vi "Final_Phase C_GND.vi"() -> ()   [LabVIEW 2014]
uses:
  <vilib>/DAQmx/create/channels.llb/DAQmx Create Channel (CO-Pulse Generation-Frequency).vi
  <vilib>/DAQmx/configure/timing.llb/DAQmx Timing (Implicit).vi
  <vilib>/DAQmx/write.llb/DAQmx Write (Counter Frequency 1Chan 1Samp).vi
  <vilib>/DAQmx/create/channels.llb/DAQmx Create Channel (DO-Digital Output).vi
  <vilib>/DAQmx/write.llb/DAQmx Write (Digital Bool 1Line 1Point).vi
  <vilib>/express/express arith-compare/Formula/XNode/ExpressFormulaBlockNode.xnode
panel:
  in  "Duration":dbl
  out "SB Elapsed Time (s)":dbl caption="Elapsed Time (s)"
  in  "frequency":dbl=1.0 format="%_6g"
  in  "Resistor Values in Ohms":string(combo)
  out "resis bank Numeric":dbl
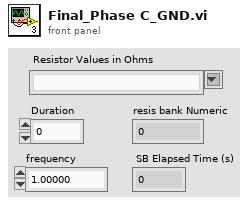
[diagram p1: front panel]
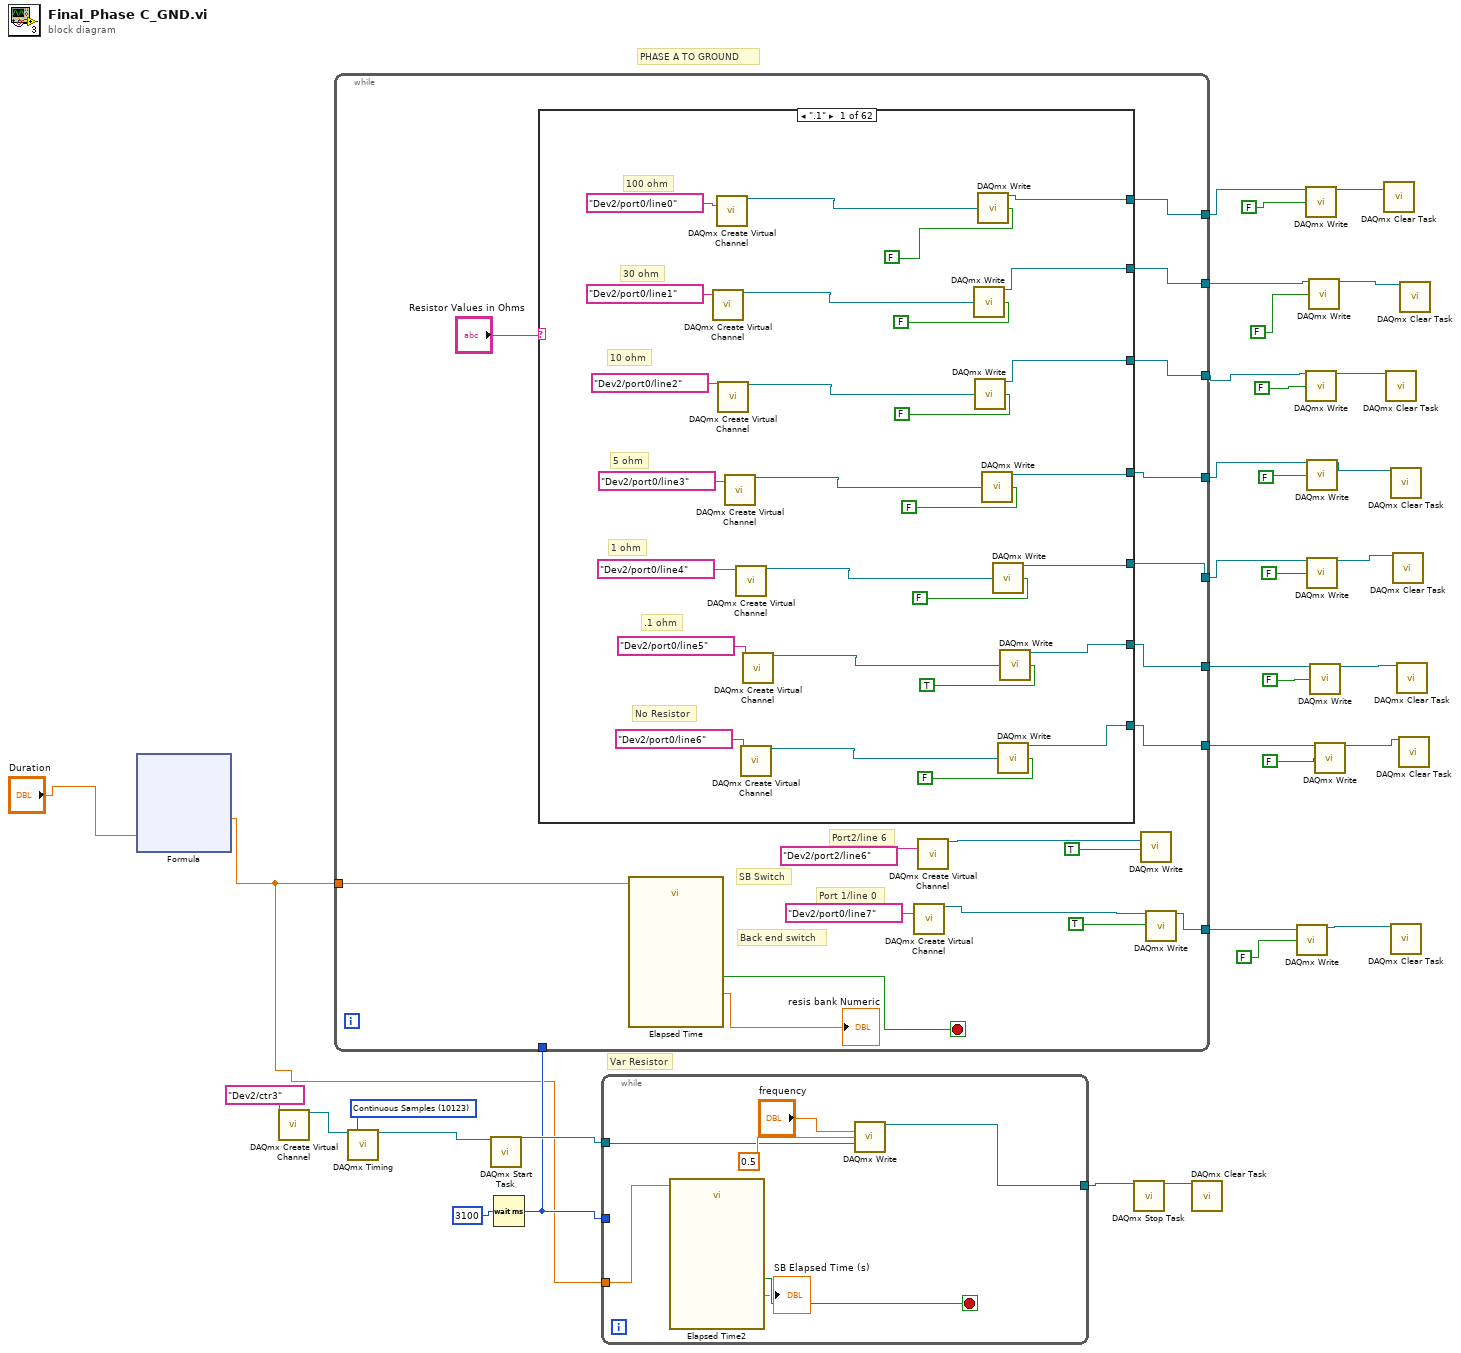
[diagram p0: block diagram]
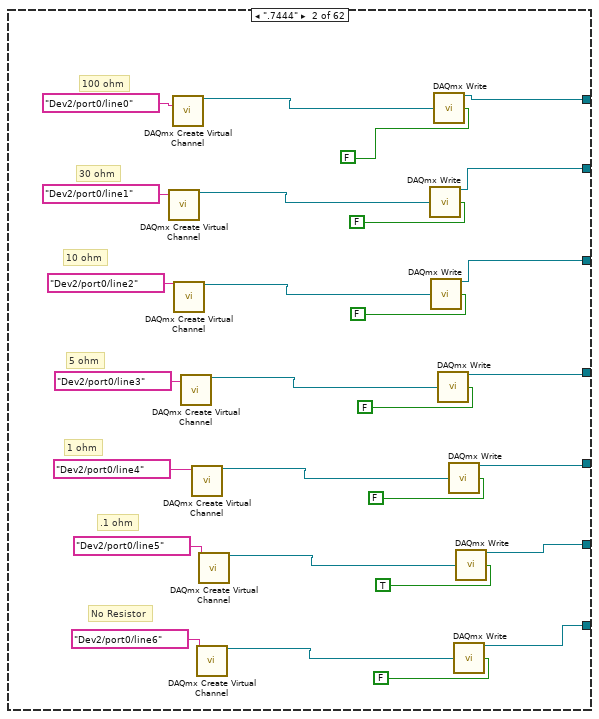
[diagram p2: hidden frame]
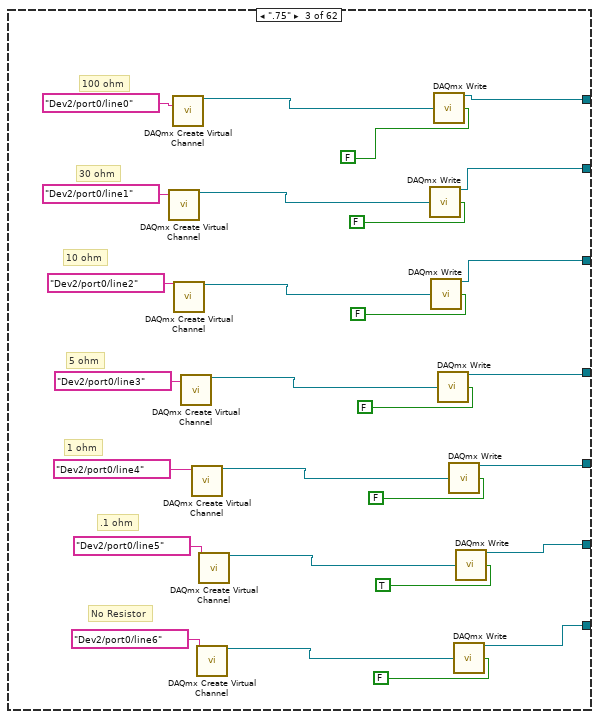
[diagram p3: hidden frame]
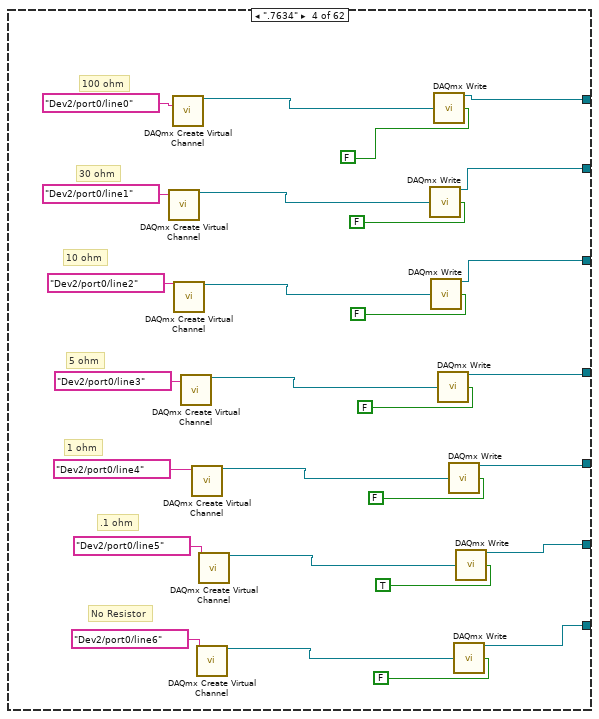
[diagram p4: hidden frame]
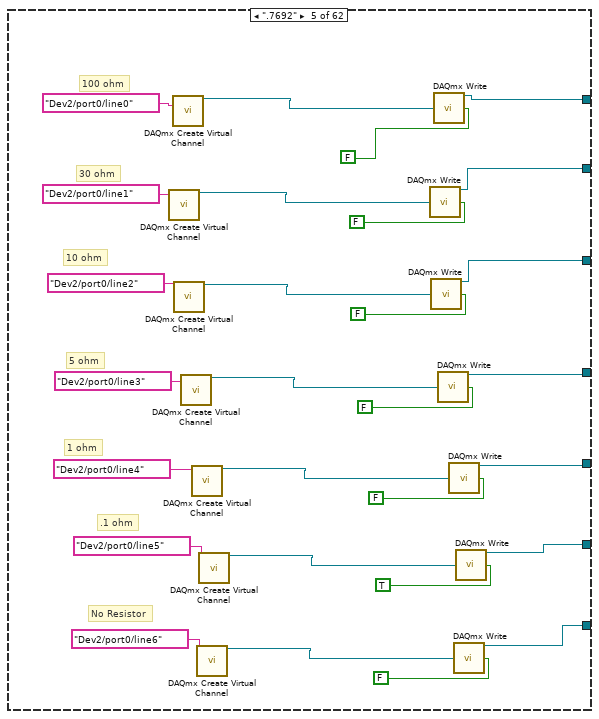
[diagram p5: hidden frame]
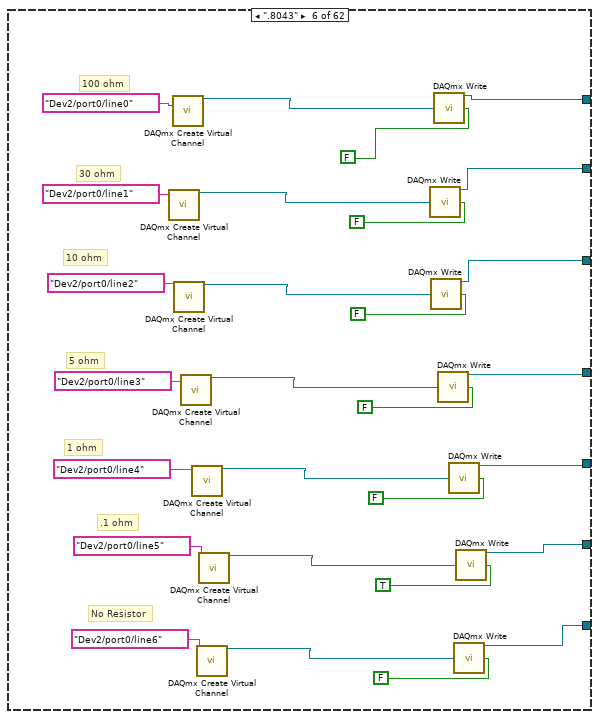
[diagram p6: hidden frame]
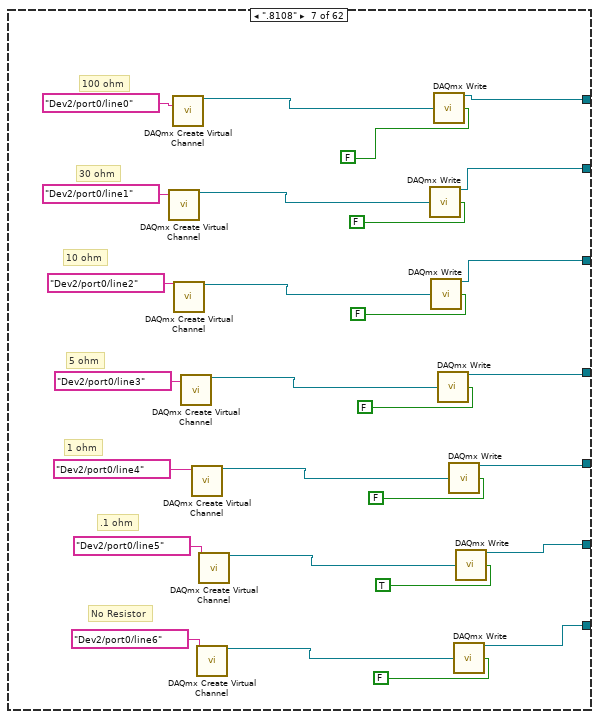
[diagram p7: hidden frame]
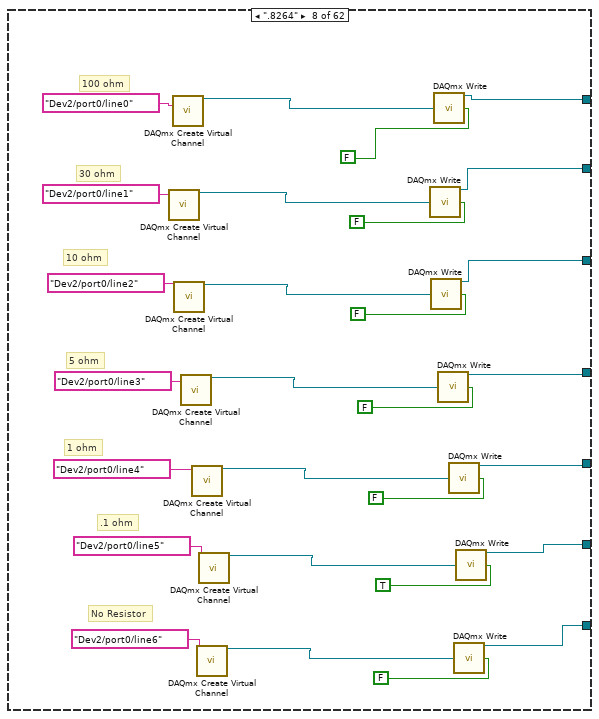
[diagram p8: hidden frame]
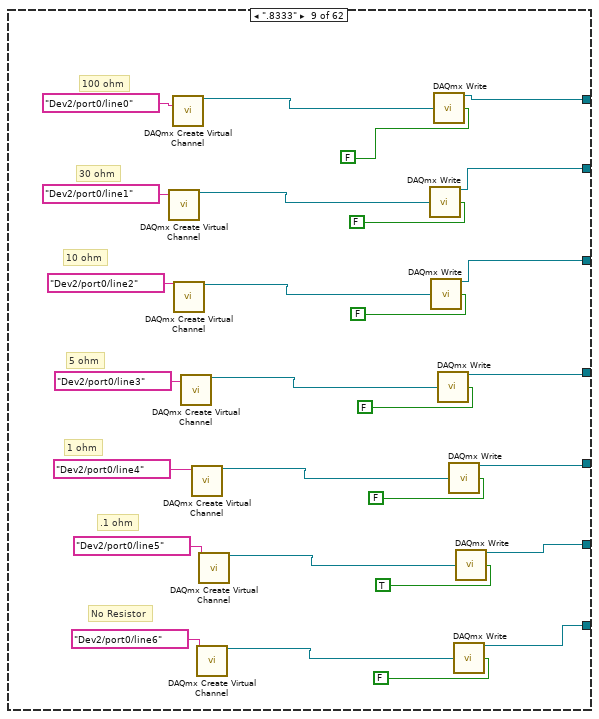
[diagram p9: hidden frame]
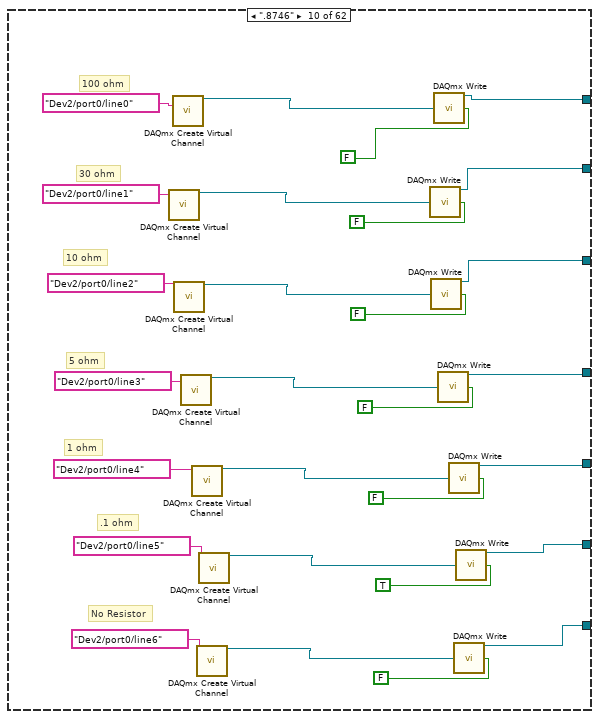
[diagram p10: hidden frame]
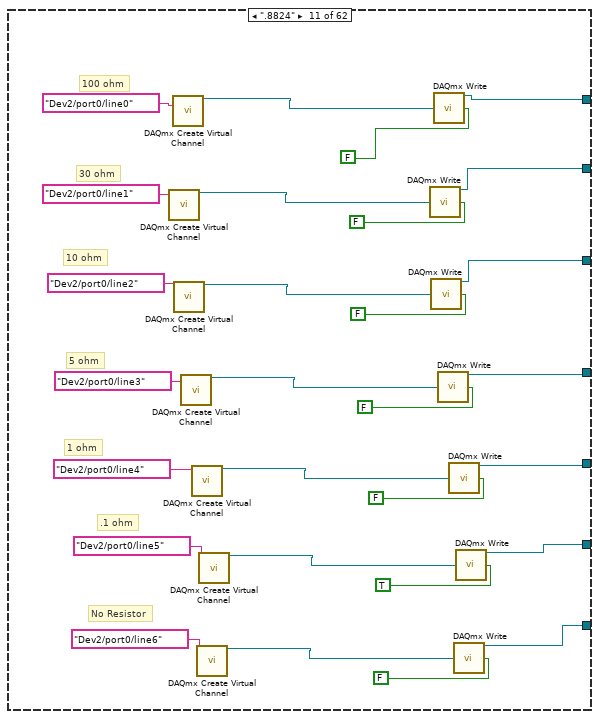
[diagram p11: hidden frame]
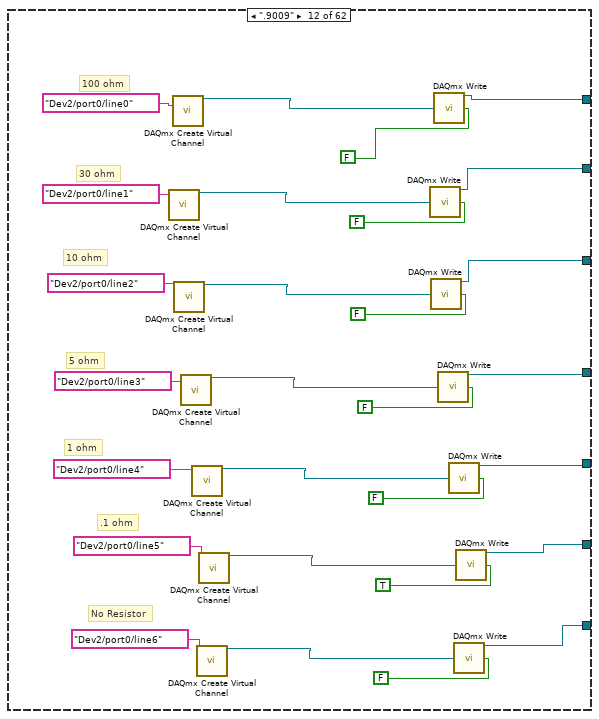
[diagram p12: hidden frame]
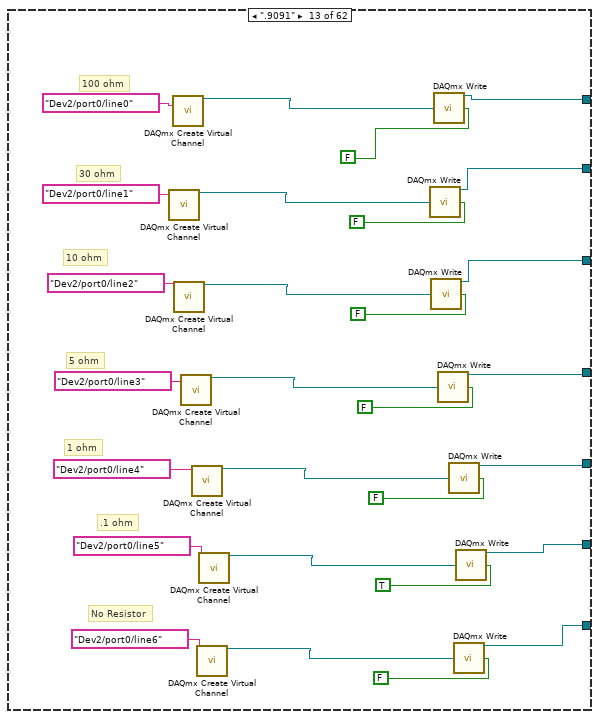
[diagram p13: hidden frame]
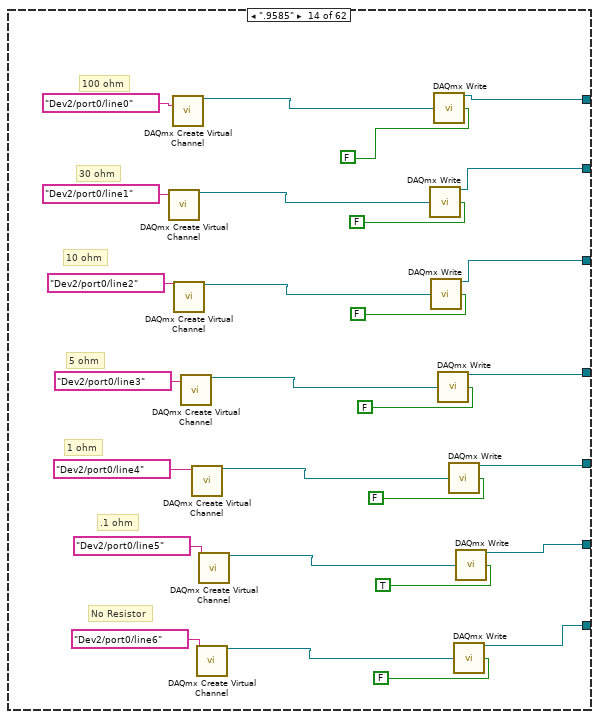
[diagram p14: hidden frame]
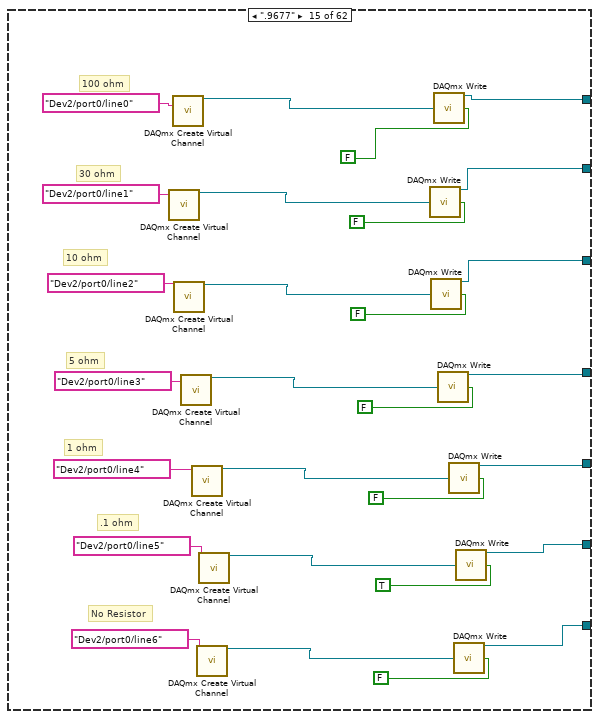
[diagram p15: hidden frame]
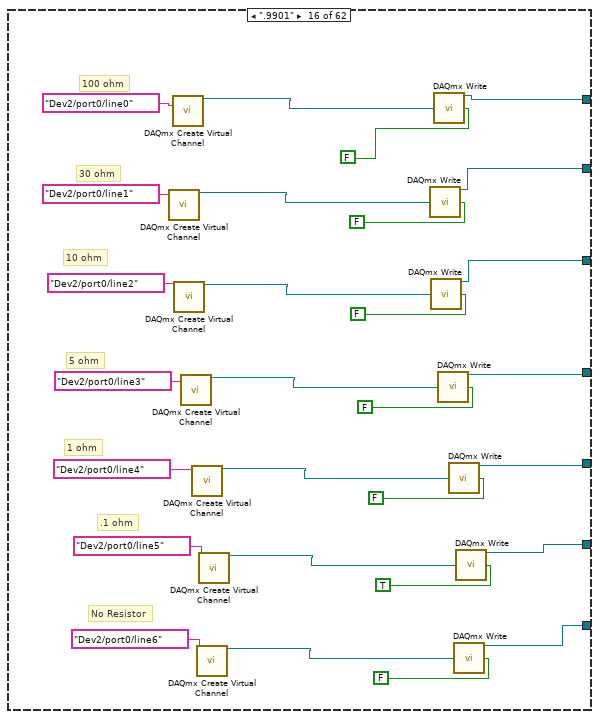
[diagram p16: hidden frame]
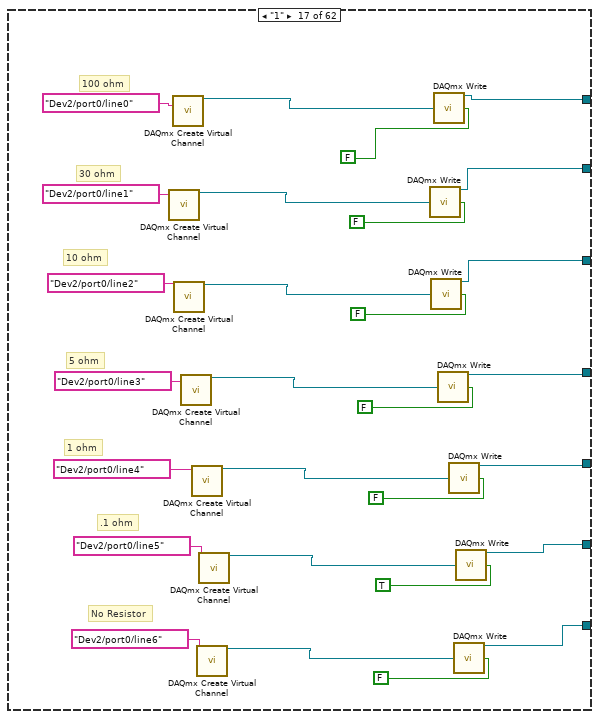
[diagram p17: hidden frame]
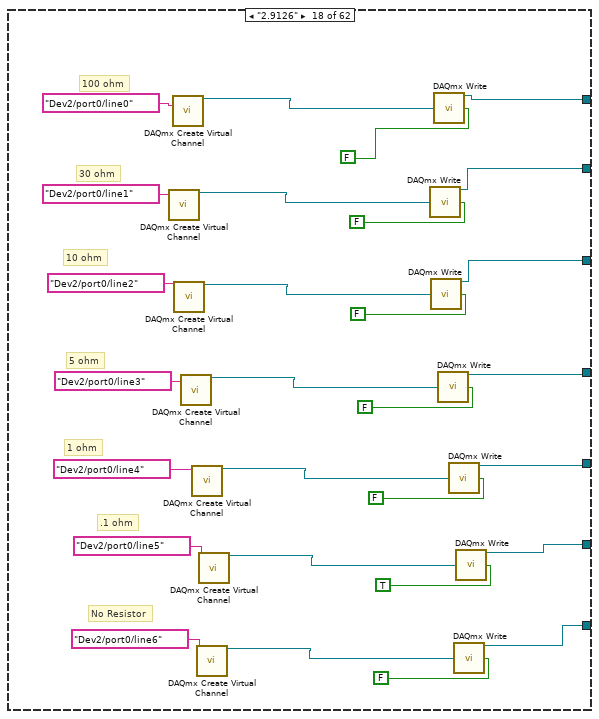
[diagram p18: hidden frame]
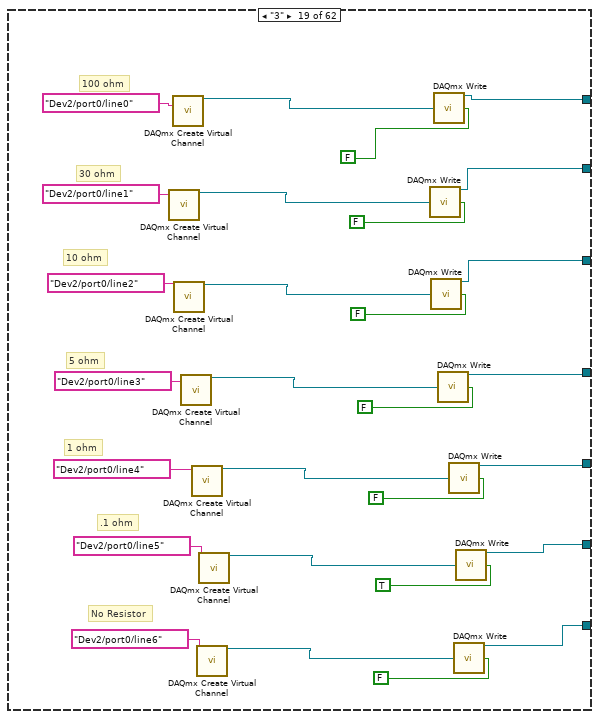
[diagram p19: hidden frame]
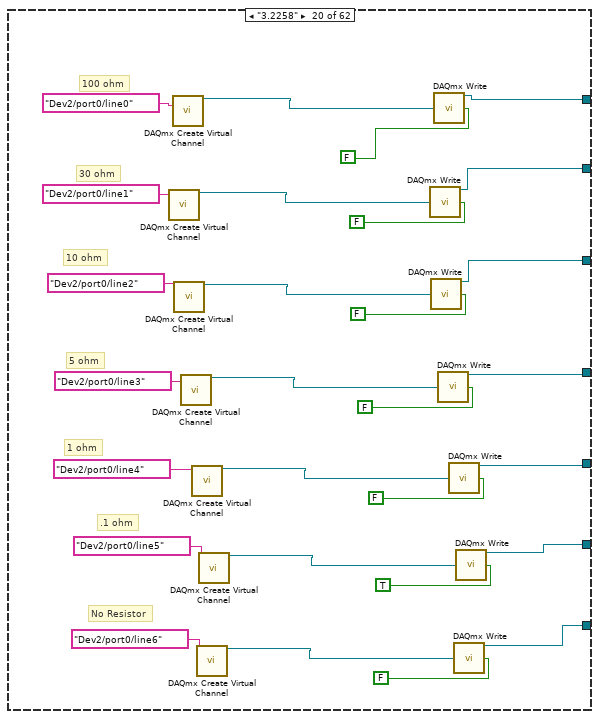
[diagram p20: hidden frame]
diagram:
  w7 = 10123 items=["Finite Samples"=10178, "Continuous Samples"=10123, "Hardware Timed Single Point"=12522] ("sample mode")
  # "Var Resistor"
  # "PHASE A TO GROUND"
  n1 = xnode "Formula"("X"="Duration") -> ("Result"=w4:dbl)  [unwired: 1 in, 1 out]
  n2 = call-poly <vilib>:"DAQmx Create Virtual Channel.vi"("counter"=tag "Dev2/ctr3" ("Counter(s)")) -> ("task out"=w8:refnum<k21>)  [unwired: 8 in, 6 out]
  n3 = call-poly <vilib>:"DAQmx Timing.vi"("task/channels in"=w8, "sample mode"=w7) -> ("task out"=w9:refnum<k21>)  [unwired: 3 in, 10 out]
  n4 = call <vilib>:"DAQmx Start Task.vi"("task/channels in"=w9) -> ("task out"=w6:refnum<k21>)  [unwired: 1 in, 13 out]
  n5 = Wait (ms)(milliseconds to wait=u32 3100) -> (millisecond timer value=w5:u32)
  n6 = while {
    tunnel: [w47] -> w12
    tunnel: [w46] -> w19
    tunnel: [w45] -> w18
    tunnel: [w44] -> w17
    tunnel: [w43] -> w16
    tunnel: [w42] -> w15
    tunnel: [w41] -> w14
    tunnel: [w40] -> w13
    tunnel: w5 -> [_]
    tunnel: w4 -> [w36]
    stop <- w37 stop-if-true
    # "Port 1/line 0"
    # "Port2/line 6"
    # "SB Switch"
    # "Back end switch"
    n7 = case shown="\".1\"" "Resistor Values in Ohms" {
      tunnel: [w63 w91 w119 w147 w175 w203 w231 w259 w287 w315 w343 w371 w399 w427 w455 w483 w511 w539 w567 w595 w623 w651 w679 w707 w735 w763 w791 w819 w847 w875 w903 w931 w959 w987 w1015 w1043 w1071 w1099 w1127 w1155 w1183 w1211 w1239 w1267 w1295 w1323 w1351 w1379 w1407 w1435 w1463 w1491 w1519 w1547 w1575 w1603 w1631 w1659 w1687 w1715 w1743 w1771] -> w46
      tunnel: [w62 w90 w118 w146 w174 w202 w230 w258 w286 w314 w342 w370 w398 w426 w454 w482 w510 w538 w566 w594 w622 w650 w678 w706 w734 w762 w790 w818 w846 w874 w902 w930 w958 w986 w1014 w1042 w1070 w1098 w1126 w1154 w1182 w1210 w1238 w1266 w1294 w1322 w1350 w1378 w1406 w1434 w1462 w1490 w1518 w1546 w1574 w1602 w1630 w1658 w1686 w1714 w1742 w1770] -> w45
      tunnel: [w60 w88 w116 w144 w172 w200 w228 w256 w284 w312 w340 w368 w396 w424 w452 w480 w508 w536 w564 w592 w620 w648 w676 w704 w732 w760 w788 w816 w844 w872 w900 w928 w956 w984 w1012 w1040 w1068 w1096 w1124 w1152 w1180 w1208 w1236 w1264 w1292 w1320 w1348 w1376 w1404 w1432 w1460 w1488 w1516 w1544 w1572 w1600 w1628 w1656 w1684 w1712 w1740 w1768] -> w43
      tunnel: [w59 w87 w115 w143 w171 w199 w227 w255 w283 w311 w339 w367 w395 w423 w451 w479 w507 w535 w563 w591 w619 w647 w675 w703 w731 w759 w787 w815 w843 w871 w899 w927 w955 w983 w1011 w1039 w1067 w1095 w1123 w1151 w1179 w1207 w1235 w1263 w1291 w1319 w1347 w1375 w1403 w1431 w1459 w1487 w1515 w1543 w1571 w1599 w1627 w1655 w1683 w1711 w1739 w1767] -> w42
      tunnel: [w58 w86 w114 w142 w170 w198 w226 w254 w282 w310 w338 w366 w394 w422 w450 w478 w506 w534 w562 w590 w618 w646 w674 w702 w730 w758 w786 w814 w842 w870 w898 w926 w954 w982 w1010 w1038 w1066 w1094 w1122 w1150 w1178 w1206 w1234 w1262 w1290 w1318 w1346 w1374 w1402 w1430 w1458 w1486 w1514 w1542 w1570 w1598 w1626 w1654 w1682 w1710 w1738 w1766] -> w41
      tunnel: [w54 w82 w110 w138 w166 w194 w222 w250 w278 w306 w334 w362 w390 w418 w446 w474 w502 w530 w558 w586 w614 w642 w670 w698 w726 w754 w782 w810 w838 w866 w894 w922 w950 w978 w1006 w1034 w1062 w1090 w1118 w1146 w1174 w1202 w1230 w1258 w1286 w1314 w1342 w1370 w1398 w1426 w1454 w1482 w1510 w1538 w1566 w1594 w1622 w1650 w1678 w1706 w1734 w1762] -> w40
      tunnel: [w61 w89 w117 w145 w173 w201 w229 w257 w285 w313 w341 w369 w397 w425 w453 w481 w509 w537 w565 w593 w621 w649 w677 w705 w733 w761 w789 w817 w845 w873 w901 w929 w957 w985 w1013 w1041 w1069 w1097 w1125 w1153 w1181 w1209 w1237 w1265 w1293 w1321 w1349 w1377 w1405 w1433 w1461 w1489 w1517 w1545 w1573 w1601 w1629 w1657 w1685 w1713 w1741 w1769] -> w44
      frame ".1" {
        # "No Resistor"
        # "30 ohm"
        # ".1 ohm"
        # "1 ohm"
        # "5 ohm"
        # "10 ohm"
        # "100 ohm"
        n8 = call-poly <vilib>:"DAQmx Create Virtual Channel.vi"("lines"=tag "Dev2/port0/line1") -> ("task out"=w68:refnum<k21>)  [unwired: 13 in, 1 out]
        n9 = call-poly <vilib>:"DAQmx Create Virtual Channel.vi"("lines"=tag "Dev2/port0/line0") -> ("task out"=w69:refnum<k21>)  [unwired: 13 in, 1 out]
        n10 = call-poly <vilib>:"DAQmx Create Virtual Channel.vi"("lines"=tag "Dev2/port0/line2") -> ("task out"=w67:refnum<k21>)  [unwired: 13 in, 1 out]
        n11 = call-poly <vilib>:"DAQmx Create Virtual Channel.vi"("lines"=tag "Dev2/port0/line3") -> ("task out"=w66:refnum<k21>)  [unwired: 13 in, 1 out]
        n12 = call-poly <vilib>:"DAQmx Create Virtual Channel.vi"("lines"=tag "Dev2/port0/line4") -> ("task out"=w65:refnum<k21>)  [unwired: 13 in, 1 out]
        n13 = call-poly <vilib>:"DAQmx Create Virtual Channel.vi"("lines"=tag "Dev2/port0/line6") -> ("task out"=w57:refnum<k21>)  [unwired: 13 in, 1 out]
        n14 = call-poly <vilib>:"DAQmx Create Virtual Channel.vi"("lines"=tag "Dev2/port0/line5") -> ("task out"=w64:refnum<k21>)  [unwired: 13 in, 1 out]
        n15 = call-poly <vilib>:"DAQmx Write.vi"("task/channels in"=w68, "data"=FALSE) -> ("task out"=w62:refnum<k21>)  [unwired: 11 in, 2 out]
        n16 = call-poly <vilib>:"DAQmx Write.vi"("task/channels in"=w67, "data"=FALSE) -> ("task out"=w61:refnum<k21>)  [unwired: 11 in, 2 out]
        n17 = call-poly <vilib>:"DAQmx Write.vi"("task/channels in"=w69, "data"=FALSE) -> ("task out"=w63:refnum<k21>)  [unwired: 11 in, 2 out]
        n18 = call-poly <vilib>:"DAQmx Write.vi"("task/channels in"=w66, "data"=FALSE) -> ("task out"=w60:refnum<k21>)  [unwired: 11 in, 2 out]
        n19 = call-poly <vilib>:"DAQmx Write.vi"("task/channels in"=w65, "data"=FALSE) -> ("task out"=w59:refnum<k21>)  [unwired: 11 in, 2 out]
        n20 = call-poly <vilib>:"DAQmx Write.vi"("task/channels in"=w57, "data"=FALSE) -> ("task out"=w54:refnum<k21>)  [unwired: 11 in, 2 out]
        n21 = call-poly <vilib>:"DAQmx Write.vi"("task/channels in"=w64, "data"=TRUE) -> ("task out"=w58:refnum<k21>)  [unwired: 11 in, 2 out]
      }
      frame ".7444" {
        # "No Resistor"
        # "30 ohm"
        # ".1 ohm"
        # "1 ohm"
        # "5 ohm"
        # "10 ohm"
        # "100 ohm"
        n22 = call-poly <vilib>:"DAQmx Create Virtual Channel.vi"("lines"=tag "Dev2/port0/line1") -> ("task out"=w96:refnum<k21>)  [unwired: 13 in, 1 out]
        n23 = call-poly <vilib>:"DAQmx Create Virtual Channel.vi"("lines"=tag "Dev2/port0/line0") -> ("task out"=w97:refnum<k21>)  [unwired: 13 in, 1 out]
        n24 = call-poly <vilib>:"DAQmx Create Virtual Channel.vi"("lines"=tag "Dev2/port0/line2") -> ("task out"=w95:refnum<k21>)  [unwired: 13 in, 1 out]
        n25 = call-poly <vilib>:"DAQmx Create Virtual Channel.vi"("lines"=tag "Dev2/port0/line3") -> ("task out"=w94:refnum<k21>)  [unwired: 13 in, 1 out]
        n26 = call-poly <vilib>:"DAQmx Create Virtual Channel.vi"("lines"=tag "Dev2/port0/line4") -> ("task out"=w93:refnum<k21>)  [unwired: 13 in, 1 out]
        n27 = call-poly <vilib>:"DAQmx Create Virtual Channel.vi"("lines"=tag "Dev2/port0/line6") -> ("task out"=w85:refnum<k21>)  [unwired: 13 in, 1 out]
        n28 = call-poly <vilib>:"DAQmx Create Virtual Channel.vi"("lines"=tag "Dev2/port0/line5") -> ("task out"=w92:refnum<k21>)  [unwired: 13 in, 1 out]
        n29 = call-poly <vilib>:"DAQmx Write.vi"("task/channels in"=w96, "data"=FALSE) -> ("task out"=w90:refnum<k21>)  [unwired: 11 in, 2 out]
        n30 = call-poly <vilib>:"DAQmx Write.vi"("task/channels in"=w95, "data"=FALSE) -> ("task out"=w89:refnum<k21>)  [unwired: 11 in, 2 out]
        n31 = call-poly <vilib>:"DAQmx Write.vi"("task/channels in"=w97, "data"=FALSE) -> ("task out"=w91:refnum<k21>)  [unwired: 11 in, 2 out]
        n32 = call-poly <vilib>:"DAQmx Write.vi"("task/channels in"=w94, "data"=FALSE) -> ("task out"=w88:refnum<k21>)  [unwired: 11 in, 2 out]
        n33 = call-poly <vilib>:"DAQmx Write.vi"("task/channels in"=w93, "data"=FALSE) -> ("task out"=w87:refnum<k21>)  [unwired: 11 in, 2 out]
        n34 = call-poly <vilib>:"DAQmx Write.vi"("task/channels in"=w85, "data"=FALSE) -> ("task out"=w82:refnum<k21>)  [unwired: 11 in, 2 out]
        n35 = call-poly <vilib>:"DAQmx Write.vi"("task/channels in"=w92, "data"=TRUE) -> ("task out"=w86:refnum<k21>)  [unwired: 11 in, 2 out]
      }
      frame ".75" {
        # "No Resistor"
        # "30 ohm"
        # ".1 ohm"
        # "1 ohm"
        # "5 ohm"
        # "10 ohm"
        # "100 ohm"
        n36 = call-poly <vilib>:"DAQmx Create Virtual Channel.vi"("lines"=tag "Dev2/port0/line1") -> ("task out"=w124:refnum<k21>)  [unwired: 13 in, 1 out]
        n37 = call-poly <vilib>:"DAQmx Create Virtual Channel.vi"("lines"=tag "Dev2/port0/line0") -> ("task out"=w125:refnum<k21>)  [unwired: 13 in, 1 out]
        n38 = call-poly <vilib>:"DAQmx Create Virtual Channel.vi"("lines"=tag "Dev2/port0/line2") -> ("task out"=w123:refnum<k21>)  [unwired: 13 in, 1 out]
        n39 = call-poly <vilib>:"DAQmx Create Virtual Channel.vi"("lines"=tag "Dev2/port0/line3") -> ("task out"=w122:refnum<k21>)  [unwired: 13 in, 1 out]
        n40 = call-poly <vilib>:"DAQmx Create Virtual Channel.vi"("lines"=tag "Dev2/port0/line4") -> ("task out"=w121:refnum<k21>)  [unwired: 13 in, 1 out]
        n41 = call-poly <vilib>:"DAQmx Create Virtual Channel.vi"("lines"=tag "Dev2/port0/line6") -> ("task out"=w113:refnum<k21>)  [unwired: 13 in, 1 out]
        n42 = call-poly <vilib>:"DAQmx Create Virtual Channel.vi"("lines"=tag "Dev2/port0/line5") -> ("task out"=w120:refnum<k21>)  [unwired: 13 in, 1 out]
        n43 = call-poly <vilib>:"DAQmx Write.vi"("task/channels in"=w124, "data"=FALSE) -> ("task out"=w118:refnum<k21>)  [unwired: 11 in, 2 out]
        n44 = call-poly <vilib>:"DAQmx Write.vi"("task/channels in"=w123, "data"=FALSE) -> ("task out"=w117:refnum<k21>)  [unwired: 11 in, 2 out]
        n45 = call-poly <vilib>:"DAQmx Write.vi"("task/channels in"=w125, "data"=FALSE) -> ("task out"=w119:refnum<k21>)  [unwired: 11 in, 2 out]
        n46 = call-poly <vilib>:"DAQmx Write.vi"("task/channels in"=w122, "data"=FALSE) -> ("task out"=w116:refnum<k21>)  [unwired: 11 in, 2 out]
        n47 = call-poly <vilib>:"DAQmx Write.vi"("task/channels in"=w121, "data"=FALSE) -> ("task out"=w115:refnum<k21>)  [unwired: 11 in, 2 out]
        n48 = call-poly <vilib>:"DAQmx Write.vi"("task/channels in"=w113, "data"=FALSE) -> ("task out"=w110:refnum<k21>)  [unwired: 11 in, 2 out]
        n49 = call-poly <vilib>:"DAQmx Write.vi"("task/channels in"=w120, "data"=TRUE) -> ("task out"=w114:refnum<k21>)  [unwired: 11 in, 2 out]
      }
      frame ".7634" {
        # "No Resistor"
        # "30 ohm"
        # ".1 ohm"
        # "1 ohm"
        # "5 ohm"
        # "10 ohm"
        # "100 ohm"
        n50 = call-poly <vilib>:"DAQmx Create Virtual Channel.vi"("lines"=tag "Dev2/port0/line1") -> ("task out"=w152:refnum<k21>)  [unwired: 13 in, 1 out]
        n51 = call-poly <vilib>:"DAQmx Create Virtual Channel.vi"("lines"=tag "Dev2/port0/line0") -> ("task out"=w153:refnum<k21>)  [unwired: 13 in, 1 out]
        n52 = call-poly <vilib>:"DAQmx Create Virtual Channel.vi"("lines"=tag "Dev2/port0/line2") -> ("task out"=w151:refnum<k21>)  [unwired: 13 in, 1 out]
        n53 = call-poly <vilib>:"DAQmx Create Virtual Channel.vi"("lines"=tag "Dev2/port0/line3") -> ("task out"=w150:refnum<k21>)  [unwired: 13 in, 1 out]
        n54 = call-poly <vilib>:"DAQmx Create Virtual Channel.vi"("lines"=tag "Dev2/port0/line4") -> ("task out"=w149:refnum<k21>)  [unwired: 13 in, 1 out]
        n55 = call-poly <vilib>:"DAQmx Create Virtual Channel.vi"("lines"=tag "Dev2/port0/line6") -> ("task out"=w141:refnum<k21>)  [unwired: 13 in, 1 out]
        n56 = call-poly <vilib>:"DAQmx Create Virtual Channel.vi"("lines"=tag "Dev2/port0/line5") -> ("task out"=w148:refnum<k21>)  [unwired: 13 in, 1 out]
        n57 = call-poly <vilib>:"DAQmx Write.vi"("task/channels in"=w152, "data"=FALSE) -> ("task out"=w146:refnum<k21>)  [unwired: 11 in, 2 out]
        n58 = call-poly <vilib>:"DAQmx Write.vi"("task/channels in"=w151, "data"=FALSE) -> ("task out"=w145:refnum<k21>)  [unwired: 11 in, 2 out]
        n59 = call-poly <vilib>:"DAQmx Write.vi"("task/channels in"=w153, "data"=FALSE) -> ("task out"=w147:refnum<k21>)  [unwired: 11 in, 2 out]
        n60 = call-poly <vilib>:"DAQmx Write.vi"("task/channels in"=w150, "data"=FALSE) -> ("task out"=w144:refnum<k21>)  [unwired: 11 in, 2 out]
        n61 = call-poly <vilib>:"DAQmx Write.vi"("task/channels in"=w149, "data"=FALSE) -> ("task out"=w143:refnum<k21>)  [unwired: 11 in, 2 out]
        n62 = call-poly <vilib>:"DAQmx Write.vi"("task/channels in"=w141, "data"=FALSE) -> ("task out"=w138:refnum<k21>)  [unwired: 11 in, 2 out]
        n63 = call-poly <vilib>:"DAQmx Write.vi"("task/channels in"=w148, "data"=TRUE) -> ("task out"=w142:refnum<k21>)  [unwired: 11 in, 2 out]
      }
      frame ".7692" {
        # "No Resistor"
        # "30 ohm"
        # ".1 ohm"
        # "1 ohm"
        # "5 ohm"
        # "10 ohm"
        # "100 ohm"
        n64 = call-poly <vilib>:"DAQmx Create Virtual Channel.vi"("lines"=tag "Dev2/port0/line1") -> ("task out"=w180:refnum<k21>)  [unwired: 13 in, 1 out]
        n65 = call-poly <vilib>:"DAQmx Create Virtual Channel.vi"("lines"=tag "Dev2/port0/line0") -> ("task out"=w181:refnum<k21>)  [unwired: 13 in, 1 out]
        n66 = call-poly <vilib>:"DAQmx Create Virtual Channel.vi"("lines"=tag "Dev2/port0/line2") -> ("task out"=w179:refnum<k21>)  [unwired: 13 in, 1 out]
        n67 = call-poly <vilib>:"DAQmx Create Virtual Channel.vi"("lines"=tag "Dev2/port0/line3") -> ("task out"=w178:refnum<k21>)  [unwired: 13 in, 1 out]
        n68 = call-poly <vilib>:"DAQmx Create Virtual Channel.vi"("lines"=tag "Dev2/port0/line4") -> ("task out"=w177:refnum<k21>)  [unwired: 13 in, 1 out]
        n69 = call-poly <vilib>:"DAQmx Create Virtual Channel.vi"("lines"=tag "Dev2/port0/line6") -> ("task out"=w169:refnum<k21>)  [unwired: 13 in, 1 out]
        n70 = call-poly <vilib>:"DAQmx Create Virtual Channel.vi"("lines"=tag "Dev2/port0/line5") -> ("task out"=w176:refnum<k21>)  [unwired: 13 in, 1 out]
        n71 = call-poly <vilib>:"DAQmx Write.vi"("task/channels in"=w180, "data"=FALSE) -> ("task out"=w174:refnum<k21>)  [unwired: 11 in, 2 out]
        n72 = call-poly <vilib>:"DAQmx Write.vi"("task/channels in"=w179, "data"=FALSE) -> ("task out"=w173:refnum<k21>)  [unwired: 11 in, 2 out]
        n73 = call-poly <vilib>:"DAQmx Write.vi"("task/channels in"=w181, "data"=FALSE) -> ("task out"=w175:refnum<k21>)  [unwired: 11 in, 2 out]
        n74 = call-poly <vilib>:"DAQmx Write.vi"("task/channels in"=w178, "data"=FALSE) -> ("task out"=w172:refnum<k21>)  [unwired: 11 in, 2 out]
        n75 = call-poly <vilib>:"DAQmx Write.vi"("task/channels in"=w177, "data"=FALSE) -> ("task out"=w171:refnum<k21>)  [unwired: 11 in, 2 out]
        n76 = call-poly <vilib>:"DAQmx Write.vi"("task/channels in"=w169, "data"=FALSE) -> ("task out"=w166:refnum<k21>)  [unwired: 11 in, 2 out]
        n77 = call-poly <vilib>:"DAQmx Write.vi"("task/channels in"=w176, "data"=TRUE) -> ("task out"=w170:refnum<k21>)  [unwired: 11 in, 2 out]
      }
      frame ".8043" {
        # "No Resistor"
        # "30 ohm"
        # ".1 ohm"
        # "1 ohm"
        # "5 ohm"
        # "10 ohm"
        # "100 ohm"
        n78 = call-poly <vilib>:"DAQmx Create Virtual Channel.vi"("lines"=tag "Dev2/port0/line1") -> ("task out"=w208:refnum<k21>)  [unwired: 13 in, 1 out]
        n79 = call-poly <vilib>:"DAQmx Create Virtual Channel.vi"("lines"=tag "Dev2/port0/line0") -> ("task out"=w209:refnum<k21>)  [unwired: 13 in, 1 out]
        n80 = call-poly <vilib>:"DAQmx Create Virtual Channel.vi"("lines"=tag "Dev2/port0/line2") -> ("task out"=w207:refnum<k21>)  [unwired: 13 in, 1 out]
        n81 = call-poly <vilib>:"DAQmx Create Virtual Channel.vi"("lines"=tag "Dev2/port0/line3") -> ("task out"=w206:refnum<k21>)  [unwired: 13 in, 1 out]
        n82 = call-poly <vilib>:"DAQmx Create Virtual Channel.vi"("lines"=tag "Dev2/port0/line4") -> ("task out"=w205:refnum<k21>)  [unwired: 13 in, 1 out]
        n83 = call-poly <vilib>:"DAQmx Create Virtual Channel.vi"("lines"=tag "Dev2/port0/line6") -> ("task out"=w197:refnum<k21>)  [unwired: 13 in, 1 out]
        n84 = call-poly <vilib>:"DAQmx Create Virtual Channel.vi"("lines"=tag "Dev2/port0/line5") -> ("task out"=w204:refnum<k21>)  [unwired: 13 in, 1 out]
        n85 = call-poly <vilib>:"DAQmx Write.vi"("task/channels in"=w208, "data"=FALSE) -> ("task out"=w202:refnum<k21>)  [unwired: 11 in, 2 out]
        n86 = call-poly <vilib>:"DAQmx Write.vi"("task/channels in"=w207, "data"=FALSE) -> ("task out"=w201:refnum<k21>)  [unwired: 11 in, 2 out]
        n87 = call-poly <vilib>:"DAQmx Write.vi"("task/channels in"=w209, "data"=FALSE) -> ("task out"=w203:refnum<k21>)  [unwired: 11 in, 2 out]
        n88 = call-poly <vilib>:"DAQmx Write.vi"("task/channels in"=w206, "data"=FALSE) -> ("task out"=w200:refnum<k21>)  [unwired: 11 in, 2 out]
        n89 = call-poly <vilib>:"DAQmx Write.vi"("task/channels in"=w205, "data"=FALSE) -> ("task out"=w199:refnum<k21>)  [unwired: 11 in, 2 out]
        n90 = call-poly <vilib>:"DAQmx Write.vi"("task/channels in"=w197, "data"=FALSE) -> ("task out"=w194:refnum<k21>)  [unwired: 11 in, 2 out]
        n91 = call-poly <vilib>:"DAQmx Write.vi"("task/channels in"=w204, "data"=TRUE) -> ("task out"=w198:refnum<k21>)  [unwired: 11 in, 2 out]
      }
      frame ".8108" {
        # "No Resistor"
        # "30 ohm"
        # ".1 ohm"
        # "1 ohm"
        # "5 ohm"
        # "10 ohm"
        # "100 ohm"
        n92 = call-poly <vilib>:"DAQmx Create Virtual Channel.vi"("lines"=tag "Dev2/port0/line1") -> ("task out"=w236:refnum<k21>)  [unwired: 13 in, 1 out]
        n93 = call-poly <vilib>:"DAQmx Create Virtual Channel.vi"("lines"=tag "Dev2/port0/line0") -> ("task out"=w237:refnum<k21>)  [unwired: 13 in, 1 out]
        n94 = call-poly <vilib>:"DAQmx Create Virtual Channel.vi"("lines"=tag "Dev2/port0/line2") -> ("task out"=w235:refnum<k21>)  [unwired: 13 in, 1 out]
        n95 = call-poly <vilib>:"DAQmx Create Virtual Channel.vi"("lines"=tag "Dev2/port0/line3") -> ("task out"=w234:refnum<k21>)  [unwired: 13 in, 1 out]
        n96 = call-poly <vilib>:"DAQmx Create Virtual Channel.vi"("lines"=tag "Dev2/port0/line4") -> ("task out"=w233:refnum<k21>)  [unwired: 13 in, 1 out]
        n97 = call-poly <vilib>:"DAQmx Create Virtual Channel.vi"("lines"=tag "Dev2/port0/line6") -> ("task out"=w225:refnum<k21>)  [unwired: 13 in, 1 out]
        n98 = call-poly <vilib>:"DAQmx Create Virtual Channel.vi"("lines"=tag "Dev2/port0/line5") -> ("task out"=w232:refnum<k21>)  [unwired: 13 in, 1 out]
        n99 = call-poly <vilib>:"DAQmx Write.vi"("task/channels in"=w236, "data"=FALSE) -> ("task out"=w230:refnum<k21>)  [unwired: 11 in, 2 out]
        n100 = call-poly <vilib>:"DAQmx Write.vi"("task/channels in"=w235, "data"=FALSE) -> ("task out"=w229:refnum<k21>)  [unwired: 11 in, 2 out]
        n101 = call-poly <vilib>:"DAQmx Write.vi"("task/channels in"=w237, "data"=FALSE) -> ("task out"=w231:refnum<k21>)  [unwired: 11 in, 2 out]
        n102 = call-poly <vilib>:"DAQmx Write.vi"("task/channels in"=w234, "data"=FALSE) -> ("task out"=w228:refnum<k21>)  [unwired: 11 in, 2 out]
        n103 = call-poly <vilib>:"DAQmx Write.vi"("task/channels in"=w233, "data"=FALSE) -> ("task out"=w227:refnum<k21>)  [unwired: 11 in, 2 out]
        n104 = call-poly <vilib>:"DAQmx Write.vi"("task/channels in"=w225, "data"=FALSE) -> ("task out"=w222:refnum<k21>)  [unwired: 11 in, 2 out]
        n105 = call-poly <vilib>:"DAQmx Write.vi"("task/channels in"=w232, "data"=TRUE) -> ("task out"=w226:refnum<k21>)  [unwired: 11 in, 2 out]
      }
      frame ".8264" {
        # "No Resistor"
        # "30 ohm"
        # ".1 ohm"
        # "1 ohm"
        # "5 ohm"
        # "10 ohm"
        # "100 ohm"
        n106 = call-poly <vilib>:"DAQmx Create Virtual Channel.vi"("lines"=tag "Dev2/port0/line1") -> ("task out"=w264:refnum<k21>)  [unwired: 13 in, 1 out]
        n107 = call-poly <vilib>:"DAQmx Create Virtual Channel.vi"("lines"=tag "Dev2/port0/line0") -> ("task out"=w265:refnum<k21>)  [unwired: 13 in, 1 out]
        n108 = call-poly <vilib>:"DAQmx Create Virtual Channel.vi"("lines"=tag "Dev2/port0/line2") -> ("task out"=w263:refnum<k21>)  [unwired: 13 in, 1 out]
        n109 = call-poly <vilib>:"DAQmx Create Virtual Channel.vi"("lines"=tag "Dev2/port0/line3") -> ("task out"=w262:refnum<k21>)  [unwired: 13 in, 1 out]
        n110 = call-poly <vilib>:"DAQmx Create Virtual Channel.vi"("lines"=tag "Dev2/port0/line4") -> ("task out"=w261:refnum<k21>)  [unwired: 13 in, 1 out]
        n111 = call-poly <vilib>:"DAQmx Create Virtual Channel.vi"("lines"=tag "Dev2/port0/line6") -> ("task out"=w253:refnum<k21>)  [unwired: 13 in, 1 out]
        n112 = call-poly <vilib>:"DAQmx Create Virtual Channel.vi"("lines"=tag "Dev2/port0/line5") -> ("task out"=w260:refnum<k21>)  [unwired: 13 in, 1 out]
        n113 = call-poly <vilib>:"DAQmx Write.vi"("task/channels in"=w264, "data"=FALSE) -> ("task out"=w258:refnum<k21>)  [unwired: 11 in, 2 out]
        n114 = call-poly <vilib>:"DAQmx Write.vi"("task/channels in"=w263, "data"=FALSE) -> ("task out"=w257:refnum<k21>)  [unwired: 11 in, 2 out]
        n115 = call-poly <vilib>:"DAQmx Write.vi"("task/channels in"=w265, "data"=FALSE) -> ("task out"=w259:refnum<k21>)  [unwired: 11 in, 2 out]
        n116 = call-poly <vilib>:"DAQmx Write.vi"("task/channels in"=w262, "data"=FALSE) -> ("task out"=w256:refnum<k21>)  [unwired: 11 in, 2 out]
        n117 = call-poly <vilib>:"DAQmx Write.vi"("task/channels in"=w261, "data"=FALSE) -> ("task out"=w255:refnum<k21>)  [unwired: 11 in, 2 out]
        n118 = call-poly <vilib>:"DAQmx Write.vi"("task/channels in"=w253, "data"=FALSE) -> ("task out"=w250:refnum<k21>)  [unwired: 11 in, 2 out]
        n119 = call-poly <vilib>:"DAQmx Write.vi"("task/channels in"=w260, "data"=TRUE) -> ("task out"=w254:refnum<k21>)  [unwired: 11 in, 2 out]
      }
      frame ".8333" {
        # "No Resistor"
        # "30 ohm"
        # ".1 ohm"
        # "1 ohm"
        # "5 ohm"
        # "10 ohm"
        # "100 ohm"
        n120 = call-poly <vilib>:"DAQmx Create Virtual Channel.vi"("lines"=tag "Dev2/port0/line1") -> ("task out"=w292:refnum<k21>)  [unwired: 13 in, 1 out]
        n121 = call-poly <vilib>:"DAQmx Create Virtual Channel.vi"("lines"=tag "Dev2/port0/line0") -> ("task out"=w293:refnum<k21>)  [unwired: 13 in, 1 out]
        n122 = call-poly <vilib>:"DAQmx Create Virtual Channel.vi"("lines"=tag "Dev2/port0/line2") -> ("task out"=w291:refnum<k21>)  [unwired: 13 in, 1 out]
        n123 = call-poly <vilib>:"DAQmx Create Virtual Channel.vi"("lines"=tag "Dev2/port0/line3") -> ("task out"=w290:refnum<k21>)  [unwired: 13 in, 1 out]
        n124 = call-poly <vilib>:"DAQmx Create Virtual Channel.vi"("lines"=tag "Dev2/port0/line4") -> ("task out"=w289:refnum<k21>)  [unwired: 13 in, 1 out]
        n125 = call-poly <vilib>:"DAQmx Create Virtual Channel.vi"("lines"=tag "Dev2/port0/line6") -> ("task out"=w281:refnum<k21>)  [unwired: 13 in, 1 out]
        n126 = call-poly <vilib>:"DAQmx Create Virtual Channel.vi"("lines"=tag "Dev2/port0/line5") -> ("task out"=w288:refnum<k21>)  [unwired: 13 in, 1 out]
        n127 = call-poly <vilib>:"DAQmx Write.vi"("task/channels in"=w292, "data"=FALSE) -> ("task out"=w286:refnum<k21>)  [unwired: 11 in, 2 out]
        n128 = call-poly <vilib>:"DAQmx Write.vi"("task/channels in"=w291, "data"=FALSE) -> ("task out"=w285:refnum<k21>)  [unwired: 11 in, 2 out]
        n129 = call-poly <vilib>:"DAQmx Write.vi"("task/channels in"=w293, "data"=FALSE) -> ("task out"=w287:refnum<k21>)  [unwired: 11 in, 2 out]
        n130 = call-poly <vilib>:"DAQmx Write.vi"("task/channels in"=w290, "data"=FALSE) -> ("task out"=w284:refnum<k21>)  [unwired: 11 in, 2 out]
        n131 = call-poly <vilib>:"DAQmx Write.vi"("task/channels in"=w289, "data"=FALSE) -> ("task out"=w283:refnum<k21>)  [unwired: 11 in, 2 out]
        n132 = call-poly <vilib>:"DAQmx Write.vi"("task/channels in"=w281, "data"=FALSE) -> ("task out"=w278:refnum<k21>)  [unwired: 11 in, 2 out]
        n133 = call-poly <vilib>:"DAQmx Write.vi"("task/channels in"=w288, "data"=TRUE) -> ("task out"=w282:refnum<k21>)  [unwired: 11 in, 2 out]
      }
      frame ".8746" {
        # "No Resistor"
        # "30 ohm"
        # ".1 ohm"
        # "1 ohm"
        # "5 ohm"
        # "10 ohm"
        # "100 ohm"
        n134 = call-poly <vilib>:"DAQmx Create Virtual Channel.vi"("lines"=tag "Dev2/port0/line1") -> ("task out"=w320:refnum<k21>)  [unwired: 13 in, 1 out]
        n135 = call-poly <vilib>:"DAQmx Create Virtual Channel.vi"("lines"=tag "Dev2/port0/line0") -> ("task out"=w321:refnum<k21>)  [unwired: 13 in, 1 out]
        n136 = call-poly <vilib>:"DAQmx Create Virtual Channel.vi"("lines"=tag "Dev2/port0/line2") -> ("task out"=w319:refnum<k21>)  [unwired: 13 in, 1 out]
        n137 = call-poly <vilib>:"DAQmx Create Virtual Channel.vi"("lines"=tag "Dev2/port0/line3") -> ("task out"=w318:refnum<k21>)  [unwired: 13 in, 1 out]
        n138 = call-poly <vilib>:"DAQmx Create Virtual Channel.vi"("lines"=tag "Dev2/port0/line4") -> ("task out"=w317:refnum<k21>)  [unwired: 13 in, 1 out]
        n139 = call-poly <vilib>:"DAQmx Create Virtual Channel.vi"("lines"=tag "Dev2/port0/line6") -> ("task out"=w309:refnum<k21>)  [unwired: 13 in, 1 out]
        n140 = call-poly <vilib>:"DAQmx Create Virtual Channel.vi"("lines"=tag "Dev2/port0/line5") -> ("task out"=w316:refnum<k21>)  [unwired: 13 in, 1 out]
        n141 = call-poly <vilib>:"DAQmx Write.vi"("task/channels in"=w320, "data"=FALSE) -> ("task out"=w314:refnum<k21>)  [unwired: 11 in, 2 out]
        n142 = call-poly <vilib>:"DAQmx Write.vi"("task/channels in"=w319, "data"=FALSE) -> ("task out"=w313:refnum<k21>)  [unwired: 11 in, 2 out]
        n143 = call-poly <vilib>:"DAQmx Write.vi"("task/channels in"=w321, "data"=FALSE) -> ("task out"=w315:refnum<k21>)  [unwired: 11 in, 2 out]
        n144 = call-poly <vilib>:"DAQmx Write.vi"("task/channels in"=w318, "data"=FALSE) -> ("task out"=w312:refnum<k21>)  [unwired: 11 in, 2 out]
        n145 = call-poly <vilib>:"DAQmx Write.vi"("task/channels in"=w317, "data"=FALSE) -> ("task out"=w311:refnum<k21>)  [unwired: 11 in, 2 out]
        n146 = call-poly <vilib>:"DAQmx Write.vi"("task/channels in"=w309, "data"=FALSE) -> ("task out"=w306:refnum<k21>)  [unwired: 11 in, 2 out]
        n147 = call-poly <vilib>:"DAQmx Write.vi"("task/channels in"=w316, "data"=TRUE) -> ("task out"=w310:refnum<k21>)  [unwired: 11 in, 2 out]
      }
      frame ".8824" {
        # "No Resistor"
        # "30 ohm"
        # ".1 ohm"
        # "1 ohm"
        # "5 ohm"
        # "10 ohm"
        # "100 ohm"
        n148 = call-poly <vilib>:"DAQmx Create Virtual Channel.vi"("lines"=tag "Dev2/port0/line1") -> ("task out"=w348:refnum<k21>)  [unwired: 13 in, 1 out]
        n149 = call-poly <vilib>:"DAQmx Create Virtual Channel.vi"("lines"=tag "Dev2/port0/line0") -> ("task out"=w349:refnum<k21>)  [unwired: 13 in, 1 out]
        n150 = call-poly <vilib>:"DAQmx Create Virtual Channel.vi"("lines"=tag "Dev2/port0/line2") -> ("task out"=w347:refnum<k21>)  [unwired: 13 in, 1 out]
        n151 = call-poly <vilib>:"DAQmx Create Virtual Channel.vi"("lines"=tag "Dev2/port0/line3") -> ("task out"=w346:refnum<k21>)  [unwired: 13 in, 1 out]
        n152 = call-poly <vilib>:"DAQmx Create Virtual Channel.vi"("lines"=tag "Dev2/port0/line4") -> ("task out"=w345:refnum<k21>)  [unwired: 13 in, 1 out]
        n153 = call-poly <vilib>:"DAQmx Create Virtual Channel.vi"("lines"=tag "Dev2/port0/line6") -> ("task out"=w337:refnum<k21>)  [unwired: 13 in, 1 out]
        n154 = call-poly <vilib>:"DAQmx Create Virtual Channel.vi"("lines"=tag "Dev2/port0/line5") -> ("task out"=w344:refnum<k21>)  [unwired: 13 in, 1 out]
        n155 = call-poly <vilib>:"DAQmx Write.vi"("task/channels in"=w348, "data"=FALSE) -> ("task out"=w342:refnum<k21>)  [unwired: 11 in, 2 out]
        n156 = call-poly <vilib>:"DAQmx Write.vi"("task/channels in"=w347, "data"=FALSE) -> ("task out"=w341:refnum<k21>)  [unwired: 11 in, 2 out]
        n157 = call-poly <vilib>:"DAQmx Write.vi"("task/channels in"=w349, "data"=FALSE) -> ("task out"=w343:refnum<k21>)  [unwired: 11 in, 2 out]
        n158 = call-poly <vilib>:"DAQmx Write.vi"("task/channels in"=w346, "data"=FALSE) -> ("task out"=w340:refnum<k21>)  [unwired: 11 in, 2 out]
        n159 = call-poly <vilib>:"DAQmx Write.vi"("task/channels in"=w345, "data"=FALSE) -> ("task out"=w339:refnum<k21>)  [unwired: 11 in, 2 out]
        n160 = call-poly <vilib>:"DAQmx Write.vi"("task/channels in"=w337, "data"=FALSE) -> ("task out"=w334:refnum<k21>)  [unwired: 11 in, 2 out]
        n161 = call-poly <vilib>:"DAQmx Write.vi"("task/channels in"=w344, "data"=TRUE) -> ("task out"=w338:refnum<k21>)  [unwired: 11 in, 2 out]
      }
      frame ".9009" {
        # "No Resistor"
        # "30 ohm"
        # ".1 ohm"
        # "1 ohm"
        # "5 ohm"
        # "10 ohm"
        # "100 ohm"
        n162 = call-poly <vilib>:"DAQmx Create Virtual Channel.vi"("lines"=tag "Dev2/port0/line1") -> ("task out"=w376:refnum<k21>)  [unwired: 13 in, 1 out]
        n163 = call-poly <vilib>:"DAQmx Create Virtual Channel.vi"("lines"=tag "Dev2/port0/line0") -> ("task out"=w377:refnum<k21>)  [unwired: 13 in, 1 out]
        n164 = call-poly <vilib>:"DAQmx Create Virtual Channel.vi"("lines"=tag "Dev2/port0/line2") -> ("task out"=w375:refnum<k21>)  [unwired: 13 in, 1 out]
        n165 = call-poly <vilib>:"DAQmx Create Virtual Channel.vi"("lines"=tag "Dev2/port0/line3") -> ("task out"=w374:refnum<k21>)  [unwired: 13 in, 1 out]
        n166 = call-poly <vilib>:"DAQmx Create Virtual Channel.vi"("lines"=tag "Dev2/port0/line4") -> ("task out"=w373:refnum<k21>)  [unwired: 13 in, 1 out]
        n167 = call-poly <vilib>:"DAQmx Create Virtual Channel.vi"("lines"=tag "Dev2/port0/line6") -> ("task out"=w365:refnum<k21>)  [unwired: 13 in, 1 out]
        n168 = call-poly <vilib>:"DAQmx Create Virtual Channel.vi"("lines"=tag "Dev2/port0/line5") -> ("task out"=w372:refnum<k21>)  [unwired: 13 in, 1 out]
        n169 = call-poly <vilib>:"DAQmx Write.vi"("task/channels in"=w376, "data"=FALSE) -> ("task out"=w370:refnum<k21>)  [unwired: 11 in, 2 out]
        n170 = call-poly <vilib>:"DAQmx Write.vi"("task/channels in"=w375, "data"=FALSE) -> ("task out"=w369:refnum<k21>)  [unwired: 11 in, 2 out]
        n171 = call-poly <vilib>:"DAQmx Write.vi"("task/channels in"=w377, "data"=FALSE) -> ("task out"=w371:refnum<k21>)  [unwired: 11 in, 2 out]
        n172 = call-poly <vilib>:"DAQmx Write.vi"("task/channels in"=w374, "data"=FALSE) -> ("task out"=w368:refnum<k21>)  [unwired: 11 in, 2 out]
        n173 = call-poly <vilib>:"DAQmx Write.vi"("task/channels in"=w373, "data"=FALSE) -> ("task out"=w367:refnum<k21>)  [unwired: 11 in, 2 out]
        n174 = call-poly <vilib>:"DAQmx Write.vi"("task/channels in"=w365, "data"=FALSE) -> ("task out"=w362:refnum<k21>)  [unwired: 11 in, 2 out]
        n175 = call-poly <vilib>:"DAQmx Write.vi"("task/channels in"=w372, "data"=TRUE) -> ("task out"=w366:refnum<k21>)  [unwired: 11 in, 2 out]
      }
      frame ".9091" {
        # "No Resistor"
        # "30 ohm"
        # ".1 ohm"
        # "1 ohm"
        # "5 ohm"
        # "10 ohm"
        # "100 ohm"
        n176 = call-poly <vilib>:"DAQmx Create Virtual Channel.vi"("lines"=tag "Dev2/port0/line1") -> ("task out"=w404:refnum<k21>)  [unwired: 13 in, 1 out]
        n177 = call-poly <vilib>:"DAQmx Create Virtual Channel.vi"("lines"=tag "Dev2/port0/line0") -> ("task out"=w405:refnum<k21>)  [unwired: 13 in, 1 out]
        n178 = call-poly <vilib>:"DAQmx Create Virtual Channel.vi"("lines"=tag "Dev2/port0/line2") -> ("task out"=w403:refnum<k21>)  [unwired: 13 in, 1 out]
        n179 = call-poly <vilib>:"DAQmx Create Virtual Channel.vi"("lines"=tag "Dev2/port0/line3") -> ("task out"=w402:refnum<k21>)  [unwired: 13 in, 1 out]
        n180 = call-poly <vilib>:"DAQmx Create Virtual Channel.vi"("lines"=tag "Dev2/port0/line4") -> ("task out"=w401:refnum<k21>)  [unwired: 13 in, 1 out]
        n181 = call-poly <vilib>:"DAQmx Create Virtual Channel.vi"("lines"=tag "Dev2/port0/line6") -> ("task out"=w393:refnum<k21>)  [unwired: 13 in, 1 out]
        n182 = call-poly <vilib>:"DAQmx Create Virtual Channel.vi"("lines"=tag "Dev2/port0/line5") -> ("task out"=w400:refnum<k21>)  [unwired: 13 in, 1 out]
        n183 = call-poly <vilib>:"DAQmx Write.vi"("task/channels in"=w404, "data"=FALSE) -> ("task out"=w398:refnum<k21>)  [unwired: 11 in, 2 out]
        n184 = call-poly <vilib>:"DAQmx Write.vi"("task/channels in"=w403, "data"=FALSE) -> ("task out"=w397:refnum<k21>)  [unwired: 11 in, 2 out]
        n185 = call-poly <vilib>:"DAQmx Write.vi"("task/channels in"=w405, "data"=FALSE) -> ("task out"=w399:refnum<k21>)  [unwired: 11 in, 2 out]
        n186 = call-poly <vilib>:"DAQmx Write.vi"("task/channels in"=w402, "data"=FALSE) -> ("task out"=w396:refnum<k21>)  [unwired: 11 in, 2 out]
        n187 = call-poly <vilib>:"DAQmx Write.vi"("task/channels in"=w401, "data"=FALSE) -> ("task out"=w395:refnum<k21>)  [unwired: 11 in, 2 out]
        n188 = call-poly <vilib>:"DAQmx Write.vi"("task/channels in"=w393, "data"=FALSE) -> ("task out"=w390:refnum<k21>)  [unwired: 11 in, 2 out]
        n189 = call-poly <vilib>:"DAQmx Write.vi"("task/channels in"=w400, "data"=TRUE) -> ("task out"=w394:refnum<k21>)  [unwired: 11 in, 2 out]
      }
      frame ".9585" {
        # "No Resistor"
        # "30 ohm"
        # ".1 ohm"
        # "1 ohm"
        # "5 ohm"
        # "10 ohm"
        # "100 ohm"
        n190 = call-poly <vilib>:"DAQmx Create Virtual Channel.vi"("lines"=tag "Dev2/port0/line1") -> ("task out"=w432:refnum<k21>)  [unwired: 13 in, 1 out]
        n191 = call-poly <vilib>:"DAQmx Create Virtual Channel.vi"("lines"=tag "Dev2/port0/line0") -> ("task out"=w433:refnum<k21>)  [unwired: 13 in, 1 out]
        n192 = call-poly <vilib>:"DAQmx Create Virtual Channel.vi"("lines"=tag "Dev2/port0/line2") -> ("task out"=w431:refnum<k21>)  [unwired: 13 in, 1 out]
        n193 = call-poly <vilib>:"DAQmx Create Virtual Channel.vi"("lines"=tag "Dev2/port0/line3") -> ("task out"=w430:refnum<k21>)  [unwired: 13 in, 1 out]
        n194 = call-poly <vilib>:"DAQmx Create Virtual Channel.vi"("lines"=tag "Dev2/port0/line4") -> ("task out"=w429:refnum<k21>)  [unwired: 13 in, 1 out]
        n195 = call-poly <vilib>:"DAQmx Create Virtual Channel.vi"("lines"=tag "Dev2/port0/line6") -> ("task out"=w421:refnum<k21>)  [unwired: 13 in, 1 out]
        n196 = call-poly <vilib>:"DAQmx Create Virtual Channel.vi"("lines"=tag "Dev2/port0/line5") -> ("task out"=w428:refnum<k21>)  [unwired: 13 in, 1 out]
        n197 = call-poly <vilib>:"DAQmx Write.vi"("task/channels in"=w432, "data"=FALSE) -> ("task out"=w426:refnum<k21>)  [unwired: 11 in, 2 out]
        n198 = call-poly <vilib>:"DAQmx Write.vi"("task/channels in"=w431, "data"=FALSE) -> ("task out"=w425:refnum<k21>)  [unwired: 11 in, 2 out]
        n199 = call-poly <vilib>:"DAQmx Write.vi"("task/channels in"=w433, "data"=FALSE) -> ("task out"=w427:refnum<k21>)  [unwired: 11 in, 2 out]
        n200 = call-poly <vilib>:"DAQmx Write.vi"("task/channels in"=w430, "data"=FALSE) -> ("task out"=w424:refnum<k21>)  [unwired: 11 in, 2 out]
        n201 = call-poly <vilib>:"DAQmx Write.vi"("task/channels in"=w429, "data"=FALSE) -> ("task out"=w423:refnum<k21>)  [unwired: 11 in, 2 out]
        n202 = call-poly <vilib>:"DAQmx Write.vi"("task/channels in"=w421, "data"=FALSE) -> ("task out"=w418:refnum<k21>)  [unwired: 11 in, 2 out]
        n203 = call-poly <vilib>:"DAQmx Write.vi"("task/channels in"=w428, "data"=TRUE) -> ("task out"=w422:refnum<k21>)  [unwired: 11 in, 2 out]
      }
      frame ".9677" {
        # "No Resistor"
        # "30 ohm"
        # ".1 ohm"
        # "1 ohm"
        # "5 ohm"
        # "10 ohm"
        # "100 ohm"
        n204 = call-poly <vilib>:"DAQmx Create Virtual Channel.vi"("lines"=tag "Dev2/port0/line1") -> ("task out"=w460:refnum<k21>)  [unwired: 13 in, 1 out]
        n205 = call-poly <vilib>:"DAQmx Create Virtual Channel.vi"("lines"=tag "Dev2/port0/line0") -> ("task out"=w461:refnum<k21>)  [unwired: 13 in, 1 out]
        n206 = call-poly <vilib>:"DAQmx Create Virtual Channel.vi"("lines"=tag "Dev2/port0/line2") -> ("task out"=w459:refnum<k21>)  [unwired: 13 in, 1 out]
        n207 = call-poly <vilib>:"DAQmx Create Virtual Channel.vi"("lines"=tag "Dev2/port0/line3") -> ("task out"=w458:refnum<k21>)  [unwired: 13 in, 1 out]
        n208 = call-poly <vilib>:"DAQmx Create Virtual Channel.vi"("lines"=tag "Dev2/port0/line4") -> ("task out"=w457:refnum<k21>)  [unwired: 13 in, 1 out]
        n209 = call-poly <vilib>:"DAQmx Create Virtual Channel.vi"("lines"=tag "Dev2/port0/line6") -> ("task out"=w449:refnum<k21>)  [unwired: 13 in, 1 out]
        n210 = call-poly <vilib>:"DAQmx Create Virtual Channel.vi"("lines"=tag "Dev2/port0/line5") -> ("task out"=w456:refnum<k21>)  [unwired: 13 in, 1 out]
        n211 = call-poly <vilib>:"DAQmx Write.vi"("task/channels in"=w460, "data"=FALSE) -> ("task out"=w454:refnum<k21>)  [unwired: 11 in, 2 out]
        n212 = call-poly <vilib>:"DAQmx Write.vi"("task/channels in"=w459, "data"=FALSE) -> ("task out"=w453:refnum<k21>)  [unwired: 11 in, 2 out]
        n213 = call-poly <vilib>:"DAQmx Write.vi"("task/channels in"=w461, "data"=FALSE) -> ("task out"=w455:refnum<k21>)  [unwired: 11 in, 2 out]
        n214 = call-poly <vilib>:"DAQmx Write.vi"("task/channels in"=w458, "data"=FALSE) -> ("task out"=w452:refnum<k21>)  [unwired: 11 in, 2 out]
        n215 = call-poly <vilib>:"DAQmx Write.vi"("task/channels in"=w457, "data"=FALSE) -> ("task out"=w451:refnum<k21>)  [unwired: 11 in, 2 out]
        n216 = call-poly <vilib>:"DAQmx Write.vi"("task/channels in"=w449, "data"=FALSE) -> ("task out"=w446:refnum<k21>)  [unwired: 11 in, 2 out]
        n217 = call-poly <vilib>:"DAQmx Write.vi"("task/channels in"=w456, "data"=TRUE) -> ("task out"=w450:refnum<k21>)  [unwired: 11 in, 2 out]
      }
      frame ".9901" {
        # "No Resistor"
        # "30 ohm"
        # ".1 ohm"
        # "1 ohm"
        # "5 ohm"
        # "10 ohm"
        # "100 ohm"
        n218 = call-poly <vilib>:"DAQmx Create Virtual Channel.vi"("lines"=tag "Dev2/port0/line1") -> ("task out"=w488:refnum<k21>)  [unwired: 13 in, 1 out]
        n219 = call-poly <vilib>:"DAQmx Create Virtual Channel.vi"("lines"=tag "Dev2/port0/line0") -> ("task out"=w489:refnum<k21>)  [unwired: 13 in, 1 out]
        n220 = call-poly <vilib>:"DAQmx Create Virtual Channel.vi"("lines"=tag "Dev2/port0/line2") -> ("task out"=w487:refnum<k21>)  [unwired: 13 in, 1 out]
        n221 = call-poly <vilib>:"DAQmx Create Virtual Channel.vi"("lines"=tag "Dev2/port0/line3") -> ("task out"=w486:refnum<k21>)  [unwired: 13 in, 1 out]
        n222 = call-poly <vilib>:"DAQmx Create Virtual Channel.vi"("lines"=tag "Dev2/port0/line4") -> ("task out"=w485:refnum<k21>)  [unwired: 13 in, 1 out]
        n223 = call-poly <vilib>:"DAQmx Create Virtual Channel.vi"("lines"=tag "Dev2/port0/line6") -> ("task out"=w477:refnum<k21>)  [unwired: 13 in, 1 out]
        n224 = call-poly <vilib>:"DAQmx Create Virtual Channel.vi"("lines"=tag "Dev2/port0/line5") -> ("task out"=w484:refnum<k21>)  [unwired: 13 in, 1 out]
        n225 = call-poly <vilib>:"DAQmx Write.vi"("task/channels in"=w488, "data"=FALSE) -> ("task out"=w482:refnum<k21>)  [unwired: 11 in, 2 out]
        n226 = call-poly <vilib>:"DAQmx Write.vi"("task/channels in"=w487, "data"=FALSE) -> ("task out"=w481:refnum<k21>)  [unwired: 11 in, 2 out]
        n227 = call-poly <vilib>:"DAQmx Write.vi"("task/channels in"=w489, "data"=FALSE) -> ("task out"=w483:refnum<k21>)  [unwired: 11 in, 2 out]
        n228 = call-poly <vilib>:"DAQmx Write.vi"("task/channels in"=w486, "data"=FALSE) -> ("task out"=w480:refnum<k21>)  [unwired: 11 in, 2 out]
        n229 = call-poly <vilib>:"DAQmx Write.vi"("task/channels in"=w485, "data"=FALSE) -> ("task out"=w479:refnum<k21>)  [unwired: 11 in, 2 out]
        n230 = call-poly <vilib>:"DAQmx Write.vi"("task/channels in"=w477, "data"=FALSE) -> ("task out"=w474:refnum<k21>)  [unwired: 11 in, 2 out]
        n231 = call-poly <vilib>:"DAQmx Write.vi"("task/channels in"=w484, "data"=TRUE) -> ("task out"=w478:refnum<k21>)  [unwired: 11 in, 2 out]
      }
      frame "1" {
        # "No Resistor"
        # "30 ohm"
        # ".1 ohm"
        # "1 ohm"
        # "5 ohm"
        # "10 ohm"
        # "100 ohm"
        n232 = call-poly <vilib>:"DAQmx Create Virtual Channel.vi"("lines"=tag "Dev2/port0/line1") -> ("task out"=w516:refnum<k21>)  [unwired: 13 in, 1 out]
        n233 = call-poly <vilib>:"DAQmx Create Virtual Channel.vi"("lines"=tag "Dev2/port0/line0") -> ("task out"=w517:refnum<k21>)  [unwired: 13 in, 1 out]
        n234 = call-poly <vilib>:"DAQmx Create Virtual Channel.vi"("lines"=tag "Dev2/port0/line2") -> ("task out"=w515:refnum<k21>)  [unwired: 13 in, 1 out]
        n235 = call-poly <vilib>:"DAQmx Create Virtual Channel.vi"("lines"=tag "Dev2/port0/line3") -> ("task out"=w514:refnum<k21>)  [unwired: 13 in, 1 out]
        n236 = call-poly <vilib>:"DAQmx Create Virtual Channel.vi"("lines"=tag "Dev2/port0/line4") -> ("task out"=w513:refnum<k21>)  [unwired: 13 in, 1 out]
        n237 = call-poly <vilib>:"DAQmx Create Virtual Channel.vi"("lines"=tag "Dev2/port0/line6") -> ("task out"=w505:refnum<k21>)  [unwired: 13 in, 1 out]
        n238 = call-poly <vilib>:"DAQmx Create Virtual Channel.vi"("lines"=tag "Dev2/port0/line5") -> ("task out"=w512:refnum<k21>)  [unwired: 13 in, 1 out]
        n239 = call-poly <vilib>:"DAQmx Write.vi"("task/channels in"=w516, "data"=FALSE) -> ("task out"=w510:refnum<k21>)  [unwired: 11 in, 2 out]
        n240 = call-poly <vilib>:"DAQmx Write.vi"("task/channels in"=w515, "data"=FALSE) -> ("task out"=w509:refnum<k21>)  [unwired: 11 in, 2 out]
        n241 = call-poly <vilib>:"DAQmx Write.vi"("task/channels in"=w517, "data"=FALSE) -> ("task out"=w511:refnum<k21>)  [unwired: 11 in, 2 out]
        n242 = call-poly <vilib>:"DAQmx Write.vi"("task/channels in"=w514, "data"=FALSE) -> ("task out"=w508:refnum<k21>)  [unwired: 11 in, 2 out]
        n243 = call-poly <vilib>:"DAQmx Write.vi"("task/channels in"=w513, "data"=FALSE) -> ("task out"=w507:refnum<k21>)  [unwired: 11 in, 2 out]
        n244 = call-poly <vilib>:"DAQmx Write.vi"("task/channels in"=w505, "data"=FALSE) -> ("task out"=w502:refnum<k21>)  [unwired: 11 in, 2 out]
        n245 = call-poly <vilib>:"DAQmx Write.vi"("task/channels in"=w512, "data"=TRUE) -> ("task out"=w506:refnum<k21>)  [unwired: 11 in, 2 out]
      }
      frame "2.9126" {
        # "No Resistor"
        # "30 ohm"
        # ".1 ohm"
        # "1 ohm"
        # "5 ohm"
        # "10 ohm"
        # "100 ohm"
        n246 = call-poly <vilib>:"DAQmx Create Virtual Channel.vi"("lines"=tag "Dev2/port0/line1") -> ("task out"=w544:refnum<k21>)  [unwired: 13 in, 1 out]
        n247 = call-poly <vilib>:"DAQmx Create Virtual Channel.vi"("lines"=tag "Dev2/port0/line0") -> ("task out"=w545:refnum<k21>)  [unwired: 13 in, 1 out]
        n248 = call-poly <vilib>:"DAQmx Create Virtual Channel.vi"("lines"=tag "Dev2/port0/line2") -> ("task out"=w543:refnum<k21>)  [unwired: 13 in, 1 out]
        n249 = call-poly <vilib>:"DAQmx Create Virtual Channel.vi"("lines"=tag "Dev2/port0/line3") -> ("task out"=w542:refnum<k21>)  [unwired: 13 in, 1 out]
        n250 = call-poly <vilib>:"DAQmx Create Virtual Channel.vi"("lines"=tag "Dev2/port0/line4") -> ("task out"=w541:refnum<k21>)  [unwired: 13 in, 1 out]
        n251 = call-poly <vilib>:"DAQmx Create Virtual Channel.vi"("lines"=tag "Dev2/port0/line6") -> ("task out"=w533:refnum<k21>)  [unwired: 13 in, 1 out]
        n252 = call-poly <vilib>:"DAQmx Create Virtual Channel.vi"("lines"=tag "Dev2/port0/line5") -> ("task out"=w540:refnum<k21>)  [unwired: 13 in, 1 out]
        n253 = call-poly <vilib>:"DAQmx Write.vi"("task/channels in"=w544, "data"=FALSE) -> ("task out"=w538:refnum<k21>)  [unwired: 11 in, 2 out]
        n254 = call-poly <vilib>:"DAQmx Write.vi"("task/channels in"=w543, "data"=FALSE) -> ("task out"=w537:refnum<k21>)  [unwired: 11 in, 2 out]
        n255 = call-poly <vilib>:"DAQmx Write.vi"("task/channels in"=w545, "data"=FALSE) -> ("task out"=w539:refnum<k21>)  [unwired: 11 in, 2 out]
        n256 = call-poly <vilib>:"DAQmx Write.vi"("task/channels in"=w542, "data"=FALSE) -> ("task out"=w536:refnum<k21>)  [unwired: 11 in, 2 out]
        n257 = call-poly <vilib>:"DAQmx Write.vi"("task/channels in"=w541, "data"=FALSE) -> ("task out"=w535:refnum<k21>)  [unwired: 11 in, 2 out]
        n258 = call-poly <vilib>:"DAQmx Write.vi"("task/channels in"=w533, "data"=FALSE) -> ("task out"=w530:refnum<k21>)  [unwired: 11 in, 2 out]
        n259 = call-poly <vilib>:"DAQmx Write.vi"("task/channels in"=w540, "data"=TRUE) -> ("task out"=w534:refnum<k21>)  [unwired: 11 in, 2 out]
      }
      frame "3" {
        # "No Resistor"
        # "30 ohm"
        # ".1 ohm"
        # "1 ohm"
        # "5 ohm"
        # "10 ohm"
        # "100 ohm"
        n260 = call-poly <vilib>:"DAQmx Create Virtual Channel.vi"("lines"=tag "Dev2/port0/line1") -> ("task out"=w572:refnum<k21>)  [unwired: 13 in, 1 out]
        n261 = call-poly <vilib>:"DAQmx Create Virtual Channel.vi"("lines"=tag "Dev2/port0/line0") -> ("task out"=w573:refnum<k21>)  [unwired: 13 in, 1 out]
        n262 = call-poly <vilib>:"DAQmx Create Virtual Channel.vi"("lines"=tag "Dev2/port0/line2") -> ("task out"=w571:refnum<k21>)  [unwired: 13 in, 1 out]
        n263 = call-poly <vilib>:"DAQmx Create Virtual Channel.vi"("lines"=tag "Dev2/port0/line3") -> ("task out"=w570:refnum<k21>)  [unwired: 13 in, 1 out]
        n264 = call-poly <vilib>:"DAQmx Create Virtual Channel.vi"("lines"=tag "Dev2/port0/line4") -> ("task out"=w569:refnum<k21>)  [unwired: 13 in, 1 out]
        n265 = call-poly <vilib>:"DAQmx Create Virtual Channel.vi"("lines"=tag "Dev2/port0/line6") -> ("task out"=w561:refnum<k21>)  [unwired: 13 in, 1 out]
        n266 = call-poly <vilib>:"DAQmx Create Virtual Channel.vi"("lines"=tag "Dev2/port0/line5") -> ("task out"=w568:refnum<k21>)  [unwired: 13 in, 1 out]
        n267 = call-poly <vilib>:"DAQmx Write.vi"("task/channels in"=w572, "data"=FALSE) -> ("task out"=w566:refnum<k21>)  [unwired: 11 in, 2 out]
        n268 = call-poly <vilib>:"DAQmx Write.vi"("task/channels in"=w571, "data"=FALSE) -> ("task out"=w565:refnum<k21>)  [unwired: 11 in, 2 out]
        n269 = call-poly <vilib>:"DAQmx Write.vi"("task/channels in"=w573, "data"=FALSE) -> ("task out"=w567:refnum<k21>)  [unwired: 11 in, 2 out]
        n270 = call-poly <vilib>:"DAQmx Write.vi"("task/channels in"=w570, "data"=FALSE) -> ("task out"=w564:refnum<k21>)  [unwired: 11 in, 2 out]
        n271 = call-poly <vilib>:"DAQmx Write.vi"("task/channels in"=w569, "data"=FALSE) -> ("task out"=w563:refnum<k21>)  [unwired: 11 in, 2 out]
        n272 = call-poly <vilib>:"DAQmx Write.vi"("task/channels in"=w561, "data"=FALSE) -> ("task out"=w558:refnum<k21>)  [unwired: 11 in, 2 out]
        n273 = call-poly <vilib>:"DAQmx Write.vi"("task/channels in"=w568, "data"=TRUE) -> ("task out"=w562:refnum<k21>)  [unwired: 11 in, 2 out]
      }
      frame "3.2258" {
        # "No Resistor"
        # "30 ohm"
        # ".1 ohm"
        # "1 ohm"
        # "5 ohm"
        # "10 ohm"
        # "100 ohm"
        n274 = call-poly <vilib>:"DAQmx Create Virtual Channel.vi"("lines"=tag "Dev2/port0/line1") -> ("task out"=w600:refnum<k21>)  [unwired: 13 in, 1 out]
        n275 = call-poly <vilib>:"DAQmx Create Virtual Channel.vi"("lines"=tag "Dev2/port0/line0") -> ("task out"=w601:refnum<k21>)  [unwired: 13 in, 1 out]
        n276 = call-poly <vilib>:"DAQmx Create Virtual Channel.vi"("lines"=tag "Dev2/port0/line2") -> ("task out"=w599:refnum<k21>)  [unwired: 13 in, 1 out]
        n277 = call-poly <vilib>:"DAQmx Create Virtual Channel.vi"("lines"=tag "Dev2/port0/line3") -> ("task out"=w598:refnum<k21>)  [unwired: 13 in, 1 out]
        n278 = call-poly <vilib>:"DAQmx Create Virtual Channel.vi"("lines"=tag "Dev2/port0/line4") -> ("task out"=w597:refnum<k21>)  [unwired: 13 in, 1 out]
        n279 = call-poly <vilib>:"DAQmx Create Virtual Channel.vi"("lines"=tag "Dev2/port0/line6") -> ("task out"=w589:refnum<k21>)  [unwired: 13 in, 1 out]
        n280 = call-poly <vilib>:"DAQmx Create Virtual Channel.vi"("lines"=tag "Dev2/port0/line5") -> ("task out"=w596:refnum<k21>)  [unwired: 13 in, 1 out]
        n281 = call-poly <vilib>:"DAQmx Write.vi"("task/channels in"=w600, "data"=FALSE) -> ("task out"=w594:refnum<k21>)  [unwired: 11 in, 2 out]
        n282 = call-poly <vilib>:"DAQmx Write.vi"("task/channels in"=w599, "data"=FALSE) -> ("task out"=w593:refnum<k21>)  [unwired: 11 in, 2 out]
        n283 = call-poly <vilib>:"DAQmx Write.vi"("task/channels in"=w601, "data"=FALSE) -> ("task out"=w595:refnum<k21>)  [unwired: 11 in, 2 out]
        n284 = call-poly <vilib>:"DAQmx Write.vi"("task/channels in"=w598, "data"=FALSE) -> ("task out"=w592:refnum<k21>)  [unwired: 11 in, 2 out]
        n285 = call-poly <vilib>:"DAQmx Write.vi"("task/channels in"=w597, "data"=FALSE) -> ("task out"=w591:refnum<k21>)  [unwired: 11 in, 2 out]
        n286 = call-poly <vilib>:"DAQmx Write.vi"("task/channels in"=w589, "data"=FALSE) -> ("task out"=w586:refnum<k21>)  [unwired: 11 in, 2 out]
        n287 = call-poly <vilib>:"DAQmx Write.vi"("task/channels in"=w596, "data"=TRUE) -> ("task out"=w590:refnum<k21>)  [unwired: 11 in, 2 out]
      }
      frame "3.333" {
        # "No Resistor"
        # "30 ohm"
        # ".1 ohm"
        # "1 ohm"
        # "5 ohm"
        # "10 ohm"
        # "100 ohm"
        n288 = call-poly <vilib>:"DAQmx Create Virtual Channel.vi"("lines"=tag "Dev2/port0/line1") -> ("task out"=w628:refnum<k21>)  [unwired: 13 in, 1 out]
        n289 = call-poly <vilib>:"DAQmx Create Virtual Channel.vi"("lines"=tag "Dev2/port0/line0") -> ("task out"=w629:refnum<k21>)  [unwired: 13 in, 1 out]
        n290 = call-poly <vilib>:"DAQmx Create Virtual Channel.vi"("lines"=tag "Dev2/port0/line2") -> ("task out"=w627:refnum<k21>)  [unwired: 13 in, 1 out]
        n291 = call-poly <vilib>:"DAQmx Create Virtual Channel.vi"("lines"=tag "Dev2/port0/line3") -> ("task out"=w626:refnum<k21>)  [unwired: 13 in, 1 out]
        n292 = call-poly <vilib>:"DAQmx Create Virtual Channel.vi"("lines"=tag "Dev2/port0/line4") -> ("task out"=w625:refnum<k21>)  [unwired: 13 in, 1 out]
        n293 = call-poly <vilib>:"DAQmx Create Virtual Channel.vi"("lines"=tag "Dev2/port0/line6") -> ("task out"=w617:refnum<k21>)  [unwired: 13 in, 1 out]
        n294 = call-poly <vilib>:"DAQmx Create Virtual Channel.vi"("lines"=tag "Dev2/port0/line5") -> ("task out"=w624:refnum<k21>)  [unwired: 13 in, 1 out]
        n295 = call-poly <vilib>:"DAQmx Write.vi"("task/channels in"=w628, "data"=FALSE) -> ("task out"=w622:refnum<k21>)  [unwired: 11 in, 2 out]
        n296 = call-poly <vilib>:"DAQmx Write.vi"("task/channels in"=w627, "data"=FALSE) -> ("task out"=w621:refnum<k21>)  [unwired: 11 in, 2 out]
        n297 = call-poly <vilib>:"DAQmx Write.vi"("task/channels in"=w629, "data"=FALSE) -> ("task out"=w623:refnum<k21>)  [unwired: 11 in, 2 out]
        n298 = call-poly <vilib>:"DAQmx Write.vi"("task/channels in"=w626, "data"=FALSE) -> ("task out"=w620:refnum<k21>)  [unwired: 11 in, 2 out]
        n299 = call-poly <vilib>:"DAQmx Write.vi"("task/channels in"=w625, "data"=FALSE) -> ("task out"=w619:refnum<k21>)  [unwired: 11 in, 2 out]
        n300 = call-poly <vilib>:"DAQmx Write.vi"("task/channels in"=w617, "data"=FALSE) -> ("task out"=w614:refnum<k21>)  [unwired: 11 in, 2 out]
        n301 = call-poly <vilib>:"DAQmx Write.vi"("task/channels in"=w624, "data"=TRUE) -> ("task out"=w618:refnum<k21>)  [unwired: 11 in, 2 out]
      }
      frame "4.1096" {
        # "No Resistor"
        # "30 ohm"
        # ".1 ohm"
        # "1 ohm"
        # "5 ohm"
        # "10 ohm"
        # "100 ohm"
        n302 = call-poly <vilib>:"DAQmx Create Virtual Channel.vi"("lines"=tag "Dev2/port0/line1") -> ("task out"=w656:refnum<k21>)  [unwired: 13 in, 1 out]
        n303 = call-poly <vilib>:"DAQmx Create Virtual Channel.vi"("lines"=tag "Dev2/port0/line0") -> ("task out"=w657:refnum<k21>)  [unwired: 13 in, 1 out]
        n304 = call-poly <vilib>:"DAQmx Create Virtual Channel.vi"("lines"=tag "Dev2/port0/line2") -> ("task out"=w655:refnum<k21>)  [unwired: 13 in, 1 out]
        n305 = call-poly <vilib>:"DAQmx Create Virtual Channel.vi"("lines"=tag "Dev2/port0/line3") -> ("task out"=w654:refnum<k21>)  [unwired: 13 in, 1 out]
        n306 = call-poly <vilib>:"DAQmx Create Virtual Channel.vi"("lines"=tag "Dev2/port0/line4") -> ("task out"=w653:refnum<k21>)  [unwired: 13 in, 1 out]
        n307 = call-poly <vilib>:"DAQmx Create Virtual Channel.vi"("lines"=tag "Dev2/port0/line6") -> ("task out"=w645:refnum<k21>)  [unwired: 13 in, 1 out]
        n308 = call-poly <vilib>:"DAQmx Create Virtual Channel.vi"("lines"=tag "Dev2/port0/line5") -> ("task out"=w652:refnum<k21>)  [unwired: 13 in, 1 out]
        n309 = call-poly <vilib>:"DAQmx Write.vi"("task/channels in"=w656, "data"=FALSE) -> ("task out"=w650:refnum<k21>)  [unwired: 11 in, 2 out]
        n310 = call-poly <vilib>:"DAQmx Write.vi"("task/channels in"=w655, "data"=FALSE) -> ("task out"=w649:refnum<k21>)  [unwired: 11 in, 2 out]
        n311 = call-poly <vilib>:"DAQmx Write.vi"("task/channels in"=w657, "data"=FALSE) -> ("task out"=w651:refnum<k21>)  [unwired: 11 in, 2 out]
        n312 = call-poly <vilib>:"DAQmx Write.vi"("task/channels in"=w654, "data"=FALSE) -> ("task out"=w648:refnum<k21>)  [unwired: 11 in, 2 out]
        n313 = call-poly <vilib>:"DAQmx Write.vi"("task/channels in"=w653, "data"=FALSE) -> ("task out"=w647:refnum<k21>)  [unwired: 11 in, 2 out]
        n314 = call-poly <vilib>:"DAQmx Write.vi"("task/channels in"=w645, "data"=FALSE) -> ("task out"=w642:refnum<k21>)  [unwired: 11 in, 2 out]
        n315 = call-poly <vilib>:"DAQmx Write.vi"("task/channels in"=w652, "data"=TRUE) -> ("task out"=w646:refnum<k21>)  [unwired: 11 in, 2 out]
      }
      frame "4.2857" {
        # "No Resistor"
        # "30 ohm"
        # ".1 ohm"
        # "1 ohm"
        # "5 ohm"
        # "10 ohm"
        # "100 ohm"
        n316 = call-poly <vilib>:"DAQmx Create Virtual Channel.vi"("lines"=tag "Dev2/port0/line1") -> ("task out"=w684:refnum<k21>)  [unwired: 13 in, 1 out]
        n317 = call-poly <vilib>:"DAQmx Create Virtual Channel.vi"("lines"=tag "Dev2/port0/line0") -> ("task out"=w685:refnum<k21>)  [unwired: 13 in, 1 out]
        n318 = call-poly <vilib>:"DAQmx Create Virtual Channel.vi"("lines"=tag "Dev2/port0/line2") -> ("task out"=w683:refnum<k21>)  [unwired: 13 in, 1 out]
        n319 = call-poly <vilib>:"DAQmx Create Virtual Channel.vi"("lines"=tag "Dev2/port0/line3") -> ("task out"=w682:refnum<k21>)  [unwired: 13 in, 1 out]
        n320 = call-poly <vilib>:"DAQmx Create Virtual Channel.vi"("lines"=tag "Dev2/port0/line4") -> ("task out"=w681:refnum<k21>)  [unwired: 13 in, 1 out]
        n321 = call-poly <vilib>:"DAQmx Create Virtual Channel.vi"("lines"=tag "Dev2/port0/line6") -> ("task out"=w673:refnum<k21>)  [unwired: 13 in, 1 out]
        n322 = call-poly <vilib>:"DAQmx Create Virtual Channel.vi"("lines"=tag "Dev2/port0/line5") -> ("task out"=w680:refnum<k21>)  [unwired: 13 in, 1 out]
        n323 = call-poly <vilib>:"DAQmx Write.vi"("task/channels in"=w684, "data"=FALSE) -> ("task out"=w678:refnum<k21>)  [unwired: 11 in, 2 out]
        n324 = call-poly <vilib>:"DAQmx Write.vi"("task/channels in"=w683, "data"=FALSE) -> ("task out"=w677:refnum<k21>)  [unwired: 11 in, 2 out]
        n325 = call-poly <vilib>:"DAQmx Write.vi"("task/channels in"=w685, "data"=FALSE) -> ("task out"=w679:refnum<k21>)  [unwired: 11 in, 2 out]
        n326 = call-poly <vilib>:"DAQmx Write.vi"("task/channels in"=w682, "data"=FALSE) -> ("task out"=w676:refnum<k21>)  [unwired: 11 in, 2 out]
        n327 = call-poly <vilib>:"DAQmx Write.vi"("task/channels in"=w681, "data"=FALSE) -> ("task out"=w675:refnum<k21>)  [unwired: 11 in, 2 out]
        n328 = call-poly <vilib>:"DAQmx Write.vi"("task/channels in"=w673, "data"=FALSE) -> ("task out"=w670:refnum<k21>)  [unwired: 11 in, 2 out]
        n329 = call-poly <vilib>:"DAQmx Write.vi"("task/channels in"=w680, "data"=TRUE) -> ("task out"=w674:refnum<k21>)  [unwired: 11 in, 2 out]
      }
      frame "4.7619" {
        # "No Resistor"
        # "30 ohm"
        # ".1 ohm"
        # "1 ohm"
        # "5 ohm"
        # "10 ohm"
        # "100 ohm"
        n330 = call-poly <vilib>:"DAQmx Create Virtual Channel.vi"("lines"=tag "Dev2/port0/line1") -> ("task out"=w712:refnum<k21>)  [unwired: 13 in, 1 out]
        n331 = call-poly <vilib>:"DAQmx Create Virtual Channel.vi"("lines"=tag "Dev2/port0/line0") -> ("task out"=w713:refnum<k21>)  [unwired: 13 in, 1 out]
        n332 = call-poly <vilib>:"DAQmx Create Virtual Channel.vi"("lines"=tag "Dev2/port0/line2") -> ("task out"=w711:refnum<k21>)  [unwired: 13 in, 1 out]
        n333 = call-poly <vilib>:"DAQmx Create Virtual Channel.vi"("lines"=tag "Dev2/port0/line3") -> ("task out"=w710:refnum<k21>)  [unwired: 13 in, 1 out]
        n334 = call-poly <vilib>:"DAQmx Create Virtual Channel.vi"("lines"=tag "Dev2/port0/line4") -> ("task out"=w709:refnum<k21>)  [unwired: 13 in, 1 out]
        n335 = call-poly <vilib>:"DAQmx Create Virtual Channel.vi"("lines"=tag "Dev2/port0/line6") -> ("task out"=w701:refnum<k21>)  [unwired: 13 in, 1 out]
        n336 = call-poly <vilib>:"DAQmx Create Virtual Channel.vi"("lines"=tag "Dev2/port0/line5") -> ("task out"=w708:refnum<k21>)  [unwired: 13 in, 1 out]
        n337 = call-poly <vilib>:"DAQmx Write.vi"("task/channels in"=w712, "data"=FALSE) -> ("task out"=w706:refnum<k21>)  [unwired: 11 in, 2 out]
        n338 = call-poly <vilib>:"DAQmx Write.vi"("task/channels in"=w711, "data"=FALSE) -> ("task out"=w705:refnum<k21>)  [unwired: 11 in, 2 out]
        n339 = call-poly <vilib>:"DAQmx Write.vi"("task/channels in"=w713, "data"=FALSE) -> ("task out"=w707:refnum<k21>)  [unwired: 11 in, 2 out]
        n340 = call-poly <vilib>:"DAQmx Write.vi"("task/channels in"=w710, "data"=FALSE) -> ("task out"=w704:refnum<k21>)  [unwired: 11 in, 2 out]
        n341 = call-poly <vilib>:"DAQmx Write.vi"("task/channels in"=w709, "data"=FALSE) -> ("task out"=w703:refnum<k21>)  [unwired: 11 in, 2 out]
        n342 = call-poly <vilib>:"DAQmx Write.vi"("task/channels in"=w701, "data"=FALSE) -> ("task out"=w698:refnum<k21>)  [unwired: 11 in, 2 out]
        n343 = call-poly <vilib>:"DAQmx Write.vi"("task/channels in"=w708, "data"=TRUE) -> ("task out"=w702:refnum<k21>)  [unwired: 11 in, 2 out]
      }
      frame "5" {
        # "No Resistor"
        # "30 ohm"
        # ".1 ohm"
        # "1 ohm"
        # "5 ohm"
        # "10 ohm"
        # "100 ohm"
        n344 = call-poly <vilib>:"DAQmx Create Virtual Channel.vi"("lines"=tag "Dev2/port0/line1") -> ("task out"=w740:refnum<k21>)  [unwired: 13 in, 1 out]
        n345 = call-poly <vilib>:"DAQmx Create Virtual Channel.vi"("lines"=tag "Dev2/port0/line0") -> ("task out"=w741:refnum<k21>)  [unwired: 13 in, 1 out]
        n346 = call-poly <vilib>:"DAQmx Create Virtual Channel.vi"("lines"=tag "Dev2/port0/line2") -> ("task out"=w739:refnum<k21>)  [unwired: 13 in, 1 out]
        n347 = call-poly <vilib>:"DAQmx Create Virtual Channel.vi"("lines"=tag "Dev2/port0/line3") -> ("task out"=w738:refnum<k21>)  [unwired: 13 in, 1 out]
        n348 = call-poly <vilib>:"DAQmx Create Virtual Channel.vi"("lines"=tag "Dev2/port0/line4") -> ("task out"=w737:refnum<k21>)  [unwired: 13 in, 1 out]
        n349 = call-poly <vilib>:"DAQmx Create Virtual Channel.vi"("lines"=tag "Dev2/port0/line6") -> ("task out"=w729:refnum<k21>)  [unwired: 13 in, 1 out]
        n350 = call-poly <vilib>:"DAQmx Create Virtual Channel.vi"("lines"=tag "Dev2/port0/line5") -> ("task out"=w736:refnum<k21>)  [unwired: 13 in, 1 out]
        n351 = call-poly <vilib>:"DAQmx Write.vi"("task/channels in"=w740, "data"=FALSE) -> ("task out"=w734:refnum<k21>)  [unwired: 11 in, 2 out]
        n352 = call-poly <vilib>:"DAQmx Write.vi"("task/channels in"=w739, "data"=FALSE) -> ("task out"=w733:refnum<k21>)  [unwired: 11 in, 2 out]
        n353 = call-poly <vilib>:"DAQmx Write.vi"("task/channels in"=w741, "data"=FALSE) -> ("task out"=w735:refnum<k21>)  [unwired: 11 in, 2 out]
        n354 = call-poly <vilib>:"DAQmx Write.vi"("task/channels in"=w738, "data"=FALSE) -> ("task out"=w732:refnum<k21>)  [unwired: 11 in, 2 out]
        n355 = call-poly <vilib>:"DAQmx Write.vi"("task/channels in"=w737, "data"=FALSE) -> ("task out"=w731:refnum<k21>)  [unwired: 11 in, 2 out]
        n356 = call-poly <vilib>:"DAQmx Write.vi"("task/channels in"=w729, "data"=FALSE) -> ("task out"=w726:refnum<k21>)  [unwired: 11 in, 2 out]
        n357 = call-poly <vilib>:"DAQmx Write.vi"("task/channels in"=w736, "data"=TRUE) -> ("task out"=w730:refnum<k21>)  [unwired: 11 in, 2 out]
      }
      frame "6.9767" {
        # "No Resistor"
        # "30 ohm"
        # ".1 ohm"
        # "1 ohm"
        # "5 ohm"
        # "10 ohm"
        # "100 ohm"
        n358 = call-poly <vilib>:"DAQmx Create Virtual Channel.vi"("lines"=tag "Dev2/port0/line1") -> ("task out"=w768:refnum<k21>)  [unwired: 13 in, 1 out]
        n359 = call-poly <vilib>:"DAQmx Create Virtual Channel.vi"("lines"=tag "Dev2/port0/line0") -> ("task out"=w769:refnum<k21>)  [unwired: 13 in, 1 out]
        n360 = call-poly <vilib>:"DAQmx Create Virtual Channel.vi"("lines"=tag "Dev2/port0/line2") -> ("task out"=w767:refnum<k21>)  [unwired: 13 in, 1 out]
        n361 = call-poly <vilib>:"DAQmx Create Virtual Channel.vi"("lines"=tag "Dev2/port0/line3") -> ("task out"=w766:refnum<k21>)  [unwired: 13 in, 1 out]
        n362 = call-poly <vilib>:"DAQmx Create Virtual Channel.vi"("lines"=tag "Dev2/port0/line4") -> ("task out"=w765:refnum<k21>)  [unwired: 13 in, 1 out]
        n363 = call-poly <vilib>:"DAQmx Create Virtual Channel.vi"("lines"=tag "Dev2/port0/line6") -> ("task out"=w757:refnum<k21>)  [unwired: 13 in, 1 out]
        n364 = call-poly <vilib>:"DAQmx Create Virtual Channel.vi"("lines"=tag "Dev2/port0/line5") -> ("task out"=w764:refnum<k21>)  [unwired: 13 in, 1 out]
        n365 = call-poly <vilib>:"DAQmx Write.vi"("task/channels in"=w768, "data"=FALSE) -> ("task out"=w762:refnum<k21>)  [unwired: 11 in, 2 out]
        n366 = call-poly <vilib>:"DAQmx Write.vi"("task/channels in"=w767, "data"=FALSE) -> ("task out"=w761:refnum<k21>)  [unwired: 11 in, 2 out]
        n367 = call-poly <vilib>:"DAQmx Write.vi"("task/channels in"=w769, "data"=FALSE) -> ("task out"=w763:refnum<k21>)  [unwired: 11 in, 2 out]
        n368 = call-poly <vilib>:"DAQmx Write.vi"("task/channels in"=w766, "data"=FALSE) -> ("task out"=w760:refnum<k21>)  [unwired: 11 in, 2 out]
        n369 = call-poly <vilib>:"DAQmx Write.vi"("task/channels in"=w765, "data"=FALSE) -> ("task out"=w759:refnum<k21>)  [unwired: 11 in, 2 out]
        n370 = call-poly <vilib>:"DAQmx Write.vi"("task/channels in"=w757, "data"=FALSE) -> ("task out"=w754:refnum<k21>)  [unwired: 11 in, 2 out]
        n371 = call-poly <vilib>:"DAQmx Write.vi"("task/channels in"=w764, "data"=TRUE) -> ("task out"=w758:refnum<k21>)  [unwired: 11 in, 2 out]
      }
      frame "7.5" {
        # "No Resistor"
        # "30 ohm"
        # ".1 ohm"
        # "1 ohm"
        # "5 ohm"
        # "10 ohm"
        # "100 ohm"
        n372 = call-poly <vilib>:"DAQmx Create Virtual Channel.vi"("lines"=tag "Dev2/port0/line1") -> ("task out"=w796:refnum<k21>)  [unwired: 13 in, 1 out]
        n373 = call-poly <vilib>:"DAQmx Create Virtual Channel.vi"("lines"=tag "Dev2/port0/line0") -> ("task out"=w797:refnum<k21>)  [unwired: 13 in, 1 out]
        n374 = call-poly <vilib>:"DAQmx Create Virtual Channel.vi"("lines"=tag "Dev2/port0/line2") -> ("task out"=w795:refnum<k21>)  [unwired: 13 in, 1 out]
        n375 = call-poly <vilib>:"DAQmx Create Virtual Channel.vi"("lines"=tag "Dev2/port0/line3") -> ("task out"=w794:refnum<k21>)  [unwired: 13 in, 1 out]
        n376 = call-poly <vilib>:"DAQmx Create Virtual Channel.vi"("lines"=tag "Dev2/port0/line4") -> ("task out"=w793:refnum<k21>)  [unwired: 13 in, 1 out]
        n377 = call-poly <vilib>:"DAQmx Create Virtual Channel.vi"("lines"=tag "Dev2/port0/line6") -> ("task out"=w785:refnum<k21>)  [unwired: 13 in, 1 out]
        n378 = call-poly <vilib>:"DAQmx Create Virtual Channel.vi"("lines"=tag "Dev2/port0/line5") -> ("task out"=w792:refnum<k21>)  [unwired: 13 in, 1 out]
        n379 = call-poly <vilib>:"DAQmx Write.vi"("task/channels in"=w796, "data"=FALSE) -> ("task out"=w790:refnum<k21>)  [unwired: 11 in, 2 out]
        n380 = call-poly <vilib>:"DAQmx Write.vi"("task/channels in"=w795, "data"=FALSE) -> ("task out"=w789:refnum<k21>)  [unwired: 11 in, 2 out]
        n381 = call-poly <vilib>:"DAQmx Write.vi"("task/channels in"=w797, "data"=FALSE) -> ("task out"=w791:refnum<k21>)  [unwired: 11 in, 2 out]
        n382 = call-poly <vilib>:"DAQmx Write.vi"("task/channels in"=w794, "data"=FALSE) -> ("task out"=w788:refnum<k21>)  [unwired: 11 in, 2 out]
        n383 = call-poly <vilib>:"DAQmx Write.vi"("task/channels in"=w793, "data"=FALSE) -> ("task out"=w787:refnum<k21>)  [unwired: 11 in, 2 out]
        n384 = call-poly <vilib>:"DAQmx Write.vi"("task/channels in"=w785, "data"=FALSE) -> ("task out"=w782:refnum<k21>)  [unwired: 11 in, 2 out]
        n385 = call-poly <vilib>:"DAQmx Write.vi"("task/channels in"=w792, "data"=TRUE) -> ("task out"=w786:refnum<k21>)  [unwired: 11 in, 2 out]
      }
      frame "9.0909" {
        # "No Resistor"
        # "30 ohm"
        # ".1 ohm"
        # "1 ohm"
        # "5 ohm"
        # "10 ohm"
        # "100 ohm"
        n386 = call-poly <vilib>:"DAQmx Create Virtual Channel.vi"("lines"=tag "Dev2/port0/line1") -> ("task out"=w824:refnum<k21>)  [unwired: 13 in, 1 out]
        n387 = call-poly <vilib>:"DAQmx Create Virtual Channel.vi"("lines"=tag "Dev2/port0/line0") -> ("task out"=w825:refnum<k21>)  [unwired: 13 in, 1 out]
        n388 = call-poly <vilib>:"DAQmx Create Virtual Channel.vi"("lines"=tag "Dev2/port0/line2") -> ("task out"=w823:refnum<k21>)  [unwired: 13 in, 1 out]
        n389 = call-poly <vilib>:"DAQmx Create Virtual Channel.vi"("lines"=tag "Dev2/port0/line3") -> ("task out"=w822:refnum<k21>)  [unwired: 13 in, 1 out]
        n390 = call-poly <vilib>:"DAQmx Create Virtual Channel.vi"("lines"=tag "Dev2/port0/line4") -> ("task out"=w821:refnum<k21>)  [unwired: 13 in, 1 out]
        n391 = call-poly <vilib>:"DAQmx Create Virtual Channel.vi"("lines"=tag "Dev2/port0/line6") -> ("task out"=w813:refnum<k21>)  [unwired: 13 in, 1 out]
        n392 = call-poly <vilib>:"DAQmx Create Virtual Channel.vi"("lines"=tag "Dev2/port0/line5") -> ("task out"=w820:refnum<k21>)  [unwired: 13 in, 1 out]
        n393 = call-poly <vilib>:"DAQmx Write.vi"("task/channels in"=w824, "data"=FALSE) -> ("task out"=w818:refnum<k21>)  [unwired: 11 in, 2 out]
        n394 = call-poly <vilib>:"DAQmx Write.vi"("task/channels in"=w823, "data"=FALSE) -> ("task out"=w817:refnum<k21>)  [unwired: 11 in, 2 out]
        n395 = call-poly <vilib>:"DAQmx Write.vi"("task/channels in"=w825, "data"=FALSE) -> ("task out"=w819:refnum<k21>)  [unwired: 11 in, 2 out]
        n396 = call-poly <vilib>:"DAQmx Write.vi"("task/channels in"=w822, "data"=FALSE) -> ("task out"=w816:refnum<k21>)  [unwired: 11 in, 2 out]
        n397 = call-poly <vilib>:"DAQmx Write.vi"("task/channels in"=w821, "data"=FALSE) -> ("task out"=w815:refnum<k21>)  [unwired: 11 in, 2 out]
        n398 = call-poly <vilib>:"DAQmx Write.vi"("task/channels in"=w813, "data"=FALSE) -> ("task out"=w810:refnum<k21>)  [unwired: 11 in, 2 out]
        n399 = call-poly <vilib>:"DAQmx Write.vi"("task/channels in"=w820, "data"=TRUE) -> ("task out"=w814:refnum<k21>)  [unwired: 11 in, 2 out]
      }
      frame "10" {
        # "No Resistor"
        # "30 ohm"
        # ".1 ohm"
        # "1 ohm"
        # "5 ohm"
        # "10 ohm"
        # "100 ohm"
        n400 = call-poly <vilib>:"DAQmx Create Virtual Channel.vi"("lines"=tag "Dev2/port0/line1") -> ("task out"=w852:refnum<k21>)  [unwired: 13 in, 1 out]
        n401 = call-poly <vilib>:"DAQmx Create Virtual Channel.vi"("lines"=tag "Dev2/port0/line0") -> ("task out"=w853:refnum<k21>)  [unwired: 13 in, 1 out]
        n402 = call-poly <vilib>:"DAQmx Create Virtual Channel.vi"("lines"=tag "Dev2/port0/line2") -> ("task out"=w851:refnum<k21>)  [unwired: 13 in, 1 out]
        n403 = call-poly <vilib>:"DAQmx Create Virtual Channel.vi"("lines"=tag "Dev2/port0/line3") -> ("task out"=w850:refnum<k21>)  [unwired: 13 in, 1 out]
        n404 = call-poly <vilib>:"DAQmx Create Virtual Channel.vi"("lines"=tag "Dev2/port0/line4") -> ("task out"=w849:refnum<k21>)  [unwired: 13 in, 1 out]
        n405 = call-poly <vilib>:"DAQmx Create Virtual Channel.vi"("lines"=tag "Dev2/port0/line6") -> ("task out"=w841:refnum<k21>)  [unwired: 13 in, 1 out]
        n406 = call-poly <vilib>:"DAQmx Create Virtual Channel.vi"("lines"=tag "Dev2/port0/line5") -> ("task out"=w848:refnum<k21>)  [unwired: 13 in, 1 out]
        n407 = call-poly <vilib>:"DAQmx Write.vi"("task/channels in"=w852, "data"=FALSE) -> ("task out"=w846:refnum<k21>)  [unwired: 11 in, 2 out]
        n408 = call-poly <vilib>:"DAQmx Write.vi"("task/channels in"=w851, "data"=FALSE) -> ("task out"=w845:refnum<k21>)  [unwired: 11 in, 2 out]
        n409 = call-poly <vilib>:"DAQmx Write.vi"("task/channels in"=w853, "data"=FALSE) -> ("task out"=w847:refnum<k21>)  [unwired: 11 in, 2 out]
        n410 = call-poly <vilib>:"DAQmx Write.vi"("task/channels in"=w850, "data"=FALSE) -> ("task out"=w844:refnum<k21>)  [unwired: 11 in, 2 out]
        n411 = call-poly <vilib>:"DAQmx Write.vi"("task/channels in"=w849, "data"=FALSE) -> ("task out"=w843:refnum<k21>)  [unwired: 11 in, 2 out]
        n412 = call-poly <vilib>:"DAQmx Write.vi"("task/channels in"=w841, "data"=FALSE) -> ("task out"=w838:refnum<k21>)  [unwired: 11 in, 2 out]
        n413 = call-poly <vilib>:"DAQmx Write.vi"("task/channels in"=w848, "data"=TRUE) -> ("task out"=w842:refnum<k21>)  [unwired: 11 in, 2 out]
      }
      frame "23.0769" {
        # "No Resistor"
        # "30 ohm"
        # ".1 ohm"
        # "1 ohm"
        # "5 ohm"
        # "10 ohm"
        # "100 ohm"
        n414 = call-poly <vilib>:"DAQmx Create Virtual Channel.vi"("lines"=tag "Dev2/port0/line1") -> ("task out"=w880:refnum<k21>)  [unwired: 13 in, 1 out]
        n415 = call-poly <vilib>:"DAQmx Create Virtual Channel.vi"("lines"=tag "Dev2/port0/line0") -> ("task out"=w881:refnum<k21>)  [unwired: 13 in, 1 out]
        n416 = call-poly <vilib>:"DAQmx Create Virtual Channel.vi"("lines"=tag "Dev2/port0/line2") -> ("task out"=w879:refnum<k21>)  [unwired: 13 in, 1 out]
        n417 = call-poly <vilib>:"DAQmx Create Virtual Channel.vi"("lines"=tag "Dev2/port0/line3") -> ("task out"=w878:refnum<k21>)  [unwired: 13 in, 1 out]
        n418 = call-poly <vilib>:"DAQmx Create Virtual Channel.vi"("lines"=tag "Dev2/port0/line4") -> ("task out"=w877:refnum<k21>)  [unwired: 13 in, 1 out]
        n419 = call-poly <vilib>:"DAQmx Create Virtual Channel.vi"("lines"=tag "Dev2/port0/line6") -> ("task out"=w869:refnum<k21>)  [unwired: 13 in, 1 out]
        n420 = call-poly <vilib>:"DAQmx Create Virtual Channel.vi"("lines"=tag "Dev2/port0/line5") -> ("task out"=w876:refnum<k21>)  [unwired: 13 in, 1 out]
        n421 = call-poly <vilib>:"DAQmx Write.vi"("task/channels in"=w880, "data"=FALSE) -> ("task out"=w874:refnum<k21>)  [unwired: 11 in, 2 out]
        n422 = call-poly <vilib>:"DAQmx Write.vi"("task/channels in"=w879, "data"=FALSE) -> ("task out"=w873:refnum<k21>)  [unwired: 11 in, 2 out]
        n423 = call-poly <vilib>:"DAQmx Write.vi"("task/channels in"=w881, "data"=FALSE) -> ("task out"=w875:refnum<k21>)  [unwired: 11 in, 2 out]
        n424 = call-poly <vilib>:"DAQmx Write.vi"("task/channels in"=w878, "data"=FALSE) -> ("task out"=w872:refnum<k21>)  [unwired: 11 in, 2 out]
        n425 = call-poly <vilib>:"DAQmx Write.vi"("task/channels in"=w877, "data"=FALSE) -> ("task out"=w871:refnum<k21>)  [unwired: 11 in, 2 out]
        n426 = call-poly <vilib>:"DAQmx Write.vi"("task/channels in"=w869, "data"=FALSE) -> ("task out"=w866:refnum<k21>)  [unwired: 11 in, 2 out]
        n427 = call-poly <vilib>:"DAQmx Write.vi"("task/channels in"=w876, "data"=TRUE) -> ("task out"=w870:refnum<k21>)  [unwired: 11 in, 2 out]
      }
      frame "30" {
        # "No Resistor"
        # "30 ohm"
        # ".1 ohm"
        # "1 ohm"
        # "5 ohm"
        # "10 ohm"
        # "100 ohm"
        n428 = call-poly <vilib>:"DAQmx Create Virtual Channel.vi"("lines"=tag "Dev2/port0/line1") -> ("task out"=w908:refnum<k21>)  [unwired: 13 in, 1 out]
        n429 = call-poly <vilib>:"DAQmx Create Virtual Channel.vi"("lines"=tag "Dev2/port0/line0") -> ("task out"=w909:refnum<k21>)  [unwired: 13 in, 1 out]
        n430 = call-poly <vilib>:"DAQmx Create Virtual Channel.vi"("lines"=tag "Dev2/port0/line2") -> ("task out"=w907:refnum<k21>)  [unwired: 13 in, 1 out]
        n431 = call-poly <vilib>:"DAQmx Create Virtual Channel.vi"("lines"=tag "Dev2/port0/line3") -> ("task out"=w906:refnum<k21>)  [unwired: 13 in, 1 out]
        n432 = call-poly <vilib>:"DAQmx Create Virtual Channel.vi"("lines"=tag "Dev2/port0/line4") -> ("task out"=w905:refnum<k21>)  [unwired: 13 in, 1 out]
        n433 = call-poly <vilib>:"DAQmx Create Virtual Channel.vi"("lines"=tag "Dev2/port0/line6") -> ("task out"=w897:refnum<k21>)  [unwired: 13 in, 1 out]
        n434 = call-poly <vilib>:"DAQmx Create Virtual Channel.vi"("lines"=tag "Dev2/port0/line5") -> ("task out"=w904:refnum<k21>)  [unwired: 13 in, 1 out]
        n435 = call-poly <vilib>:"DAQmx Write.vi"("task/channels in"=w908, "data"=FALSE) -> ("task out"=w902:refnum<k21>)  [unwired: 11 in, 2 out]
        n436 = call-poly <vilib>:"DAQmx Write.vi"("task/channels in"=w907, "data"=FALSE) -> ("task out"=w901:refnum<k21>)  [unwired: 11 in, 2 out]
        n437 = call-poly <vilib>:"DAQmx Write.vi"("task/channels in"=w909, "data"=FALSE) -> ("task out"=w903:refnum<k21>)  [unwired: 11 in, 2 out]
        n438 = call-poly <vilib>:"DAQmx Write.vi"("task/channels in"=w906, "data"=FALSE) -> ("task out"=w900:refnum<k21>)  [unwired: 11 in, 2 out]
        n439 = call-poly <vilib>:"DAQmx Write.vi"("task/channels in"=w905, "data"=FALSE) -> ("task out"=w899:refnum<k21>)  [unwired: 11 in, 2 out]
        n440 = call-poly <vilib>:"DAQmx Write.vi"("task/channels in"=w897, "data"=FALSE) -> ("task out"=w894:refnum<k21>)  [unwired: 11 in, 2 out]
        n441 = call-poly <vilib>:"DAQmx Write.vi"("task/channels in"=w904, "data"=TRUE) -> ("task out"=w898:refnum<k21>)  [unwired: 11 in, 2 out]
      }
      frame "100" {
        # "No Resistor"
        # "30 ohm"
        # ".1 ohm"
        # "1 ohm"
        # "5 ohm"
        # "10 ohm"
        # "100 ohm"
        n442 = call-poly <vilib>:"DAQmx Create Virtual Channel.vi"("lines"=tag "Dev2/port0/line1") -> ("task out"=w936:refnum<k21>)  [unwired: 13 in, 1 out]
        n443 = call-poly <vilib>:"DAQmx Create Virtual Channel.vi"("lines"=tag "Dev2/port0/line0") -> ("task out"=w937:refnum<k21>)  [unwired: 13 in, 1 out]
        n444 = call-poly <vilib>:"DAQmx Create Virtual Channel.vi"("lines"=tag "Dev2/port0/line2") -> ("task out"=w935:refnum<k21>)  [unwired: 13 in, 1 out]
        n445 = call-poly <vilib>:"DAQmx Create Virtual Channel.vi"("lines"=tag "Dev2/port0/line3") -> ("task out"=w934:refnum<k21>)  [unwired: 13 in, 1 out]
        n446 = call-poly <vilib>:"DAQmx Create Virtual Channel.vi"("lines"=tag "Dev2/port0/line4") -> ("task out"=w933:refnum<k21>)  [unwired: 13 in, 1 out]
        n447 = call-poly <vilib>:"DAQmx Create Virtual Channel.vi"("lines"=tag "Dev2/port0/line6") -> ("task out"=w925:refnum<k21>)  [unwired: 13 in, 1 out]
        n448 = call-poly <vilib>:"DAQmx Create Virtual Channel.vi"("lines"=tag "Dev2/port0/line5") -> ("task out"=w932:refnum<k21>)  [unwired: 13 in, 1 out]
        n449 = call-poly <vilib>:"DAQmx Write.vi"("task/channels in"=w936, "data"=FALSE) -> ("task out"=w930:refnum<k21>)  [unwired: 11 in, 2 out]
        n450 = call-poly <vilib>:"DAQmx Write.vi"("task/channels in"=w935, "data"=FALSE) -> ("task out"=w929:refnum<k21>)  [unwired: 11 in, 2 out]
        n451 = call-poly <vilib>:"DAQmx Write.vi"("task/channels in"=w937, "data"=FALSE) -> ("task out"=w931:refnum<k21>)  [unwired: 11 in, 2 out]
        n452 = call-poly <vilib>:"DAQmx Write.vi"("task/channels in"=w934, "data"=FALSE) -> ("task out"=w928:refnum<k21>)  [unwired: 11 in, 2 out]
        n453 = call-poly <vilib>:"DAQmx Write.vi"("task/channels in"=w933, "data"=FALSE) -> ("task out"=w927:refnum<k21>)  [unwired: 11 in, 2 out]
        n454 = call-poly <vilib>:"DAQmx Write.vi"("task/channels in"=w925, "data"=FALSE) -> ("task out"=w922:refnum<k21>)  [unwired: 11 in, 2 out]
        n455 = call-poly <vilib>:"DAQmx Write.vi"("task/channels in"=w932, "data"=TRUE) -> ("task out"=w926:refnum<k21>)  [unwired: 11 in, 2 out]
      }
      frame "0", Default {
        # "No Resistor"
        # "30 ohm"
        # ".1 ohm"
        # "1 ohm"
        # "5 ohm"
        # "10 ohm"
        # "100 ohm"
        n456 = call-poly <vilib>:"DAQmx Create Virtual Channel.vi"("lines"=tag "Dev2/port0/line1") -> ("task out"=w964:refnum<k21>)  [unwired: 13 in, 1 out]
        n457 = call-poly <vilib>:"DAQmx Create Virtual Channel.vi"("lines"=tag "Dev2/port0/line0") -> ("task out"=w965:refnum<k21>)  [unwired: 13 in, 1 out]
        n458 = call-poly <vilib>:"DAQmx Create Virtual Channel.vi"("lines"=tag "Dev2/port0/line2") -> ("task out"=w963:refnum<k21>)  [unwired: 13 in, 1 out]
        n459 = call-poly <vilib>:"DAQmx Create Virtual Channel.vi"("lines"=tag "Dev2/port0/line3") -> ("task out"=w962:refnum<k21>)  [unwired: 13 in, 1 out]
        n460 = call-poly <vilib>:"DAQmx Create Virtual Channel.vi"("lines"=tag "Dev2/port0/line4") -> ("task out"=w961:refnum<k21>)  [unwired: 13 in, 1 out]
        n461 = call-poly <vilib>:"DAQmx Create Virtual Channel.vi"("lines"=tag "Dev2/port0/line6") -> ("task out"=w953:refnum<k21>)  [unwired: 13 in, 1 out]
        n462 = call-poly <vilib>:"DAQmx Create Virtual Channel.vi"("lines"=tag "Dev2/port0/line5") -> ("task out"=w960:refnum<k21>)  [unwired: 13 in, 1 out]
        n463 = call-poly <vilib>:"DAQmx Write.vi"("task/channels in"=w964, "data"=FALSE) -> ("task out"=w958:refnum<k21>)  [unwired: 11 in, 2 out]
        n464 = call-poly <vilib>:"DAQmx Write.vi"("task/channels in"=w963, "data"=FALSE) -> ("task out"=w957:refnum<k21>)  [unwired: 11 in, 2 out]
        n465 = call-poly <vilib>:"DAQmx Write.vi"("task/channels in"=w965, "data"=FALSE) -> ("task out"=w959:refnum<k21>)  [unwired: 11 in, 2 out]
        n466 = call-poly <vilib>:"DAQmx Write.vi"("task/channels in"=w962, "data"=FALSE) -> ("task out"=w956:refnum<k21>)  [unwired: 11 in, 2 out]
        n467 = call-poly <vilib>:"DAQmx Write.vi"("task/channels in"=w961, "data"=FALSE) -> ("task out"=w955:refnum<k21>)  [unwired: 11 in, 2 out]
        n468 = call-poly <vilib>:"DAQmx Write.vi"("task/channels in"=w953, "data"=FALSE) -> ("task out"=w950:refnum<k21>)  [unwired: 11 in, 2 out]
        n469 = call-poly <vilib>:"DAQmx Write.vi"("task/channels in"=w960, "data"=TRUE) -> ("task out"=w954:refnum<k21>)  [unwired: 11 in, 2 out]
      }
      frame ".0882" {
        # "No Resistor"
        # "30 ohm"
        # ".1 ohm"
        # "1 ohm"
        # "5 ohm"
        # "10 ohm"
        # "100 ohm"
        n470 = call-poly <vilib>:"DAQmx Create Virtual Channel.vi"("lines"=tag "Dev2/port0/line1") -> ("task out"=w992:refnum<k21>)  [unwired: 13 in, 1 out]
        n471 = call-poly <vilib>:"DAQmx Create Virtual Channel.vi"("lines"=tag "Dev2/port0/line0") -> ("task out"=w993:refnum<k21>)  [unwired: 13 in, 1 out]
        n472 = call-poly <vilib>:"DAQmx Create Virtual Channel.vi"("lines"=tag "Dev2/port0/line2") -> ("task out"=w991:refnum<k21>)  [unwired: 13 in, 1 out]
        n473 = call-poly <vilib>:"DAQmx Create Virtual Channel.vi"("lines"=tag "Dev2/port0/line3") -> ("task out"=w990:refnum<k21>)  [unwired: 13 in, 1 out]
        n474 = call-poly <vilib>:"DAQmx Create Virtual Channel.vi"("lines"=tag "Dev2/port0/line4") -> ("task out"=w989:refnum<k21>)  [unwired: 13 in, 1 out]
        n475 = call-poly <vilib>:"DAQmx Create Virtual Channel.vi"("lines"=tag "Dev2/port0/line6") -> ("task out"=w981:refnum<k21>)  [unwired: 13 in, 1 out]
        n476 = call-poly <vilib>:"DAQmx Create Virtual Channel.vi"("lines"=tag "Dev2/port0/line5") -> ("task out"=w988:refnum<k21>)  [unwired: 13 in, 1 out]
        n477 = call-poly <vilib>:"DAQmx Write.vi"("task/channels in"=w992, "data"=FALSE) -> ("task out"=w986:refnum<k21>)  [unwired: 11 in, 2 out]
        n478 = call-poly <vilib>:"DAQmx Write.vi"("task/channels in"=w991, "data"=FALSE) -> ("task out"=w985:refnum<k21>)  [unwired: 11 in, 2 out]
        n479 = call-poly <vilib>:"DAQmx Write.vi"("task/channels in"=w993, "data"=FALSE) -> ("task out"=w987:refnum<k21>)  [unwired: 11 in, 2 out]
        n480 = call-poly <vilib>:"DAQmx Write.vi"("task/channels in"=w990, "data"=FALSE) -> ("task out"=w984:refnum<k21>)  [unwired: 11 in, 2 out]
        n481 = call-poly <vilib>:"DAQmx Write.vi"("task/channels in"=w989, "data"=FALSE) -> ("task out"=w983:refnum<k21>)  [unwired: 11 in, 2 out]
        n482 = call-poly <vilib>:"DAQmx Write.vi"("task/channels in"=w981, "data"=FALSE) -> ("task out"=w978:refnum<k21>)  [unwired: 11 in, 2 out]
        n483 = call-poly <vilib>:"DAQmx Write.vi"("task/channels in"=w988, "data"=TRUE) -> ("task out"=w982:refnum<k21>)  [unwired: 11 in, 2 out]
      }
      frame ".0884" {
        # "No Resistor"
        # "30 ohm"
        # ".1 ohm"
        # "1 ohm"
        # "5 ohm"
        # "10 ohm"
        # "100 ohm"
        n484 = call-poly <vilib>:"DAQmx Create Virtual Channel.vi"("lines"=tag "Dev2/port0/line1") -> ("task out"=w1020:refnum<k21>)  [unwired: 13 in, 1 out]
        n485 = call-poly <vilib>:"DAQmx Create Virtual Channel.vi"("lines"=tag "Dev2/port0/line0") -> ("task out"=w1021:refnum<k21>)  [unwired: 13 in, 1 out]
        n486 = call-poly <vilib>:"DAQmx Create Virtual Channel.vi"("lines"=tag "Dev2/port0/line2") -> ("task out"=w1019:refnum<k21>)  [unwired: 13 in, 1 out]
        n487 = call-poly <vilib>:"DAQmx Create Virtual Channel.vi"("lines"=tag "Dev2/port0/line3") -> ("task out"=w1018:refnum<k21>)  [unwired: 13 in, 1 out]
        n488 = call-poly <vilib>:"DAQmx Create Virtual Channel.vi"("lines"=tag "Dev2/port0/line4") -> ("task out"=w1017:refnum<k21>)  [unwired: 13 in, 1 out]
        n489 = call-poly <vilib>:"DAQmx Create Virtual Channel.vi"("lines"=tag "Dev2/port0/line6") -> ("task out"=w1009:refnum<k21>)  [unwired: 13 in, 1 out]
        n490 = call-poly <vilib>:"DAQmx Create Virtual Channel.vi"("lines"=tag "Dev2/port0/line5") -> ("task out"=w1016:refnum<k21>)  [unwired: 13 in, 1 out]
        n491 = call-poly <vilib>:"DAQmx Write.vi"("task/channels in"=w1020, "data"=FALSE) -> ("task out"=w1014:refnum<k21>)  [unwired: 11 in, 2 out]
        n492 = call-poly <vilib>:"DAQmx Write.vi"("task/channels in"=w1019, "data"=FALSE) -> ("task out"=w1013:refnum<k21>)  [unwired: 11 in, 2 out]
        n493 = call-poly <vilib>:"DAQmx Write.vi"("task/channels in"=w1021, "data"=FALSE) -> ("task out"=w1015:refnum<k21>)  [unwired: 11 in, 2 out]
        n494 = call-poly <vilib>:"DAQmx Write.vi"("task/channels in"=w1018, "data"=FALSE) -> ("task out"=w1012:refnum<k21>)  [unwired: 11 in, 2 out]
        n495 = call-poly <vilib>:"DAQmx Write.vi"("task/channels in"=w1017, "data"=FALSE) -> ("task out"=w1011:refnum<k21>)  [unwired: 11 in, 2 out]
        n496 = call-poly <vilib>:"DAQmx Write.vi"("task/channels in"=w1009, "data"=FALSE) -> ("task out"=w1006:refnum<k21>)  [unwired: 11 in, 2 out]
        n497 = call-poly <vilib>:"DAQmx Write.vi"("task/channels in"=w1016, "data"=TRUE) -> ("task out"=w1010:refnum<k21>)  [unwired: 11 in, 2 out]
      }
      frame ".0885" {
        # "No Resistor"
        # "30 ohm"
        # ".1 ohm"
        # "1 ohm"
        # "5 ohm"
        # "10 ohm"
        # "100 ohm"
        n498 = call-poly <vilib>:"DAQmx Create Virtual Channel.vi"("lines"=tag "Dev2/port0/line1") -> ("task out"=w1048:refnum<k21>)  [unwired: 13 in, 1 out]
        n499 = call-poly <vilib>:"DAQmx Create Virtual Channel.vi"("lines"=tag "Dev2/port0/line0") -> ("task out"=w1049:refnum<k21>)  [unwired: 13 in, 1 out]
        n500 = call-poly <vilib>:"DAQmx Create Virtual Channel.vi"("lines"=tag "Dev2/port0/line2") -> ("task out"=w1047:refnum<k21>)  [unwired: 13 in, 1 out]
        n501 = call-poly <vilib>:"DAQmx Create Virtual Channel.vi"("lines"=tag "Dev2/port0/line3") -> ("task out"=w1046:refnum<k21>)  [unwired: 13 in, 1 out]
        n502 = call-poly <vilib>:"DAQmx Create Virtual Channel.vi"("lines"=tag "Dev2/port0/line4") -> ("task out"=w1045:refnum<k21>)  [unwired: 13 in, 1 out]
        n503 = call-poly <vilib>:"DAQmx Create Virtual Channel.vi"("lines"=tag "Dev2/port0/line6") -> ("task out"=w1037:refnum<k21>)  [unwired: 13 in, 1 out]
        n504 = call-poly <vilib>:"DAQmx Create Virtual Channel.vi"("lines"=tag "Dev2/port0/line5") -> ("task out"=w1044:refnum<k21>)  [unwired: 13 in, 1 out]
        n505 = call-poly <vilib>:"DAQmx Write.vi"("task/channels in"=w1048, "data"=FALSE) -> ("task out"=w1042:refnum<k21>)  [unwired: 11 in, 2 out]
        n506 = call-poly <vilib>:"DAQmx Write.vi"("task/channels in"=w1047, "data"=FALSE) -> ("task out"=w1041:refnum<k21>)  [unwired: 11 in, 2 out]
        n507 = call-poly <vilib>:"DAQmx Write.vi"("task/channels in"=w1049, "data"=FALSE) -> ("task out"=w1043:refnum<k21>)  [unwired: 11 in, 2 out]
        n508 = call-poly <vilib>:"DAQmx Write.vi"("task/channels in"=w1046, "data"=FALSE) -> ("task out"=w1040:refnum<k21>)  [unwired: 11 in, 2 out]
        n509 = call-poly <vilib>:"DAQmx Write.vi"("task/channels in"=w1045, "data"=FALSE) -> ("task out"=w1039:refnum<k21>)  [unwired: 11 in, 2 out]
        n510 = call-poly <vilib>:"DAQmx Write.vi"("task/channels in"=w1037, "data"=FALSE) -> ("task out"=w1034:refnum<k21>)  [unwired: 11 in, 2 out]
        n511 = call-poly <vilib>:"DAQmx Write.vi"("task/channels in"=w1044, "data"=TRUE) -> ("task out"=w1038:refnum<k21>)  [unwired: 11 in, 2 out]
      }
      frame ".0889" {
        # "No Resistor"
        # "30 ohm"
        # ".1 ohm"
        # "1 ohm"
        # "5 ohm"
        # "10 ohm"
        # "100 ohm"
        n512 = call-poly <vilib>:"DAQmx Create Virtual Channel.vi"("lines"=tag "Dev2/port0/line1") -> ("task out"=w1076:refnum<k21>)  [unwired: 13 in, 1 out]
        n513 = call-poly <vilib>:"DAQmx Create Virtual Channel.vi"("lines"=tag "Dev2/port0/line0") -> ("task out"=w1077:refnum<k21>)  [unwired: 13 in, 1 out]
        n514 = call-poly <vilib>:"DAQmx Create Virtual Channel.vi"("lines"=tag "Dev2/port0/line2") -> ("task out"=w1075:refnum<k21>)  [unwired: 13 in, 1 out]
        n515 = call-poly <vilib>:"DAQmx Create Virtual Channel.vi"("lines"=tag "Dev2/port0/line3") -> ("task out"=w1074:refnum<k21>)  [unwired: 13 in, 1 out]
        n516 = call-poly <vilib>:"DAQmx Create Virtual Channel.vi"("lines"=tag "Dev2/port0/line4") -> ("task out"=w1073:refnum<k21>)  [unwired: 13 in, 1 out]
        n517 = call-poly <vilib>:"DAQmx Create Virtual Channel.vi"("lines"=tag "Dev2/port0/line6") -> ("task out"=w1065:refnum<k21>)  [unwired: 13 in, 1 out]
        n518 = call-poly <vilib>:"DAQmx Create Virtual Channel.vi"("lines"=tag "Dev2/port0/line5") -> ("task out"=w1072:refnum<k21>)  [unwired: 13 in, 1 out]
        n519 = call-poly <vilib>:"DAQmx Write.vi"("task/channels in"=w1076, "data"=FALSE) -> ("task out"=w1070:refnum<k21>)  [unwired: 11 in, 2 out]
        n520 = call-poly <vilib>:"DAQmx Write.vi"("task/channels in"=w1075, "data"=FALSE) -> ("task out"=w1069:refnum<k21>)  [unwired: 11 in, 2 out]
        n521 = call-poly <vilib>:"DAQmx Write.vi"("task/channels in"=w1077, "data"=FALSE) -> ("task out"=w1071:refnum<k21>)  [unwired: 11 in, 2 out]
        n522 = call-poly <vilib>:"DAQmx Write.vi"("task/channels in"=w1074, "data"=FALSE) -> ("task out"=w1068:refnum<k21>)  [unwired: 11 in, 2 out]
        n523 = call-poly <vilib>:"DAQmx Write.vi"("task/channels in"=w1073, "data"=FALSE) -> ("task out"=w1067:refnum<k21>)  [unwired: 11 in, 2 out]
        n524 = call-poly <vilib>:"DAQmx Write.vi"("task/channels in"=w1065, "data"=FALSE) -> ("task out"=w1062:refnum<k21>)  [unwired: 11 in, 2 out]
        n525 = call-poly <vilib>:"DAQmx Write.vi"("task/channels in"=w1072, "data"=TRUE) -> ("task out"=w1066:refnum<k21>)  [unwired: 11 in, 2 out]
      }
      frame ".089" {
        # "No Resistor"
        # "30 ohm"
        # ".1 ohm"
        # "1 ohm"
        # "5 ohm"
        # "10 ohm"
        # "100 ohm"
        n526 = call-poly <vilib>:"DAQmx Create Virtual Channel.vi"("lines"=tag "Dev2/port0/line1") -> ("task out"=w1104:refnum<k21>)  [unwired: 13 in, 1 out]
        n527 = call-poly <vilib>:"DAQmx Create Virtual Channel.vi"("lines"=tag "Dev2/port0/line0") -> ("task out"=w1105:refnum<k21>)  [unwired: 13 in, 1 out]
        n528 = call-poly <vilib>:"DAQmx Create Virtual Channel.vi"("lines"=tag "Dev2/port0/line2") -> ("task out"=w1103:refnum<k21>)  [unwired: 13 in, 1 out]
        n529 = call-poly <vilib>:"DAQmx Create Virtual Channel.vi"("lines"=tag "Dev2/port0/line3") -> ("task out"=w1102:refnum<k21>)  [unwired: 13 in, 1 out]
        n530 = call-poly <vilib>:"DAQmx Create Virtual Channel.vi"("lines"=tag "Dev2/port0/line4") -> ("task out"=w1101:refnum<k21>)  [unwired: 13 in, 1 out]
        n531 = call-poly <vilib>:"DAQmx Create Virtual Channel.vi"("lines"=tag "Dev2/port0/line6") -> ("task out"=w1093:refnum<k21>)  [unwired: 13 in, 1 out]
        n532 = call-poly <vilib>:"DAQmx Create Virtual Channel.vi"("lines"=tag "Dev2/port0/line5") -> ("task out"=w1100:refnum<k21>)  [unwired: 13 in, 1 out]
        n533 = call-poly <vilib>:"DAQmx Write.vi"("task/channels in"=w1104, "data"=FALSE) -> ("task out"=w1098:refnum<k21>)  [unwired: 11 in, 2 out]
        n534 = call-poly <vilib>:"DAQmx Write.vi"("task/channels in"=w1103, "data"=FALSE) -> ("task out"=w1097:refnum<k21>)  [unwired: 11 in, 2 out]
        n535 = call-poly <vilib>:"DAQmx Write.vi"("task/channels in"=w1105, "data"=FALSE) -> ("task out"=w1099:refnum<k21>)  [unwired: 11 in, 2 out]
        n536 = call-poly <vilib>:"DAQmx Write.vi"("task/channels in"=w1102, "data"=FALSE) -> ("task out"=w1096:refnum<k21>)  [unwired: 11 in, 2 out]
        n537 = call-poly <vilib>:"DAQmx Write.vi"("task/channels in"=w1101, "data"=FALSE) -> ("task out"=w1095:refnum<k21>)  [unwired: 11 in, 2 out]
        n538 = call-poly <vilib>:"DAQmx Write.vi"("task/channels in"=w1093, "data"=FALSE) -> ("task out"=w1090:refnum<k21>)  [unwired: 11 in, 2 out]
        n539 = call-poly <vilib>:"DAQmx Write.vi"("task/channels in"=w1100, "data"=TRUE) -> ("task out"=w1094:refnum<k21>)  [unwired: 11 in, 2 out]
      }
      frame ".0892" {
        # "No Resistor"
        # "30 ohm"
        # ".1 ohm"
        # "1 ohm"
        # "5 ohm"
        # "10 ohm"
        # "100 ohm"
        n540 = call-poly <vilib>:"DAQmx Create Virtual Channel.vi"("lines"=tag "Dev2/port0/line1") -> ("task out"=w1132:refnum<k21>)  [unwired: 13 in, 1 out]
        n541 = call-poly <vilib>:"DAQmx Create Virtual Channel.vi"("lines"=tag "Dev2/port0/line0") -> ("task out"=w1133:refnum<k21>)  [unwired: 13 in, 1 out]
        n542 = call-poly <vilib>:"DAQmx Create Virtual Channel.vi"("lines"=tag "Dev2/port0/line2") -> ("task out"=w1131:refnum<k21>)  [unwired: 13 in, 1 out]
        n543 = call-poly <vilib>:"DAQmx Create Virtual Channel.vi"("lines"=tag "Dev2/port0/line3") -> ("task out"=w1130:refnum<k21>)  [unwired: 13 in, 1 out]
        n544 = call-poly <vilib>:"DAQmx Create Virtual Channel.vi"("lines"=tag "Dev2/port0/line4") -> ("task out"=w1129:refnum<k21>)  [unwired: 13 in, 1 out]
        n545 = call-poly <vilib>:"DAQmx Create Virtual Channel.vi"("lines"=tag "Dev2/port0/line6") -> ("task out"=w1121:refnum<k21>)  [unwired: 13 in, 1 out]
        n546 = call-poly <vilib>:"DAQmx Create Virtual Channel.vi"("lines"=tag "Dev2/port0/line5") -> ("task out"=w1128:refnum<k21>)  [unwired: 13 in, 1 out]
        n547 = call-poly <vilib>:"DAQmx Write.vi"("task/channels in"=w1132, "data"=FALSE) -> ("task out"=w1126:refnum<k21>)  [unwired: 11 in, 2 out]
        n548 = call-poly <vilib>:"DAQmx Write.vi"("task/channels in"=w1131, "data"=FALSE) -> ("task out"=w1125:refnum<k21>)  [unwired: 11 in, 2 out]
        n549 = call-poly <vilib>:"DAQmx Write.vi"("task/channels in"=w1133, "data"=FALSE) -> ("task out"=w1127:refnum<k21>)  [unwired: 11 in, 2 out]
        n550 = call-poly <vilib>:"DAQmx Write.vi"("task/channels in"=w1130, "data"=FALSE) -> ("task out"=w1124:refnum<k21>)  [unwired: 11 in, 2 out]
        n551 = call-poly <vilib>:"DAQmx Write.vi"("task/channels in"=w1129, "data"=FALSE) -> ("task out"=w1123:refnum<k21>)  [unwired: 11 in, 2 out]
        n552 = call-poly <vilib>:"DAQmx Write.vi"("task/channels in"=w1121, "data"=FALSE) -> ("task out"=w1118:refnum<k21>)  [unwired: 11 in, 2 out]
        n553 = call-poly <vilib>:"DAQmx Write.vi"("task/channels in"=w1128, "data"=TRUE) -> ("task out"=w1122:refnum<k21>)  [unwired: 11 in, 2 out]
      }
      frame ".0893" {
        # "No Resistor"
        # "30 ohm"
        # ".1 ohm"
        # "1 ohm"
        # "5 ohm"
        # "10 ohm"
        # "100 ohm"
        n554 = call-poly <vilib>:"DAQmx Create Virtual Channel.vi"("lines"=tag "Dev2/port0/line1") -> ("task out"=w1160:refnum<k21>)  [unwired: 13 in, 1 out]
        n555 = call-poly <vilib>:"DAQmx Create Virtual Channel.vi"("lines"=tag "Dev2/port0/line0") -> ("task out"=w1161:refnum<k21>)  [unwired: 13 in, 1 out]
        n556 = call-poly <vilib>:"DAQmx Create Virtual Channel.vi"("lines"=tag "Dev2/port0/line2") -> ("task out"=w1159:refnum<k21>)  [unwired: 13 in, 1 out]
        n557 = call-poly <vilib>:"DAQmx Create Virtual Channel.vi"("lines"=tag "Dev2/port0/line3") -> ("task out"=w1158:refnum<k21>)  [unwired: 13 in, 1 out]
        n558 = call-poly <vilib>:"DAQmx Create Virtual Channel.vi"("lines"=tag "Dev2/port0/line4") -> ("task out"=w1157:refnum<k21>)  [unwired: 13 in, 1 out]
        n559 = call-poly <vilib>:"DAQmx Create Virtual Channel.vi"("lines"=tag "Dev2/port0/line6") -> ("task out"=w1149:refnum<k21>)  [unwired: 13 in, 1 out]
        n560 = call-poly <vilib>:"DAQmx Create Virtual Channel.vi"("lines"=tag "Dev2/port0/line5") -> ("task out"=w1156:refnum<k21>)  [unwired: 13 in, 1 out]
        n561 = call-poly <vilib>:"DAQmx Write.vi"("task/channels in"=w1160, "data"=FALSE) -> ("task out"=w1154:refnum<k21>)  [unwired: 11 in, 2 out]
        n562 = call-poly <vilib>:"DAQmx Write.vi"("task/channels in"=w1159, "data"=FALSE) -> ("task out"=w1153:refnum<k21>)  [unwired: 11 in, 2 out]
        n563 = call-poly <vilib>:"DAQmx Write.vi"("task/channels in"=w1161, "data"=FALSE) -> ("task out"=w1155:refnum<k21>)  [unwired: 11 in, 2 out]
        n564 = call-poly <vilib>:"DAQmx Write.vi"("task/channels in"=w1158, "data"=FALSE) -> ("task out"=w1152:refnum<k21>)  [unwired: 11 in, 2 out]
        n565 = call-poly <vilib>:"DAQmx Write.vi"("task/channels in"=w1157, "data"=FALSE) -> ("task out"=w1151:refnum<k21>)  [unwired: 11 in, 2 out]
        n566 = call-poly <vilib>:"DAQmx Write.vi"("task/channels in"=w1149, "data"=FALSE) -> ("task out"=w1146:refnum<k21>)  [unwired: 11 in, 2 out]
        n567 = call-poly <vilib>:"DAQmx Write.vi"("task/channels in"=w1156, "data"=TRUE) -> ("task out"=w1150:refnum<k21>)  [unwired: 11 in, 2 out]
      }
      frame ".0897" {
        # "No Resistor"
        # "30 ohm"
        # ".1 ohm"
        # "1 ohm"
        # "5 ohm"
        # "10 ohm"
        # "100 ohm"
        n568 = call-poly <vilib>:"DAQmx Create Virtual Channel.vi"("lines"=tag "Dev2/port0/line1") -> ("task out"=w1188:refnum<k21>)  [unwired: 13 in, 1 out]
        n569 = call-poly <vilib>:"DAQmx Create Virtual Channel.vi"("lines"=tag "Dev2/port0/line0") -> ("task out"=w1189:refnum<k21>)  [unwired: 13 in, 1 out]
        n570 = call-poly <vilib>:"DAQmx Create Virtual Channel.vi"("lines"=tag "Dev2/port0/line2") -> ("task out"=w1187:refnum<k21>)  [unwired: 13 in, 1 out]
        n571 = call-poly <vilib>:"DAQmx Create Virtual Channel.vi"("lines"=tag "Dev2/port0/line3") -> ("task out"=w1186:refnum<k21>)  [unwired: 13 in, 1 out]
        n572 = call-poly <vilib>:"DAQmx Create Virtual Channel.vi"("lines"=tag "Dev2/port0/line4") -> ("task out"=w1185:refnum<k21>)  [unwired: 13 in, 1 out]
        n573 = call-poly <vilib>:"DAQmx Create Virtual Channel.vi"("lines"=tag "Dev2/port0/line6") -> ("task out"=w1177:refnum<k21>)  [unwired: 13 in, 1 out]
        n574 = call-poly <vilib>:"DAQmx Create Virtual Channel.vi"("lines"=tag "Dev2/port0/line5") -> ("task out"=w1184:refnum<k21>)  [unwired: 13 in, 1 out]
        n575 = call-poly <vilib>:"DAQmx Write.vi"("task/channels in"=w1188, "data"=FALSE) -> ("task out"=w1182:refnum<k21>)  [unwired: 11 in, 2 out]
        n576 = call-poly <vilib>:"DAQmx Write.vi"("task/channels in"=w1187, "data"=FALSE) -> ("task out"=w1181:refnum<k21>)  [unwired: 11 in, 2 out]
        n577 = call-poly <vilib>:"DAQmx Write.vi"("task/channels in"=w1189, "data"=FALSE) -> ("task out"=w1183:refnum<k21>)  [unwired: 11 in, 2 out]
        n578 = call-poly <vilib>:"DAQmx Write.vi"("task/channels in"=w1186, "data"=FALSE) -> ("task out"=w1180:refnum<k21>)  [unwired: 11 in, 2 out]
        n579 = call-poly <vilib>:"DAQmx Write.vi"("task/channels in"=w1185, "data"=FALSE) -> ("task out"=w1179:refnum<k21>)  [unwired: 11 in, 2 out]
        n580 = call-poly <vilib>:"DAQmx Write.vi"("task/channels in"=w1177, "data"=FALSE) -> ("task out"=w1174:refnum<k21>)  [unwired: 11 in, 2 out]
        n581 = call-poly <vilib>:"DAQmx Write.vi"("task/channels in"=w1184, "data"=TRUE) -> ("task out"=w1178:refnum<k21>)  [unwired: 11 in, 2 out]
      }
      frame ".0898" {
        # "No Resistor"
        # "30 ohm"
        # ".1 ohm"
        # "1 ohm"
        # "5 ohm"
        # "10 ohm"
        # "100 ohm"
        n582 = call-poly <vilib>:"DAQmx Create Virtual Channel.vi"("lines"=tag "Dev2/port0/line1") -> ("task out"=w1216:refnum<k21>)  [unwired: 13 in, 1 out]
        n583 = call-poly <vilib>:"DAQmx Create Virtual Channel.vi"("lines"=tag "Dev2/port0/line0") -> ("task out"=w1217:refnum<k21>)  [unwired: 13 in, 1 out]
        n584 = call-poly <vilib>:"DAQmx Create Virtual Channel.vi"("lines"=tag "Dev2/port0/line2") -> ("task out"=w1215:refnum<k21>)  [unwired: 13 in, 1 out]
        n585 = call-poly <vilib>:"DAQmx Create Virtual Channel.vi"("lines"=tag "Dev2/port0/line3") -> ("task out"=w1214:refnum<k21>)  [unwired: 13 in, 1 out]
        n586 = call-poly <vilib>:"DAQmx Create Virtual Channel.vi"("lines"=tag "Dev2/port0/line4") -> ("task out"=w1213:refnum<k21>)  [unwired: 13 in, 1 out]
        n587 = call-poly <vilib>:"DAQmx Create Virtual Channel.vi"("lines"=tag "Dev2/port0/line6") -> ("task out"=w1205:refnum<k21>)  [unwired: 13 in, 1 out]
        n588 = call-poly <vilib>:"DAQmx Create Virtual Channel.vi"("lines"=tag "Dev2/port0/line5") -> ("task out"=w1212:refnum<k21>)  [unwired: 13 in, 1 out]
        n589 = call-poly <vilib>:"DAQmx Write.vi"("task/channels in"=w1216, "data"=FALSE) -> ("task out"=w1210:refnum<k21>)  [unwired: 11 in, 2 out]
        n590 = call-poly <vilib>:"DAQmx Write.vi"("task/channels in"=w1215, "data"=FALSE) -> ("task out"=w1209:refnum<k21>)  [unwired: 11 in, 2 out]
        n591 = call-poly <vilib>:"DAQmx Write.vi"("task/channels in"=w1217, "data"=FALSE) -> ("task out"=w1211:refnum<k21>)  [unwired: 11 in, 2 out]
        n592 = call-poly <vilib>:"DAQmx Write.vi"("task/channels in"=w1214, "data"=FALSE) -> ("task out"=w1208:refnum<k21>)  [unwired: 11 in, 2 out]
        n593 = call-poly <vilib>:"DAQmx Write.vi"("task/channels in"=w1213, "data"=FALSE) -> ("task out"=w1207:refnum<k21>)  [unwired: 11 in, 2 out]
        n594 = call-poly <vilib>:"DAQmx Write.vi"("task/channels in"=w1205, "data"=FALSE) -> ("task out"=w1202:refnum<k21>)  [unwired: 11 in, 2 out]
        n595 = call-poly <vilib>:"DAQmx Write.vi"("task/channels in"=w1212, "data"=TRUE) -> ("task out"=w1206:refnum<k21>)  [unwired: 11 in, 2 out]
      }
      frame ".09" {
        # "No Resistor"
        # "30 ohm"
        # ".1 ohm"
        # "1 ohm"
        # "5 ohm"
        # "10 ohm"
        # "100 ohm"
        n596 = call-poly <vilib>:"DAQmx Create Virtual Channel.vi"("lines"=tag "Dev2/port0/line1") -> ("task out"=w1244:refnum<k21>)  [unwired: 13 in, 1 out]
        n597 = call-poly <vilib>:"DAQmx Create Virtual Channel.vi"("lines"=tag "Dev2/port0/line0") -> ("task out"=w1245:refnum<k21>)  [unwired: 13 in, 1 out]
        n598 = call-poly <vilib>:"DAQmx Create Virtual Channel.vi"("lines"=tag "Dev2/port0/line2") -> ("task out"=w1243:refnum<k21>)  [unwired: 13 in, 1 out]
        n599 = call-poly <vilib>:"DAQmx Create Virtual Channel.vi"("lines"=tag "Dev2/port0/line3") -> ("task out"=w1242:refnum<k21>)  [unwired: 13 in, 1 out]
        n600 = call-poly <vilib>:"DAQmx Create Virtual Channel.vi"("lines"=tag "Dev2/port0/line4") -> ("task out"=w1241:refnum<k21>)  [unwired: 13 in, 1 out]
        n601 = call-poly <vilib>:"DAQmx Create Virtual Channel.vi"("lines"=tag "Dev2/port0/line6") -> ("task out"=w1233:refnum<k21>)  [unwired: 13 in, 1 out]
        n602 = call-poly <vilib>:"DAQmx Create Virtual Channel.vi"("lines"=tag "Dev2/port0/line5") -> ("task out"=w1240:refnum<k21>)  [unwired: 13 in, 1 out]
        n603 = call-poly <vilib>:"DAQmx Write.vi"("task/channels in"=w1244, "data"=FALSE) -> ("task out"=w1238:refnum<k21>)  [unwired: 11 in, 2 out]
        n604 = call-poly <vilib>:"DAQmx Write.vi"("task/channels in"=w1243, "data"=FALSE) -> ("task out"=w1237:refnum<k21>)  [unwired: 11 in, 2 out]
        n605 = call-poly <vilib>:"DAQmx Write.vi"("task/channels in"=w1245, "data"=FALSE) -> ("task out"=w1239:refnum<k21>)  [unwired: 11 in, 2 out]
        n606 = call-poly <vilib>:"DAQmx Write.vi"("task/channels in"=w1242, "data"=FALSE) -> ("task out"=w1236:refnum<k21>)  [unwired: 11 in, 2 out]
        n607 = call-poly <vilib>:"DAQmx Write.vi"("task/channels in"=w1241, "data"=FALSE) -> ("task out"=w1235:refnum<k21>)  [unwired: 11 in, 2 out]
        n608 = call-poly <vilib>:"DAQmx Write.vi"("task/channels in"=w1233, "data"=FALSE) -> ("task out"=w1230:refnum<k21>)  [unwired: 11 in, 2 out]
        n609 = call-poly <vilib>:"DAQmx Write.vi"("task/channels in"=w1240, "data"=TRUE) -> ("task out"=w1234:refnum<k21>)  [unwired: 11 in, 2 out]
      }
      frame ".0901" {
        # "No Resistor"
        # "30 ohm"
        # ".1 ohm"
        # "1 ohm"
        # "5 ohm"
        # "10 ohm"
        # "100 ohm"
        n610 = call-poly <vilib>:"DAQmx Create Virtual Channel.vi"("lines"=tag "Dev2/port0/line1") -> ("task out"=w1272:refnum<k21>)  [unwired: 13 in, 1 out]
        n611 = call-poly <vilib>:"DAQmx Create Virtual Channel.vi"("lines"=tag "Dev2/port0/line0") -> ("task out"=w1273:refnum<k21>)  [unwired: 13 in, 1 out]
        n612 = call-poly <vilib>:"DAQmx Create Virtual Channel.vi"("lines"=tag "Dev2/port0/line2") -> ("task out"=w1271:refnum<k21>)  [unwired: 13 in, 1 out]
        n613 = call-poly <vilib>:"DAQmx Create Virtual Channel.vi"("lines"=tag "Dev2/port0/line3") -> ("task out"=w1270:refnum<k21>)  [unwired: 13 in, 1 out]
        n614 = call-poly <vilib>:"DAQmx Create Virtual Channel.vi"("lines"=tag "Dev2/port0/line4") -> ("task out"=w1269:refnum<k21>)  [unwired: 13 in, 1 out]
        n615 = call-poly <vilib>:"DAQmx Create Virtual Channel.vi"("lines"=tag "Dev2/port0/line6") -> ("task out"=w1261:refnum<k21>)  [unwired: 13 in, 1 out]
        n616 = call-poly <vilib>:"DAQmx Create Virtual Channel.vi"("lines"=tag "Dev2/port0/line5") -> ("task out"=w1268:refnum<k21>)  [unwired: 13 in, 1 out]
        n617 = call-poly <vilib>:"DAQmx Write.vi"("task/channels in"=w1272, "data"=FALSE) -> ("task out"=w1266:refnum<k21>)  [unwired: 11 in, 2 out]
        n618 = call-poly <vilib>:"DAQmx Write.vi"("task/channels in"=w1271, "data"=FALSE) -> ("task out"=w1265:refnum<k21>)  [unwired: 11 in, 2 out]
        n619 = call-poly <vilib>:"DAQmx Write.vi"("task/channels in"=w1273, "data"=FALSE) -> ("task out"=w1267:refnum<k21>)  [unwired: 11 in, 2 out]
        n620 = call-poly <vilib>:"DAQmx Write.vi"("task/channels in"=w1270, "data"=FALSE) -> ("task out"=w1264:refnum<k21>)  [unwired: 11 in, 2 out]
        n621 = call-poly <vilib>:"DAQmx Write.vi"("task/channels in"=w1269, "data"=FALSE) -> ("task out"=w1263:refnum<k21>)  [unwired: 11 in, 2 out]
        n622 = call-poly <vilib>:"DAQmx Write.vi"("task/channels in"=w1261, "data"=FALSE) -> ("task out"=w1258:refnum<k21>)  [unwired: 11 in, 2 out]
        n623 = call-poly <vilib>:"DAQmx Write.vi"("task/channels in"=w1268, "data"=TRUE) -> ("task out"=w1262:refnum<k21>)  [unwired: 11 in, 2 out]
      }
      frame ".0906" {
        # "No Resistor"
        # "30 ohm"
        # ".1 ohm"
        # "1 ohm"
        # "5 ohm"
        # "10 ohm"
        # "100 ohm"
        n624 = call-poly <vilib>:"DAQmx Create Virtual Channel.vi"("lines"=tag "Dev2/port0/line1") -> ("task out"=w1300:refnum<k21>)  [unwired: 13 in, 1 out]
        n625 = call-poly <vilib>:"DAQmx Create Virtual Channel.vi"("lines"=tag "Dev2/port0/line0") -> ("task out"=w1301:refnum<k21>)  [unwired: 13 in, 1 out]
        n626 = call-poly <vilib>:"DAQmx Create Virtual Channel.vi"("lines"=tag "Dev2/port0/line2") -> ("task out"=w1299:refnum<k21>)  [unwired: 13 in, 1 out]
        n627 = call-poly <vilib>:"DAQmx Create Virtual Channel.vi"("lines"=tag "Dev2/port0/line3") -> ("task out"=w1298:refnum<k21>)  [unwired: 13 in, 1 out]
        n628 = call-poly <vilib>:"DAQmx Create Virtual Channel.vi"("lines"=tag "Dev2/port0/line4") -> ("task out"=w1297:refnum<k21>)  [unwired: 13 in, 1 out]
        n629 = call-poly <vilib>:"DAQmx Create Virtual Channel.vi"("lines"=tag "Dev2/port0/line6") -> ("task out"=w1289:refnum<k21>)  [unwired: 13 in, 1 out]
        n630 = call-poly <vilib>:"DAQmx Create Virtual Channel.vi"("lines"=tag "Dev2/port0/line5") -> ("task out"=w1296:refnum<k21>)  [unwired: 13 in, 1 out]
        n631 = call-poly <vilib>:"DAQmx Write.vi"("task/channels in"=w1300, "data"=FALSE) -> ("task out"=w1294:refnum<k21>)  [unwired: 11 in, 2 out]
        n632 = call-poly <vilib>:"DAQmx Write.vi"("task/channels in"=w1299, "data"=FALSE) -> ("task out"=w1293:refnum<k21>)  [unwired: 11 in, 2 out]
        n633 = call-poly <vilib>:"DAQmx Write.vi"("task/channels in"=w1301, "data"=FALSE) -> ("task out"=w1295:refnum<k21>)  [unwired: 11 in, 2 out]
        n634 = call-poly <vilib>:"DAQmx Write.vi"("task/channels in"=w1298, "data"=FALSE) -> ("task out"=w1292:refnum<k21>)  [unwired: 11 in, 2 out]
        n635 = call-poly <vilib>:"DAQmx Write.vi"("task/channels in"=w1297, "data"=FALSE) -> ("task out"=w1291:refnum<k21>)  [unwired: 11 in, 2 out]
        n636 = call-poly <vilib>:"DAQmx Write.vi"("task/channels in"=w1289, "data"=FALSE) -> ("task out"=w1286:refnum<k21>)  [unwired: 11 in, 2 out]
        n637 = call-poly <vilib>:"DAQmx Write.vi"("task/channels in"=w1296, "data"=TRUE) -> ("task out"=w1290:refnum<k21>)  [unwired: 11 in, 2 out]
      }
      frame ".0908" {
        # "No Resistor"
        # "30 ohm"
        # ".1 ohm"
        # "1 ohm"
        # "5 ohm"
        # "10 ohm"
        # "100 ohm"
        n638 = call-poly <vilib>:"DAQmx Create Virtual Channel.vi"("lines"=tag "Dev2/port0/line1") -> ("task out"=w1328:refnum<k21>)  [unwired: 13 in, 1 out]
        n639 = call-poly <vilib>:"DAQmx Create Virtual Channel.vi"("lines"=tag "Dev2/port0/line0") -> ("task out"=w1329:refnum<k21>)  [unwired: 13 in, 1 out]
        n640 = call-poly <vilib>:"DAQmx Create Virtual Channel.vi"("lines"=tag "Dev2/port0/line2") -> ("task out"=w1327:refnum<k21>)  [unwired: 13 in, 1 out]
        n641 = call-poly <vilib>:"DAQmx Create Virtual Channel.vi"("lines"=tag "Dev2/port0/line3") -> ("task out"=w1326:refnum<k21>)  [unwired: 13 in, 1 out]
        n642 = call-poly <vilib>:"DAQmx Create Virtual Channel.vi"("lines"=tag "Dev2/port0/line4") -> ("task out"=w1325:refnum<k21>)  [unwired: 13 in, 1 out]
        n643 = call-poly <vilib>:"DAQmx Create Virtual Channel.vi"("lines"=tag "Dev2/port0/line6") -> ("task out"=w1317:refnum<k21>)  [unwired: 13 in, 1 out]
        n644 = call-poly <vilib>:"DAQmx Create Virtual Channel.vi"("lines"=tag "Dev2/port0/line5") -> ("task out"=w1324:refnum<k21>)  [unwired: 13 in, 1 out]
        n645 = call-poly <vilib>:"DAQmx Write.vi"("task/channels in"=w1328, "data"=FALSE) -> ("task out"=w1322:refnum<k21>)  [unwired: 11 in, 2 out]
        n646 = call-poly <vilib>:"DAQmx Write.vi"("task/channels in"=w1327, "data"=FALSE) -> ("task out"=w1321:refnum<k21>)  [unwired: 11 in, 2 out]
        n647 = call-poly <vilib>:"DAQmx Write.vi"("task/channels in"=w1329, "data"=FALSE) -> ("task out"=w1323:refnum<k21>)  [unwired: 11 in, 2 out]
        n648 = call-poly <vilib>:"DAQmx Write.vi"("task/channels in"=w1326, "data"=FALSE) -> ("task out"=w1320:refnum<k21>)  [unwired: 11 in, 2 out]
        n649 = call-poly <vilib>:"DAQmx Write.vi"("task/channels in"=w1325, "data"=FALSE) -> ("task out"=w1319:refnum<k21>)  [unwired: 11 in, 2 out]
        n650 = call-poly <vilib>:"DAQmx Write.vi"("task/channels in"=w1317, "data"=FALSE) -> ("task out"=w1314:refnum<k21>)  [unwired: 11 in, 2 out]
        n651 = call-poly <vilib>:"DAQmx Write.vi"("task/channels in"=w1324, "data"=TRUE) -> ("task out"=w1318:refnum<k21>)  [unwired: 11 in, 2 out]
      }
      frame ".0909" {
        # "No Resistor"
        # "30 ohm"
        # ".1 ohm"
        # "1 ohm"
        # "5 ohm"
        # "10 ohm"
        # "100 ohm"
        n652 = call-poly <vilib>:"DAQmx Create Virtual Channel.vi"("lines"=tag "Dev2/port0/line1") -> ("task out"=w1356:refnum<k21>)  [unwired: 13 in, 1 out]
        n653 = call-poly <vilib>:"DAQmx Create Virtual Channel.vi"("lines"=tag "Dev2/port0/line0") -> ("task out"=w1357:refnum<k21>)  [unwired: 13 in, 1 out]
        n654 = call-poly <vilib>:"DAQmx Create Virtual Channel.vi"("lines"=tag "Dev2/port0/line2") -> ("task out"=w1355:refnum<k21>)  [unwired: 13 in, 1 out]
        n655 = call-poly <vilib>:"DAQmx Create Virtual Channel.vi"("lines"=tag "Dev2/port0/line3") -> ("task out"=w1354:refnum<k21>)  [unwired: 13 in, 1 out]
        n656 = call-poly <vilib>:"DAQmx Create Virtual Channel.vi"("lines"=tag "Dev2/port0/line4") -> ("task out"=w1353:refnum<k21>)  [unwired: 13 in, 1 out]
        n657 = call-poly <vilib>:"DAQmx Create Virtual Channel.vi"("lines"=tag "Dev2/port0/line6") -> ("task out"=w1345:refnum<k21>)  [unwired: 13 in, 1 out]
        n658 = call-poly <vilib>:"DAQmx Create Virtual Channel.vi"("lines"=tag "Dev2/port0/line5") -> ("task out"=w1352:refnum<k21>)  [unwired: 13 in, 1 out]
        n659 = call-poly <vilib>:"DAQmx Write.vi"("task/channels in"=w1356, "data"=FALSE) -> ("task out"=w1350:refnum<k21>)  [unwired: 11 in, 2 out]
        n660 = call-poly <vilib>:"DAQmx Write.vi"("task/channels in"=w1355, "data"=FALSE) -> ("task out"=w1349:refnum<k21>)  [unwired: 11 in, 2 out]
        n661 = call-poly <vilib>:"DAQmx Write.vi"("task/channels in"=w1357, "data"=FALSE) -> ("task out"=w1351:refnum<k21>)  [unwired: 11 in, 2 out]
        n662 = call-poly <vilib>:"DAQmx Write.vi"("task/channels in"=w1354, "data"=FALSE) -> ("task out"=w1348:refnum<k21>)  [unwired: 11 in, 2 out]
        n663 = call-poly <vilib>:"DAQmx Write.vi"("task/channels in"=w1353, "data"=FALSE) -> ("task out"=w1347:refnum<k21>)  [unwired: 11 in, 2 out]
        n664 = call-poly <vilib>:"DAQmx Write.vi"("task/channels in"=w1345, "data"=FALSE) -> ("task out"=w1342:refnum<k21>)  [unwired: 11 in, 2 out]
        n665 = call-poly <vilib>:"DAQmx Write.vi"("task/channels in"=w1352, "data"=TRUE) -> ("task out"=w1346:refnum<k21>)  [unwired: 11 in, 2 out]
      }
      frame ".0967" {
        # "No Resistor"
        # "30 ohm"
        # ".1 ohm"
        # "1 ohm"
        # "5 ohm"
        # "10 ohm"
        # "100 ohm"
        n666 = call-poly <vilib>:"DAQmx Create Virtual Channel.vi"("lines"=tag "Dev2/port0/line1") -> ("task out"=w1384:refnum<k21>)  [unwired: 13 in, 1 out]
        n667 = call-poly <vilib>:"DAQmx Create Virtual Channel.vi"("lines"=tag "Dev2/port0/line0") -> ("task out"=w1385:refnum<k21>)  [unwired: 13 in, 1 out]
        n668 = call-poly <vilib>:"DAQmx Create Virtual Channel.vi"("lines"=tag "Dev2/port0/line2") -> ("task out"=w1383:refnum<k21>)  [unwired: 13 in, 1 out]
        n669 = call-poly <vilib>:"DAQmx Create Virtual Channel.vi"("lines"=tag "Dev2/port0/line3") -> ("task out"=w1382:refnum<k21>)  [unwired: 13 in, 1 out]
        n670 = call-poly <vilib>:"DAQmx Create Virtual Channel.vi"("lines"=tag "Dev2/port0/line4") -> ("task out"=w1381:refnum<k21>)  [unwired: 13 in, 1 out]
        n671 = call-poly <vilib>:"DAQmx Create Virtual Channel.vi"("lines"=tag "Dev2/port0/line6") -> ("task out"=w1373:refnum<k21>)  [unwired: 13 in, 1 out]
        n672 = call-poly <vilib>:"DAQmx Create Virtual Channel.vi"("lines"=tag "Dev2/port0/line5") -> ("task out"=w1380:refnum<k21>)  [unwired: 13 in, 1 out]
        n673 = call-poly <vilib>:"DAQmx Write.vi"("task/channels in"=w1384, "data"=FALSE) -> ("task out"=w1378:refnum<k21>)  [unwired: 11 in, 2 out]
        n674 = call-poly <vilib>:"DAQmx Write.vi"("task/channels in"=w1383, "data"=FALSE) -> ("task out"=w1377:refnum<k21>)  [unwired: 11 in, 2 out]
        n675 = call-poly <vilib>:"DAQmx Write.vi"("task/channels in"=w1385, "data"=FALSE) -> ("task out"=w1379:refnum<k21>)  [unwired: 11 in, 2 out]
        n676 = call-poly <vilib>:"DAQmx Write.vi"("task/channels in"=w1382, "data"=FALSE) -> ("task out"=w1376:refnum<k21>)  [unwired: 11 in, 2 out]
        n677 = call-poly <vilib>:"DAQmx Write.vi"("task/channels in"=w1381, "data"=FALSE) -> ("task out"=w1375:refnum<k21>)  [unwired: 11 in, 2 out]
        n678 = call-poly <vilib>:"DAQmx Write.vi"("task/channels in"=w1373, "data"=FALSE) -> ("task out"=w1370:refnum<k21>)  [unwired: 11 in, 2 out]
        n679 = call-poly <vilib>:"DAQmx Write.vi"("task/channels in"=w1380, "data"=TRUE) -> ("task out"=w1374:refnum<k21>)  [unwired: 11 in, 2 out]
      }
      frame ".0968" {
        # "No Resistor"
        # "30 ohm"
        # ".1 ohm"
        # "1 ohm"
        # "5 ohm"
        # "10 ohm"
        # "100 ohm"
        n680 = call-poly <vilib>:"DAQmx Create Virtual Channel.vi"("lines"=tag "Dev2/port0/line1") -> ("task out"=w1412:refnum<k21>)  [unwired: 13 in, 1 out]
        n681 = call-poly <vilib>:"DAQmx Create Virtual Channel.vi"("lines"=tag "Dev2/port0/line0") -> ("task out"=w1413:refnum<k21>)  [unwired: 13 in, 1 out]
        n682 = call-poly <vilib>:"DAQmx Create Virtual Channel.vi"("lines"=tag "Dev2/port0/line2") -> ("task out"=w1411:refnum<k21>)  [unwired: 13 in, 1 out]
        n683 = call-poly <vilib>:"DAQmx Create Virtual Channel.vi"("lines"=tag "Dev2/port0/line3") -> ("task out"=w1410:refnum<k21>)  [unwired: 13 in, 1 out]
        n684 = call-poly <vilib>:"DAQmx Create Virtual Channel.vi"("lines"=tag "Dev2/port0/line4") -> ("task out"=w1409:refnum<k21>)  [unwired: 13 in, 1 out]
        n685 = call-poly <vilib>:"DAQmx Create Virtual Channel.vi"("lines"=tag "Dev2/port0/line6") -> ("task out"=w1401:refnum<k21>)  [unwired: 13 in, 1 out]
        n686 = call-poly <vilib>:"DAQmx Create Virtual Channel.vi"("lines"=tag "Dev2/port0/line5") -> ("task out"=w1408:refnum<k21>)  [unwired: 13 in, 1 out]
        n687 = call-poly <vilib>:"DAQmx Write.vi"("task/channels in"=w1412, "data"=FALSE) -> ("task out"=w1406:refnum<k21>)  [unwired: 11 in, 2 out]
        n688 = call-poly <vilib>:"DAQmx Write.vi"("task/channels in"=w1411, "data"=FALSE) -> ("task out"=w1405:refnum<k21>)  [unwired: 11 in, 2 out]
        n689 = call-poly <vilib>:"DAQmx Write.vi"("task/channels in"=w1413, "data"=FALSE) -> ("task out"=w1407:refnum<k21>)  [unwired: 11 in, 2 out]
        n690 = call-poly <vilib>:"DAQmx Write.vi"("task/channels in"=w1410, "data"=FALSE) -> ("task out"=w1404:refnum<k21>)  [unwired: 11 in, 2 out]
        n691 = call-poly <vilib>:"DAQmx Write.vi"("task/channels in"=w1409, "data"=FALSE) -> ("task out"=w1403:refnum<k21>)  [unwired: 11 in, 2 out]
        n692 = call-poly <vilib>:"DAQmx Write.vi"("task/channels in"=w1401, "data"=FALSE) -> ("task out"=w1398:refnum<k21>)  [unwired: 11 in, 2 out]
        n693 = call-poly <vilib>:"DAQmx Write.vi"("task/channels in"=w1408, "data"=TRUE) -> ("task out"=w1402:refnum<k21>)  [unwired: 11 in, 2 out]
      }
      frame ".097" {
        # "No Resistor"
        # "30 ohm"
        # ".1 ohm"
        # "1 ohm"
        # "5 ohm"
        # "10 ohm"
        # "100 ohm"
        n694 = call-poly <vilib>:"DAQmx Create Virtual Channel.vi"("lines"=tag "Dev2/port0/line1") -> ("task out"=w1440:refnum<k21>)  [unwired: 13 in, 1 out]
        n695 = call-poly <vilib>:"DAQmx Create Virtual Channel.vi"("lines"=tag "Dev2/port0/line0") -> ("task out"=w1441:refnum<k21>)  [unwired: 13 in, 1 out]
        n696 = call-poly <vilib>:"DAQmx Create Virtual Channel.vi"("lines"=tag "Dev2/port0/line2") -> ("task out"=w1439:refnum<k21>)  [unwired: 13 in, 1 out]
        n697 = call-poly <vilib>:"DAQmx Create Virtual Channel.vi"("lines"=tag "Dev2/port0/line3") -> ("task out"=w1438:refnum<k21>)  [unwired: 13 in, 1 out]
        n698 = call-poly <vilib>:"DAQmx Create Virtual Channel.vi"("lines"=tag "Dev2/port0/line4") -> ("task out"=w1437:refnum<k21>)  [unwired: 13 in, 1 out]
        n699 = call-poly <vilib>:"DAQmx Create Virtual Channel.vi"("lines"=tag "Dev2/port0/line6") -> ("task out"=w1429:refnum<k21>)  [unwired: 13 in, 1 out]
        n700 = call-poly <vilib>:"DAQmx Create Virtual Channel.vi"("lines"=tag "Dev2/port0/line5") -> ("task out"=w1436:refnum<k21>)  [unwired: 13 in, 1 out]
        n701 = call-poly <vilib>:"DAQmx Write.vi"("task/channels in"=w1440, "data"=FALSE) -> ("task out"=w1434:refnum<k21>)  [unwired: 11 in, 2 out]
        n702 = call-poly <vilib>:"DAQmx Write.vi"("task/channels in"=w1439, "data"=FALSE) -> ("task out"=w1433:refnum<k21>)  [unwired: 11 in, 2 out]
        n703 = call-poly <vilib>:"DAQmx Write.vi"("task/channels in"=w1441, "data"=FALSE) -> ("task out"=w1435:refnum<k21>)  [unwired: 11 in, 2 out]
        n704 = call-poly <vilib>:"DAQmx Write.vi"("task/channels in"=w1438, "data"=FALSE) -> ("task out"=w1432:refnum<k21>)  [unwired: 11 in, 2 out]
        n705 = call-poly <vilib>:"DAQmx Write.vi"("task/channels in"=w1437, "data"=FALSE) -> ("task out"=w1431:refnum<k21>)  [unwired: 11 in, 2 out]
        n706 = call-poly <vilib>:"DAQmx Write.vi"("task/channels in"=w1429, "data"=FALSE) -> ("task out"=w1426:refnum<k21>)  [unwired: 11 in, 2 out]
        n707 = call-poly <vilib>:"DAQmx Write.vi"("task/channels in"=w1436, "data"=TRUE) -> ("task out"=w1430:refnum<k21>)  [unwired: 11 in, 2 out]
      }
      frame ".0971" {
        # "No Resistor"
        # "30 ohm"
        # ".1 ohm"
        # "1 ohm"
        # "5 ohm"
        # "10 ohm"
        # "100 ohm"
        n708 = call-poly <vilib>:"DAQmx Create Virtual Channel.vi"("lines"=tag "Dev2/port0/line1") -> ("task out"=w1468:refnum<k21>)  [unwired: 13 in, 1 out]
        n709 = call-poly <vilib>:"DAQmx Create Virtual Channel.vi"("lines"=tag "Dev2/port0/line0") -> ("task out"=w1469:refnum<k21>)  [unwired: 13 in, 1 out]
        n710 = call-poly <vilib>:"DAQmx Create Virtual Channel.vi"("lines"=tag "Dev2/port0/line2") -> ("task out"=w1467:refnum<k21>)  [unwired: 13 in, 1 out]
        n711 = call-poly <vilib>:"DAQmx Create Virtual Channel.vi"("lines"=tag "Dev2/port0/line3") -> ("task out"=w1466:refnum<k21>)  [unwired: 13 in, 1 out]
        n712 = call-poly <vilib>:"DAQmx Create Virtual Channel.vi"("lines"=tag "Dev2/port0/line4") -> ("task out"=w1465:refnum<k21>)  [unwired: 13 in, 1 out]
        n713 = call-poly <vilib>:"DAQmx Create Virtual Channel.vi"("lines"=tag "Dev2/port0/line6") -> ("task out"=w1457:refnum<k21>)  [unwired: 13 in, 1 out]
        n714 = call-poly <vilib>:"DAQmx Create Virtual Channel.vi"("lines"=tag "Dev2/port0/line5") -> ("task out"=w1464:refnum<k21>)  [unwired: 13 in, 1 out]
        n715 = call-poly <vilib>:"DAQmx Write.vi"("task/channels in"=w1468, "data"=FALSE) -> ("task out"=w1462:refnum<k21>)  [unwired: 11 in, 2 out]
        n716 = call-poly <vilib>:"DAQmx Write.vi"("task/channels in"=w1467, "data"=FALSE) -> ("task out"=w1461:refnum<k21>)  [unwired: 11 in, 2 out]
        n717 = call-poly <vilib>:"DAQmx Write.vi"("task/channels in"=w1469, "data"=FALSE) -> ("task out"=w1463:refnum<k21>)  [unwired: 11 in, 2 out]
        n718 = call-poly <vilib>:"DAQmx Write.vi"("task/channels in"=w1466, "data"=FALSE) -> ("task out"=w1460:refnum<k21>)  [unwired: 11 in, 2 out]
        n719 = call-poly <vilib>:"DAQmx Write.vi"("task/channels in"=w1465, "data"=FALSE) -> ("task out"=w1459:refnum<k21>)  [unwired: 11 in, 2 out]
        n720 = call-poly <vilib>:"DAQmx Write.vi"("task/channels in"=w1457, "data"=FALSE) -> ("task out"=w1454:refnum<k21>)  [unwired: 11 in, 2 out]
        n721 = call-poly <vilib>:"DAQmx Write.vi"("task/channels in"=w1464, "data"=TRUE) -> ("task out"=w1458:refnum<k21>)  [unwired: 11 in, 2 out]
      }
      frame ".0976" {
        # "No Resistor"
        # "30 ohm"
        # ".1 ohm"
        # "1 ohm"
        # "5 ohm"
        # "10 ohm"
        # "100 ohm"
        n722 = call-poly <vilib>:"DAQmx Create Virtual Channel.vi"("lines"=tag "Dev2/port0/line1") -> ("task out"=w1496:refnum<k21>)  [unwired: 13 in, 1 out]
        n723 = call-poly <vilib>:"DAQmx Create Virtual Channel.vi"("lines"=tag "Dev2/port0/line0") -> ("task out"=w1497:refnum<k21>)  [unwired: 13 in, 1 out]
        n724 = call-poly <vilib>:"DAQmx Create Virtual Channel.vi"("lines"=tag "Dev2/port0/line2") -> ("task out"=w1495:refnum<k21>)  [unwired: 13 in, 1 out]
        n725 = call-poly <vilib>:"DAQmx Create Virtual Channel.vi"("lines"=tag "Dev2/port0/line3") -> ("task out"=w1494:refnum<k21>)  [unwired: 13 in, 1 out]
        n726 = call-poly <vilib>:"DAQmx Create Virtual Channel.vi"("lines"=tag "Dev2/port0/line4") -> ("task out"=w1493:refnum<k21>)  [unwired: 13 in, 1 out]
        n727 = call-poly <vilib>:"DAQmx Create Virtual Channel.vi"("lines"=tag "Dev2/port0/line6") -> ("task out"=w1485:refnum<k21>)  [unwired: 13 in, 1 out]
        n728 = call-poly <vilib>:"DAQmx Create Virtual Channel.vi"("lines"=tag "Dev2/port0/line5") -> ("task out"=w1492:refnum<k21>)  [unwired: 13 in, 1 out]
        n729 = call-poly <vilib>:"DAQmx Write.vi"("task/channels in"=w1496, "data"=FALSE) -> ("task out"=w1490:refnum<k21>)  [unwired: 11 in, 2 out]
        n730 = call-poly <vilib>:"DAQmx Write.vi"("task/channels in"=w1495, "data"=FALSE) -> ("task out"=w1489:refnum<k21>)  [unwired: 11 in, 2 out]
        n731 = call-poly <vilib>:"DAQmx Write.vi"("task/channels in"=w1497, "data"=FALSE) -> ("task out"=w1491:refnum<k21>)  [unwired: 11 in, 2 out]
        n732 = call-poly <vilib>:"DAQmx Write.vi"("task/channels in"=w1494, "data"=FALSE) -> ("task out"=w1488:refnum<k21>)  [unwired: 11 in, 2 out]
        n733 = call-poly <vilib>:"DAQmx Write.vi"("task/channels in"=w1493, "data"=FALSE) -> ("task out"=w1487:refnum<k21>)  [unwired: 11 in, 2 out]
        n734 = call-poly <vilib>:"DAQmx Write.vi"("task/channels in"=w1485, "data"=FALSE) -> ("task out"=w1482:refnum<k21>)  [unwired: 11 in, 2 out]
        n735 = call-poly <vilib>:"DAQmx Write.vi"("task/channels in"=w1492, "data"=TRUE) -> ("task out"=w1486:refnum<k21>)  [unwired: 11 in, 2 out]
      }
      frame ".0977" {
        # "No Resistor"
        # "30 ohm"
        # ".1 ohm"
        # "1 ohm"
        # "5 ohm"
        # "10 ohm"
        # "100 ohm"
        n736 = call-poly <vilib>:"DAQmx Create Virtual Channel.vi"("lines"=tag "Dev2/port0/line1") -> ("task out"=w1524:refnum<k21>)  [unwired: 13 in, 1 out]
        n737 = call-poly <vilib>:"DAQmx Create Virtual Channel.vi"("lines"=tag "Dev2/port0/line0") -> ("task out"=w1525:refnum<k21>)  [unwired: 13 in, 1 out]
        n738 = call-poly <vilib>:"DAQmx Create Virtual Channel.vi"("lines"=tag "Dev2/port0/line2") -> ("task out"=w1523:refnum<k21>)  [unwired: 13 in, 1 out]
        n739 = call-poly <vilib>:"DAQmx Create Virtual Channel.vi"("lines"=tag "Dev2/port0/line3") -> ("task out"=w1522:refnum<k21>)  [unwired: 13 in, 1 out]
        n740 = call-poly <vilib>:"DAQmx Create Virtual Channel.vi"("lines"=tag "Dev2/port0/line4") -> ("task out"=w1521:refnum<k21>)  [unwired: 13 in, 1 out]
        n741 = call-poly <vilib>:"DAQmx Create Virtual Channel.vi"("lines"=tag "Dev2/port0/line6") -> ("task out"=w1513:refnum<k21>)  [unwired: 13 in, 1 out]
        n742 = call-poly <vilib>:"DAQmx Create Virtual Channel.vi"("lines"=tag "Dev2/port0/line5") -> ("task out"=w1520:refnum<k21>)  [unwired: 13 in, 1 out]
        n743 = call-poly <vilib>:"DAQmx Write.vi"("task/channels in"=w1524, "data"=FALSE) -> ("task out"=w1518:refnum<k21>)  [unwired: 11 in, 2 out]
        n744 = call-poly <vilib>:"DAQmx Write.vi"("task/channels in"=w1523, "data"=FALSE) -> ("task out"=w1517:refnum<k21>)  [unwired: 11 in, 2 out]
        n745 = call-poly <vilib>:"DAQmx Write.vi"("task/channels in"=w1525, "data"=FALSE) -> ("task out"=w1519:refnum<k21>)  [unwired: 11 in, 2 out]
        n746 = call-poly <vilib>:"DAQmx Write.vi"("task/channels in"=w1522, "data"=FALSE) -> ("task out"=w1516:refnum<k21>)  [unwired: 11 in, 2 out]
        n747 = call-poly <vilib>:"DAQmx Write.vi"("task/channels in"=w1521, "data"=FALSE) -> ("task out"=w1515:refnum<k21>)  [unwired: 11 in, 2 out]
        n748 = call-poly <vilib>:"DAQmx Write.vi"("task/channels in"=w1513, "data"=FALSE) -> ("task out"=w1510:refnum<k21>)  [unwired: 11 in, 2 out]
        n749 = call-poly <vilib>:"DAQmx Write.vi"("task/channels in"=w1520, "data"=TRUE) -> ("task out"=w1514:refnum<k21>)  [unwired: 11 in, 2 out]
      }
      frame ".0979" {
        # "No Resistor"
        # "30 ohm"
        # ".1 ohm"
        # "1 ohm"
        # "5 ohm"
        # "10 ohm"
        # "100 ohm"
        n750 = call-poly <vilib>:"DAQmx Create Virtual Channel.vi"("lines"=tag "Dev2/port0/line1") -> ("task out"=w1552:refnum<k21>)  [unwired: 13 in, 1 out]
        n751 = call-poly <vilib>:"DAQmx Create Virtual Channel.vi"("lines"=tag "Dev2/port0/line0") -> ("task out"=w1553:refnum<k21>)  [unwired: 13 in, 1 out]
        n752 = call-poly <vilib>:"DAQmx Create Virtual Channel.vi"("lines"=tag "Dev2/port0/line2") -> ("task out"=w1551:refnum<k21>)  [unwired: 13 in, 1 out]
        n753 = call-poly <vilib>:"DAQmx Create Virtual Channel.vi"("lines"=tag "Dev2/port0/line3") -> ("task out"=w1550:refnum<k21>)  [unwired: 13 in, 1 out]
        n754 = call-poly <vilib>:"DAQmx Create Virtual Channel.vi"("lines"=tag "Dev2/port0/line4") -> ("task out"=w1549:refnum<k21>)  [unwired: 13 in, 1 out]
        n755 = call-poly <vilib>:"DAQmx Create Virtual Channel.vi"("lines"=tag "Dev2/port0/line6") -> ("task out"=w1541:refnum<k21>)  [unwired: 13 in, 1 out]
        n756 = call-poly <vilib>:"DAQmx Create Virtual Channel.vi"("lines"=tag "Dev2/port0/line5") -> ("task out"=w1548:refnum<k21>)  [unwired: 13 in, 1 out]
        n757 = call-poly <vilib>:"DAQmx Write.vi"("task/channels in"=w1552, "data"=FALSE) -> ("task out"=w1546:refnum<k21>)  [unwired: 11 in, 2 out]
        n758 = call-poly <vilib>:"DAQmx Write.vi"("task/channels in"=w1551, "data"=FALSE) -> ("task out"=w1545:refnum<k21>)  [unwired: 11 in, 2 out]
        n759 = call-poly <vilib>:"DAQmx Write.vi"("task/channels in"=w1553, "data"=FALSE) -> ("task out"=w1547:refnum<k21>)  [unwired: 11 in, 2 out]
        n760 = call-poly <vilib>:"DAQmx Write.vi"("task/channels in"=w1550, "data"=FALSE) -> ("task out"=w1544:refnum<k21>)  [unwired: 11 in, 2 out]
        n761 = call-poly <vilib>:"DAQmx Write.vi"("task/channels in"=w1549, "data"=FALSE) -> ("task out"=w1543:refnum<k21>)  [unwired: 11 in, 2 out]
        n762 = call-poly <vilib>:"DAQmx Write.vi"("task/channels in"=w1541, "data"=FALSE) -> ("task out"=w1538:refnum<k21>)  [unwired: 11 in, 2 out]
        n763 = call-poly <vilib>:"DAQmx Write.vi"("task/channels in"=w1548, "data"=TRUE) -> ("task out"=w1542:refnum<k21>)  [unwired: 11 in, 2 out]
      }
      frame ".098" {
        # "No Resistor"
        # "30 ohm"
        # ".1 ohm"
        # "1 ohm"
        # "5 ohm"
        # "10 ohm"
        # "100 ohm"
        n764 = call-poly <vilib>:"DAQmx Create Virtual Channel.vi"("lines"=tag "Dev2/port0/line1") -> ("task out"=w1580:refnum<k21>)  [unwired: 13 in, 1 out]
        n765 = call-poly <vilib>:"DAQmx Create Virtual Channel.vi"("lines"=tag "Dev2/port0/line0") -> ("task out"=w1581:refnum<k21>)  [unwired: 13 in, 1 out]
        n766 = call-poly <vilib>:"DAQmx Create Virtual Channel.vi"("lines"=tag "Dev2/port0/line2") -> ("task out"=w1579:refnum<k21>)  [unwired: 13 in, 1 out]
        n767 = call-poly <vilib>:"DAQmx Create Virtual Channel.vi"("lines"=tag "Dev2/port0/line3") -> ("task out"=w1578:refnum<k21>)  [unwired: 13 in, 1 out]
        n768 = call-poly <vilib>:"DAQmx Create Virtual Channel.vi"("lines"=tag "Dev2/port0/line4") -> ("task out"=w1577:refnum<k21>)  [unwired: 13 in, 1 out]
        n769 = call-poly <vilib>:"DAQmx Create Virtual Channel.vi"("lines"=tag "Dev2/port0/line6") -> ("task out"=w1569:refnum<k21>)  [unwired: 13 in, 1 out]
        n770 = call-poly <vilib>:"DAQmx Create Virtual Channel.vi"("lines"=tag "Dev2/port0/line5") -> ("task out"=w1576:refnum<k21>)  [unwired: 13 in, 1 out]
        n771 = call-poly <vilib>:"DAQmx Write.vi"("task/channels in"=w1580, "data"=FALSE) -> ("task out"=w1574:refnum<k21>)  [unwired: 11 in, 2 out]
        n772 = call-poly <vilib>:"DAQmx Write.vi"("task/channels in"=w1579, "data"=FALSE) -> ("task out"=w1573:refnum<k21>)  [unwired: 11 in, 2 out]
        n773 = call-poly <vilib>:"DAQmx Write.vi"("task/channels in"=w1581, "data"=FALSE) -> ("task out"=w1575:refnum<k21>)  [unwired: 11 in, 2 out]
        n774 = call-poly <vilib>:"DAQmx Write.vi"("task/channels in"=w1578, "data"=FALSE) -> ("task out"=w1572:refnum<k21>)  [unwired: 11 in, 2 out]
        n775 = call-poly <vilib>:"DAQmx Write.vi"("task/channels in"=w1577, "data"=FALSE) -> ("task out"=w1571:refnum<k21>)  [unwired: 11 in, 2 out]
        n776 = call-poly <vilib>:"DAQmx Write.vi"("task/channels in"=w1569, "data"=FALSE) -> ("task out"=w1566:refnum<k21>)  [unwired: 11 in, 2 out]
        n777 = call-poly <vilib>:"DAQmx Write.vi"("task/channels in"=w1576, "data"=TRUE) -> ("task out"=w1570:refnum<k21>)  [unwired: 11 in, 2 out]
      }
      frame ".0986" {
        # "No Resistor"
        # "30 ohm"
        # ".1 ohm"
        # "1 ohm"
        # "5 ohm"
        # "10 ohm"
        # "100 ohm"
        n778 = call-poly <vilib>:"DAQmx Create Virtual Channel.vi"("lines"=tag "Dev2/port0/line1") -> ("task out"=w1608:refnum<k21>)  [unwired: 13 in, 1 out]
        n779 = call-poly <vilib>:"DAQmx Create Virtual Channel.vi"("lines"=tag "Dev2/port0/line0") -> ("task out"=w1609:refnum<k21>)  [unwired: 13 in, 1 out]
        n780 = call-poly <vilib>:"DAQmx Create Virtual Channel.vi"("lines"=tag "Dev2/port0/line2") -> ("task out"=w1607:refnum<k21>)  [unwired: 13 in, 1 out]
        n781 = call-poly <vilib>:"DAQmx Create Virtual Channel.vi"("lines"=tag "Dev2/port0/line3") -> ("task out"=w1606:refnum<k21>)  [unwired: 13 in, 1 out]
        n782 = call-poly <vilib>:"DAQmx Create Virtual Channel.vi"("lines"=tag "Dev2/port0/line4") -> ("task out"=w1605:refnum<k21>)  [unwired: 13 in, 1 out]
        n783 = call-poly <vilib>:"DAQmx Create Virtual Channel.vi"("lines"=tag "Dev2/port0/line6") -> ("task out"=w1597:refnum<k21>)  [unwired: 13 in, 1 out]
        n784 = call-poly <vilib>:"DAQmx Create Virtual Channel.vi"("lines"=tag "Dev2/port0/line5") -> ("task out"=w1604:refnum<k21>)  [unwired: 13 in, 1 out]
        n785 = call-poly <vilib>:"DAQmx Write.vi"("task/channels in"=w1608, "data"=FALSE) -> ("task out"=w1602:refnum<k21>)  [unwired: 11 in, 2 out]
        n786 = call-poly <vilib>:"DAQmx Write.vi"("task/channels in"=w1607, "data"=FALSE) -> ("task out"=w1601:refnum<k21>)  [unwired: 11 in, 2 out]
        n787 = call-poly <vilib>:"DAQmx Write.vi"("task/channels in"=w1609, "data"=FALSE) -> ("task out"=w1603:refnum<k21>)  [unwired: 11 in, 2 out]
        n788 = call-poly <vilib>:"DAQmx Write.vi"("task/channels in"=w1606, "data"=FALSE) -> ("task out"=w1600:refnum<k21>)  [unwired: 11 in, 2 out]
        n789 = call-poly <vilib>:"DAQmx Write.vi"("task/channels in"=w1605, "data"=FALSE) -> ("task out"=w1599:refnum<k21>)  [unwired: 11 in, 2 out]
        n790 = call-poly <vilib>:"DAQmx Write.vi"("task/channels in"=w1597, "data"=FALSE) -> ("task out"=w1594:refnum<k21>)  [unwired: 11 in, 2 out]
        n791 = call-poly <vilib>:"DAQmx Write.vi"("task/channels in"=w1604, "data"=TRUE) -> ("task out"=w1598:refnum<k21>)  [unwired: 11 in, 2 out]
      }
      frame ".0987" {
        # "No Resistor"
        # "30 ohm"
        # ".1 ohm"
        # "1 ohm"
        # "5 ohm"
        # "10 ohm"
        # "100 ohm"
        n792 = call-poly <vilib>:"DAQmx Create Virtual Channel.vi"("lines"=tag "Dev2/port0/line1") -> ("task out"=w1636:refnum<k21>)  [unwired: 13 in, 1 out]
        n793 = call-poly <vilib>:"DAQmx Create Virtual Channel.vi"("lines"=tag "Dev2/port0/line0") -> ("task out"=w1637:refnum<k21>)  [unwired: 13 in, 1 out]
        n794 = call-poly <vilib>:"DAQmx Create Virtual Channel.vi"("lines"=tag "Dev2/port0/line2") -> ("task out"=w1635:refnum<k21>)  [unwired: 13 in, 1 out]
        n795 = call-poly <vilib>:"DAQmx Create Virtual Channel.vi"("lines"=tag "Dev2/port0/line3") -> ("task out"=w1634:refnum<k21>)  [unwired: 13 in, 1 out]
        n796 = call-poly <vilib>:"DAQmx Create Virtual Channel.vi"("lines"=tag "Dev2/port0/line4") -> ("task out"=w1633:refnum<k21>)  [unwired: 13 in, 1 out]
        n797 = call-poly <vilib>:"DAQmx Create Virtual Channel.vi"("lines"=tag "Dev2/port0/line6") -> ("task out"=w1625:refnum<k21>)  [unwired: 13 in, 1 out]
        n798 = call-poly <vilib>:"DAQmx Create Virtual Channel.vi"("lines"=tag "Dev2/port0/line5") -> ("task out"=w1632:refnum<k21>)  [unwired: 13 in, 1 out]
        n799 = call-poly <vilib>:"DAQmx Write.vi"("task/channels in"=w1636, "data"=FALSE) -> ("task out"=w1630:refnum<k21>)  [unwired: 11 in, 2 out]
        n800 = call-poly <vilib>:"DAQmx Write.vi"("task/channels in"=w1635, "data"=FALSE) -> ("task out"=w1629:refnum<k21>)  [unwired: 11 in, 2 out]
        n801 = call-poly <vilib>:"DAQmx Write.vi"("task/channels in"=w1637, "data"=FALSE) -> ("task out"=w1631:refnum<k21>)  [unwired: 11 in, 2 out]
        n802 = call-poly <vilib>:"DAQmx Write.vi"("task/channels in"=w1634, "data"=FALSE) -> ("task out"=w1628:refnum<k21>)  [unwired: 11 in, 2 out]
        n803 = call-poly <vilib>:"DAQmx Write.vi"("task/channels in"=w1633, "data"=FALSE) -> ("task out"=w1627:refnum<k21>)  [unwired: 11 in, 2 out]
        n804 = call-poly <vilib>:"DAQmx Write.vi"("task/channels in"=w1625, "data"=FALSE) -> ("task out"=w1622:refnum<k21>)  [unwired: 11 in, 2 out]
        n805 = call-poly <vilib>:"DAQmx Write.vi"("task/channels in"=w1632, "data"=TRUE) -> ("task out"=w1626:refnum<k21>)  [unwired: 11 in, 2 out]
      }
      frame ".0989" {
        # "No Resistor"
        # "30 ohm"
        # ".1 ohm"
        # "1 ohm"
        # "5 ohm"
        # "10 ohm"
        # "100 ohm"
        n806 = call-poly <vilib>:"DAQmx Create Virtual Channel.vi"("lines"=tag "Dev2/port0/line1") -> ("task out"=w1664:refnum<k21>)  [unwired: 13 in, 1 out]
        n807 = call-poly <vilib>:"DAQmx Create Virtual Channel.vi"("lines"=tag "Dev2/port0/line0") -> ("task out"=w1665:refnum<k21>)  [unwired: 13 in, 1 out]
        n808 = call-poly <vilib>:"DAQmx Create Virtual Channel.vi"("lines"=tag "Dev2/port0/line2") -> ("task out"=w1663:refnum<k21>)  [unwired: 13 in, 1 out]
        n809 = call-poly <vilib>:"DAQmx Create Virtual Channel.vi"("lines"=tag "Dev2/port0/line3") -> ("task out"=w1662:refnum<k21>)  [unwired: 13 in, 1 out]
        n810 = call-poly <vilib>:"DAQmx Create Virtual Channel.vi"("lines"=tag "Dev2/port0/line4") -> ("task out"=w1661:refnum<k21>)  [unwired: 13 in, 1 out]
        n811 = call-poly <vilib>:"DAQmx Create Virtual Channel.vi"("lines"=tag "Dev2/port0/line6") -> ("task out"=w1653:refnum<k21>)  [unwired: 13 in, 1 out]
        n812 = call-poly <vilib>:"DAQmx Create Virtual Channel.vi"("lines"=tag "Dev2/port0/line5") -> ("task out"=w1660:refnum<k21>)  [unwired: 13 in, 1 out]
        n813 = call-poly <vilib>:"DAQmx Write.vi"("task/channels in"=w1664, "data"=FALSE) -> ("task out"=w1658:refnum<k21>)  [unwired: 11 in, 2 out]
        n814 = call-poly <vilib>:"DAQmx Write.vi"("task/channels in"=w1663, "data"=FALSE) -> ("task out"=w1657:refnum<k21>)  [unwired: 11 in, 2 out]
        n815 = call-poly <vilib>:"DAQmx Write.vi"("task/channels in"=w1665, "data"=FALSE) -> ("task out"=w1659:refnum<k21>)  [unwired: 11 in, 2 out]
        n816 = call-poly <vilib>:"DAQmx Write.vi"("task/channels in"=w1662, "data"=FALSE) -> ("task out"=w1656:refnum<k21>)  [unwired: 11 in, 2 out]
        n817 = call-poly <vilib>:"DAQmx Write.vi"("task/channels in"=w1661, "data"=FALSE) -> ("task out"=w1655:refnum<k21>)  [unwired: 11 in, 2 out]
        n818 = call-poly <vilib>:"DAQmx Write.vi"("task/channels in"=w1653, "data"=FALSE) -> ("task out"=w1650:refnum<k21>)  [unwired: 11 in, 2 out]
        n819 = call-poly <vilib>:"DAQmx Write.vi"("task/channels in"=w1660, "data"=TRUE) -> ("task out"=w1654:refnum<k21>)  [unwired: 11 in, 2 out]
      }
      frame ".099" {
        # "No Resistor"
        # "30 ohm"
        # ".1 ohm"
        # "1 ohm"
        # "5 ohm"
        # "10 ohm"
        # "100 ohm"
        n820 = call-poly <vilib>:"DAQmx Create Virtual Channel.vi"("lines"=tag "Dev2/port0/line1") -> ("task out"=w1692:refnum<k21>)  [unwired: 13 in, 1 out]
        n821 = call-poly <vilib>:"DAQmx Create Virtual Channel.vi"("lines"=tag "Dev2/port0/line0") -> ("task out"=w1693:refnum<k21>)  [unwired: 13 in, 1 out]
        n822 = call-poly <vilib>:"DAQmx Create Virtual Channel.vi"("lines"=tag "Dev2/port0/line2") -> ("task out"=w1691:refnum<k21>)  [unwired: 13 in, 1 out]
        n823 = call-poly <vilib>:"DAQmx Create Virtual Channel.vi"("lines"=tag "Dev2/port0/line3") -> ("task out"=w1690:refnum<k21>)  [unwired: 13 in, 1 out]
        n824 = call-poly <vilib>:"DAQmx Create Virtual Channel.vi"("lines"=tag "Dev2/port0/line4") -> ("task out"=w1689:refnum<k21>)  [unwired: 13 in, 1 out]
        n825 = call-poly <vilib>:"DAQmx Create Virtual Channel.vi"("lines"=tag "Dev2/port0/line6") -> ("task out"=w1681:refnum<k21>)  [unwired: 13 in, 1 out]
        n826 = call-poly <vilib>:"DAQmx Create Virtual Channel.vi"("lines"=tag "Dev2/port0/line5") -> ("task out"=w1688:refnum<k21>)  [unwired: 13 in, 1 out]
        n827 = call-poly <vilib>:"DAQmx Write.vi"("task/channels in"=w1692, "data"=FALSE) -> ("task out"=w1686:refnum<k21>)  [unwired: 11 in, 2 out]
        n828 = call-poly <vilib>:"DAQmx Write.vi"("task/channels in"=w1691, "data"=FALSE) -> ("task out"=w1685:refnum<k21>)  [unwired: 11 in, 2 out]
        n829 = call-poly <vilib>:"DAQmx Write.vi"("task/channels in"=w1693, "data"=FALSE) -> ("task out"=w1687:refnum<k21>)  [unwired: 11 in, 2 out]
        n830 = call-poly <vilib>:"DAQmx Write.vi"("task/channels in"=w1690, "data"=FALSE) -> ("task out"=w1684:refnum<k21>)  [unwired: 11 in, 2 out]
        n831 = call-poly <vilib>:"DAQmx Write.vi"("task/channels in"=w1689, "data"=FALSE) -> ("task out"=w1683:refnum<k21>)  [unwired: 11 in, 2 out]
        n832 = call-poly <vilib>:"DAQmx Write.vi"("task/channels in"=w1681, "data"=FALSE) -> ("task out"=w1678:refnum<k21>)  [unwired: 11 in, 2 out]
        n833 = call-poly <vilib>:"DAQmx Write.vi"("task/channels in"=w1688, "data"=TRUE) -> ("task out"=w1682:refnum<k21>)  [unwired: 11 in, 2 out]
      }
      frame ".0996" {
        # "No Resistor"
        # "30 ohm"
        # ".1 ohm"
        # "1 ohm"
        # "5 ohm"
        # "10 ohm"
        # "100 ohm"
        n834 = call-poly <vilib>:"DAQmx Create Virtual Channel.vi"("lines"=tag "Dev2/port0/line1") -> ("task out"=w1720:refnum<k21>)  [unwired: 13 in, 1 out]
        n835 = call-poly <vilib>:"DAQmx Create Virtual Channel.vi"("lines"=tag "Dev2/port0/line0") -> ("task out"=w1721:refnum<k21>)  [unwired: 13 in, 1 out]
        n836 = call-poly <vilib>:"DAQmx Create Virtual Channel.vi"("lines"=tag "Dev2/port0/line2") -> ("task out"=w1719:refnum<k21>)  [unwired: 13 in, 1 out]
        n837 = call-poly <vilib>:"DAQmx Create Virtual Channel.vi"("lines"=tag "Dev2/port0/line3") -> ("task out"=w1718:refnum<k21>)  [unwired: 13 in, 1 out]
        n838 = call-poly <vilib>:"DAQmx Create Virtual Channel.vi"("lines"=tag "Dev2/port0/line4") -> ("task out"=w1717:refnum<k21>)  [unwired: 13 in, 1 out]
        n839 = call-poly <vilib>:"DAQmx Create Virtual Channel.vi"("lines"=tag "Dev2/port0/line6") -> ("task out"=w1709:refnum<k21>)  [unwired: 13 in, 1 out]
        n840 = call-poly <vilib>:"DAQmx Create Virtual Channel.vi"("lines"=tag "Dev2/port0/line5") -> ("task out"=w1716:refnum<k21>)  [unwired: 13 in, 1 out]
        n841 = call-poly <vilib>:"DAQmx Write.vi"("task/channels in"=w1720, "data"=FALSE) -> ("task out"=w1714:refnum<k21>)  [unwired: 11 in, 2 out]
        n842 = call-poly <vilib>:"DAQmx Write.vi"("task/channels in"=w1719, "data"=FALSE) -> ("task out"=w1713:refnum<k21>)  [unwired: 11 in, 2 out]
        n843 = call-poly <vilib>:"DAQmx Write.vi"("task/channels in"=w1721, "data"=FALSE) -> ("task out"=w1715:refnum<k21>)  [unwired: 11 in, 2 out]
        n844 = call-poly <vilib>:"DAQmx Write.vi"("task/channels in"=w1718, "data"=FALSE) -> ("task out"=w1712:refnum<k21>)  [unwired: 11 in, 2 out]
        n845 = call-poly <vilib>:"DAQmx Write.vi"("task/channels in"=w1717, "data"=FALSE) -> ("task out"=w1711:refnum<k21>)  [unwired: 11 in, 2 out]
        n846 = call-poly <vilib>:"DAQmx Write.vi"("task/channels in"=w1709, "data"=FALSE) -> ("task out"=w1706:refnum<k21>)  [unwired: 11 in, 2 out]
        n847 = call-poly <vilib>:"DAQmx Write.vi"("task/channels in"=w1716, "data"=TRUE) -> ("task out"=w1710:refnum<k21>)  [unwired: 11 in, 2 out]
      }
      frame ".0997" {
        # "No Resistor"
        # "30 ohm"
        # ".1 ohm"
        # "1 ohm"
        # "5 ohm"
        # "10 ohm"
        # "100 ohm"
        n848 = call-poly <vilib>:"DAQmx Create Virtual Channel.vi"("lines"=tag "Dev2/port0/line1") -> ("task out"=w1748:refnum<k21>)  [unwired: 13 in, 1 out]
        n849 = call-poly <vilib>:"DAQmx Create Virtual Channel.vi"("lines"=tag "Dev2/port0/line0") -> ("task out"=w1749:refnum<k21>)  [unwired: 13 in, 1 out]
        n850 = call-poly <vilib>:"DAQmx Create Virtual Channel.vi"("lines"=tag "Dev2/port0/line2") -> ("task out"=w1747:refnum<k21>)  [unwired: 13 in, 1 out]
        n851 = call-poly <vilib>:"DAQmx Create Virtual Channel.vi"("lines"=tag "Dev2/port0/line3") -> ("task out"=w1746:refnum<k21>)  [unwired: 13 in, 1 out]
        n852 = call-poly <vilib>:"DAQmx Create Virtual Channel.vi"("lines"=tag "Dev2/port0/line4") -> ("task out"=w1745:refnum<k21>)  [unwired: 13 in, 1 out]
        n853 = call-poly <vilib>:"DAQmx Create Virtual Channel.vi"("lines"=tag "Dev2/port0/line6") -> ("task out"=w1737:refnum<k21>)  [unwired: 13 in, 1 out]
        n854 = call-poly <vilib>:"DAQmx Create Virtual Channel.vi"("lines"=tag "Dev2/port0/line5") -> ("task out"=w1744:refnum<k21>)  [unwired: 13 in, 1 out]
        n855 = call-poly <vilib>:"DAQmx Write.vi"("task/channels in"=w1748, "data"=FALSE) -> ("task out"=w1742:refnum<k21>)  [unwired: 11 in, 2 out]
        n856 = call-poly <vilib>:"DAQmx Write.vi"("task/channels in"=w1747, "data"=FALSE) -> ("task out"=w1741:refnum<k21>)  [unwired: 11 in, 2 out]
        n857 = call-poly <vilib>:"DAQmx Write.vi"("task/channels in"=w1749, "data"=FALSE) -> ("task out"=w1743:refnum<k21>)  [unwired: 11 in, 2 out]
        n858 = call-poly <vilib>:"DAQmx Write.vi"("task/channels in"=w1746, "data"=FALSE) -> ("task out"=w1740:refnum<k21>)  [unwired: 11 in, 2 out]
        n859 = call-poly <vilib>:"DAQmx Write.vi"("task/channels in"=w1745, "data"=FALSE) -> ("task out"=w1739:refnum<k21>)  [unwired: 11 in, 2 out]
        n860 = call-poly <vilib>:"DAQmx Write.vi"("task/channels in"=w1737, "data"=FALSE) -> ("task out"=w1734:refnum<k21>)  [unwired: 11 in, 2 out]
        n861 = call-poly <vilib>:"DAQmx Write.vi"("task/channels in"=w1744, "data"=TRUE) -> ("task out"=w1738:refnum<k21>)  [unwired: 11 in, 2 out]
      }
      frame ".0999" {
        # "No Resistor"
        # "30 ohm"
        # ".1 ohm"
        # "1 ohm"
        # "5 ohm"
        # "10 ohm"
        # "100 ohm"
        n862 = call-poly <vilib>:"DAQmx Create Virtual Channel.vi"("lines"=tag "Dev2/port0/line1") -> ("task out"=w1776:refnum<k21>)  [unwired: 13 in, 1 out]
        n863 = call-poly <vilib>:"DAQmx Create Virtual Channel.vi"("lines"=tag "Dev2/port0/line0") -> ("task out"=w1777:refnum<k21>)  [unwired: 13 in, 1 out]
        n864 = call-poly <vilib>:"DAQmx Create Virtual Channel.vi"("lines"=tag "Dev2/port0/line2") -> ("task out"=w1775:refnum<k21>)  [unwired: 13 in, 1 out]
        n865 = call-poly <vilib>:"DAQmx Create Virtual Channel.vi"("lines"=tag "Dev2/port0/line3") -> ("task out"=w1774:refnum<k21>)  [unwired: 13 in, 1 out]
        n866 = call-poly <vilib>:"DAQmx Create Virtual Channel.vi"("lines"=tag "Dev2/port0/line4") -> ("task out"=w1773:refnum<k21>)  [unwired: 13 in, 1 out]
        n867 = call-poly <vilib>:"DAQmx Create Virtual Channel.vi"("lines"=tag "Dev2/port0/line6") -> ("task out"=w1765:refnum<k21>)  [unwired: 13 in, 1 out]
        n868 = call-poly <vilib>:"DAQmx Create Virtual Channel.vi"("lines"=tag "Dev2/port0/line5") -> ("task out"=w1772:refnum<k21>)  [unwired: 13 in, 1 out]
        n869 = call-poly <vilib>:"DAQmx Write.vi"("task/channels in"=w1776, "data"=FALSE) -> ("task out"=w1770:refnum<k21>)  [unwired: 11 in, 2 out]
        n870 = call-poly <vilib>:"DAQmx Write.vi"("task/channels in"=w1775, "data"=FALSE) -> ("task out"=w1769:refnum<k21>)  [unwired: 11 in, 2 out]
        n871 = call-poly <vilib>:"DAQmx Write.vi"("task/channels in"=w1777, "data"=FALSE) -> ("task out"=w1771:refnum<k21>)  [unwired: 11 in, 2 out]
        n872 = call-poly <vilib>:"DAQmx Write.vi"("task/channels in"=w1774, "data"=FALSE) -> ("task out"=w1768:refnum<k21>)  [unwired: 11 in, 2 out]
        n873 = call-poly <vilib>:"DAQmx Write.vi"("task/channels in"=w1773, "data"=FALSE) -> ("task out"=w1767:refnum<k21>)  [unwired: 11 in, 2 out]
        n874 = call-poly <vilib>:"DAQmx Write.vi"("task/channels in"=w1765, "data"=FALSE) -> ("task out"=w1762:refnum<k21>)  [unwired: 11 in, 2 out]
        n875 = call-poly <vilib>:"DAQmx Write.vi"("task/channels in"=w1772, "data"=TRUE) -> ("task out"=w1766:refnum<k21>)  [unwired: 11 in, 2 out]
      }
    }
    n876 = call "Elapsed Time"("Time Target (s)"=w36) -> ("Elapsed Time (s)"=→"resis bank Numeric":dbl, "Time has Elapsed"=w37:bool)  [unwired: 11 in, 6 out]
    n877 = call-poly <vilib>:"DAQmx Create Virtual Channel.vi"("lines"=tag "Dev2/port0/line7") -> ("task out"=w48:refnum<k21>)  [unwired: 13 in, 1 out]
    n878 = call-poly <vilib>:"DAQmx Create Virtual Channel.vi"("lines"=tag "Dev2/port2/line6") -> ("task out"=w51:refnum<k21>)  [unwired: 13 in, 1 out]
    n879 = call-poly <vilib>:"DAQmx Write.vi"("task/channels in"=w51, "data"=TRUE) -> ()  [unwired: 11 in, 3 out]
    n880 = call-poly <vilib>:"DAQmx Write.vi"("task/channels in"=w48, "data"=TRUE) -> ("task out"=w47:refnum<k21>)  [unwired: 11 in, 2 out]
  }
  n881 = while {
    tunnel: w5 -> [_]
    tunnel: w6 -> [w1795]
    tunnel: w4 -> [w1794]
    tunnel: [w1790] -> w2
    stop <- w1793 stop-if-true
    n882 = call "Elapsed Time2"("Time Target (s)"=w1794) -> ("Elapsed Time (s)"=→"SB Elapsed Time (s)":dbl, "Time has Elapsed"=w1793:bool)  [unwired: 11 in, 6 out]
    n883 = call-poly <vilib>:"DAQmx Write.vi"("task/channels in"=w1795, "frequency"="frequency", "duty cycle"=0.5) -> ("task out"=w1790:refnum<k21>)  [unwired: 2 in, 10 out]
  }
  n884 = call <vilib>:"DAQmx Stop Task.vi"("task/channels in"=w2) -> ("task out"=w3:refnum<k21>)  [unwired: 13 in, 1 out]
  n885 = call <vilib>:"DAQmx Clear Task.vi"("task in"=w3) -> ()  [unwired: 14 in, 1 out]
  n886 = call-poly <vilib>:"DAQmx Write.vi"("task/channels in"=w12, "data"=FALSE) -> ("task out"=w24:refnum<k21>)  [unwired: 11 in, 2 out]
  n887 = call-poly <vilib>:"DAQmx Write.vi"("task/channels in"=w19, "data"=FALSE) -> ("task out"=w23:refnum<k21>)  [unwired: 11 in, 2 out]
  n888 = call-poly <vilib>:"DAQmx Write.vi"("task/channels in"=w17, "data"=FALSE) -> ("task out"=w35:refnum<k21>)  [unwired: 11 in, 2 out]
  n889 = call-poly <vilib>:"DAQmx Write.vi"("task/channels in"=w16, "data"=FALSE) -> ("task out"=w32:refnum<k21>)  [unwired: 11 in, 2 out]
  n890 = call-poly <vilib>:"DAQmx Write.vi"("task/channels in"=w15, "data"=FALSE) -> ("task out"=w31:refnum<k21>)  [unwired: 11 in, 2 out]
  n891 = call-poly <vilib>:"DAQmx Write.vi"("task/channels in"=w18, "data"=FALSE) -> ("task out"=w21:refnum<k21>)  [unwired: 11 in, 2 out]
  n892 = call-poly <vilib>:"DAQmx Write.vi"("task/channels in"=w14, "data"=FALSE) -> ("task out"=w28:refnum<k21>)  [unwired: 11 in, 2 out]
  n893 = call-poly <vilib>:"DAQmx Write.vi"("task/channels in"=w13, "data"=FALSE) -> ("task out"=w26:refnum<k21>)  [unwired: 11 in, 2 out]
  n894 = call <vilib>:"DAQmx Clear Task.vi"("task in"=w23) -> ()  [unwired: 14 in, 1 out]
  n895 = call <vilib>:"DAQmx Clear Task.vi"("task in"=w35) -> ()  [unwired: 14 in, 1 out]
  n896 = call <vilib>:"DAQmx Clear Task.vi"("task in"=w32) -> ()  [unwired: 14 in, 1 out]
  n897 = call <vilib>:"DAQmx Clear Task.vi"("task in"=w24) -> ()  [unwired: 14 in, 1 out]
  n898 = call <vilib>:"DAQmx Clear Task.vi"("task in"=w31) -> ()  [unwired: 14 in, 1 out]
  n899 = call <vilib>:"DAQmx Clear Task.vi"("task in"=w28) -> ()  [unwired: 14 in, 1 out]
  n900 = call <vilib>:"DAQmx Clear Task.vi"("task in"=w26) -> ()  [unwired: 14 in, 1 out]
  n901 = call <vilib>:"DAQmx Clear Task.vi"("task in"=w21) -> ()  [unwired: 14 in, 1 out]
